vi "参数生成器.vi"() -> ()   [LabVIEW 2013]
uses:
  <vilib>/Utility/config.llb/Write Key (String).vi
  <vilib>/Utility/config.llb/Read Key (String).vi
  <vilib>/Utility/file.llb/Read From Spreadsheet File (string).vi
  <vilib>/Utility/config.llb/Write Key (Path).vi
  <vilib>/Utility/config.llb/NI_LVConfig.lvlib
panel:
  in  "均衡参数设置":bool
  in  "error in":errorcluster caption="错误输入"
  out "临时从板数据":string[](array[string])
  in  "自动记录":bool
  in  "通道电压清零":bool
  in  "自动计算通道电压":bool
  out "均衡参数":T1={"充电结束电压(90%)"=3.0, "充电结束电压(91%)"=3.0, "充电结束电压(92%)"=3.0, "充电结束电压(93%)"=3.0, "充电结束电压(94%)"=3.0, "均衡计算-电压高阀值1级"=3.0, "均衡计算-电压高阀值2级"=3.0, "均衡计算-电压低阀值1级"=3.0, "均衡计算-电压低阀值2级"=3.0, "均衡计算-最低电压阀值"=3.0, "均衡停止-最低电压阀值"=3.0, "均衡计算-电压极差阀值"=3.0, "充电结束电压(95%)"=3.0, "充电结束电压(96%)"=3.0, "充电结束电压(97%)"=3.0, "充电结束电压(98%)"=3.0, "充电结束电压(99%)"=3.0, "充电结束电压(100%)"=3.0} {"充电结束电压(100%)" min=0 max=5 format="%#.4f"; "充电结束电压(99%)" min=0 max=5 format="%#.4f"; "充电结束电压(98%)" min=0 max=5 format="%#.4f"; "充电结束电压(97%)" min=0 max=5 format="%#.4f"; "充电结束电压(96%)" min=0 max=5 format="%#.4f"; "充电结束电压(95%)" min=0 max=5 format="%#.4f"; "均衡计算-电压极差阀值" min=0 max=5 format="%#.4f"; "均衡停止-最低电压阀值" min=0 max=5 format="%#.4f"; "均衡计算-最低电压阀值" min=0 max=5 format="%#.4f"; "均衡计算-电压低阀值2级" min=0 max=5 format="%#.4f"; "充电结束电压(94%)" min=0 max=5 format="%#.4f"; "充电结束电压(93%)" min=0 max=5 format="%#.4f"; "均衡计算-电压低阀值1级" min=0 max=5 format="%#.4f"; "均衡计算-电压高阀值1级" min=0 max=5 format="%#.4f"; "均衡计算-电压高阀值2级" min=0 max=5 format="%#.4f"; "充电结束电压(92%)" min=0 max=5 format="%#.4f"; "充电结束电压(91%)" min=0 max=5 format="%#.4f"; "充电结束电压(90%)" min=0 max=5 format="%#.4f"}
  in  "布尔":bool
  in  "全部记录":bool
  in  "查看":bool
  in  "读从板信息":bool
  in  "字符串":string
  out "MD5 message-digest":string="c47cafb9475eca419ba2638971991389" caption="MD5信息摘要"
  out "从板表头":string[](array[string])=["从板板号", "电压个数", "电压起始值", "温度个数", "温度起始值", "第一个保险通道", "第一个保险位置", "第二个保险通道", "第二个保险位置", "第三个保险通道", "第三个保险位置", "第四个保险通道", "第四个保险位置", "第五个保险通道", "第五个保险位置", "第六个保险通道", "第六个保险位置", "第七个保险通道", "第七个保险位置", "第八个保险通道", "第八个保险位置", "第九个保险通道", "第九个保险位置", "第十个保险通道", "第十个保险位置", "第1通道电压个数", "第2通道电压个数", "第3通道电压个数", "第4通道电压个数", "第5通道电压个数", "第6通道电压个数", "第7通道电压个数", "第8通道电压个数", "第9通道电压个数", "第10通道电压个数", "第11通道电压个数", "第12通道电压个数", "第13通道电压个数", "第14通道电压个数", "第15通道电压个数", "第16通道电压个数", "第17通道电压个数", "第18通道电压个数", "第19通道电压个数", "第20通道电压个数", "风机开启温度", "风机关闭温度", "加热开启温度", "加热关闭温度", "风机开启温差", "风机关闭温差", "加热关闭温差", "电压过高一级", "电压过低一级", "温度过高一级", "温度过低一级", "电压不均衡一级", "温度不均衡一级", "SOC过低一级", "电压过高二级", "电压过低二级", "温度过高二级", "温度过低二级", "电压不均衡二级", "温度不均衡二级", "SOC过低二级", "电压过高三级", "电压过低三级", "温度过高三级", "温度过低三级", "电压不均衡三级", "温度不均衡三级", "SOC过低三级", "均衡计算-电压高阀值1级", "均衡计算-电压高阀值2级", "均衡计算-电压低阀值1级", "均衡计算-电压低阀值2级", "均衡计算-最低电压阀值", "均衡停止-最低电压阀值", "均衡计算-电压极差阀值", "充电结束电压(90%)", "充电结束电压(91%)", "充电结束电压(92%)", "充电结束电压(93%)", "充电结束电压(94%)", "充电结束电压(95%)", "充电结束电压(96%)", "充电结束电压(97%)", "充电结束电压(98%)", "充电结束电压(99%)", "充电结束电压(100%)"]
  out "输出数组":string[][](array[string])=[["1", "2", "3", " ", " ", " ", " ", " ", " ", " ", " ", " ", " ", " ", " ", " ", " ", " ", " ", " ", " ", " ", " ", " ", " ", " ", " ", " ", " ", " "], ["10", "10", "10", " ", " ", " ", " ", " ", " ", " ", " ", " ", " ", " ", " ", " ", " ", " ", " ", " ", " ", " ", " ", " ", " ", " ", " ", " ", " ", " "], ["", "0", "0", " ", " ", " ", " ", " ", " ", " ", " ", " ", " ", " ", " ", " ", " ", " ", " ", " ", " ", " ", " ", " ", " ", " ", " ", " ", " ", " "], ["2", "2", "2", " ", " ", " ", " ", " ", " ", " ", " ", " ", " ", " ", " ", " ", " ", " ", " ", " ", " ", " ", " ", " ", " ", " ", " ", " ", " ", " "], ["", "0", "0", " ", " ", " ", " ", " ", " ", " ", " ", " ", " ", " ", " ", " ", " ", " ", " ", " ", " ", " ", " ", " ", " ", " ", " ", " ", " ", " "], [" ", " ", " ", " ", " ", " ", " ", " ", " ", " ", " ", " ", " ", " ", " ", " ", " ", " ", " ", " ", " ", " ", " ", " ", " ", " ", " ", " ", " ", " "], [" ", " ", " ", " ", " ", " ", " ", " ", " ", " ", " ", " ", " ", " ", " ", " ", " ", " ", " ", " ", " ", " ", " ", " ", " ", " ", " ", " ", " ", " "], [" ", " ", " ", " ", " ", " ", " ", " ", " ", " ", " ", " ", " ", " ", " ", " ", " ", " ", " ", " ", " ", " ", " ", " ", " ", " ", " ", " ", " ", " "], [" ", " ", " ", " ", " ", " ", " ", " ", " ", " ", " ", " ", " ", " ", " ", " ", " ", " ", " ", " ", " ", " ", " ", " ", " ", " ", " ", " ", " ", " "], [" ", " ", " ", " ", " ", " ", " ", " ", " ", " ", " ", " ", " ", " ", " ", " ", " ", " ", " ", " ", " ", " ", " ", " ", " ", " ", " ", " ", " ", " "], [" ", " ", " ", " ", " ", " ", " ", " ", " ", " ", " ", " ", " ", " ", " ", " ", " ", " ", " ", " ", " ", " ", " ", " ", " ", " ", " ", " ", " ", " "], [" ", " ", " ", " ", " ", " ", " ", " ", " ", " ", " ", " ", " ", " ", " ", " ", " ", " ", " ", " ", " ", " ", " ", " ", " ", " ", " ", " ", " ", " "], [" ", " ", " ", " ", " ", " ", " ", " ", " ", " ", " ", " ", " ", " ", " ", " ", " ", " ", " ", " ", " ", " ", " ", " ", " ", " ", " ", " ", " ", " "], [" ", " ", " ", " ", " ", " ", " ", " ", " ", " ", " ", " ", " ", " ", " ", " ", " ", " ", " ", " ", " ", " ", " ", " ", " ", " ", " ", " ", " ", " "], [" ", " ", " ", " ", " ", " ", " ", " ", " ", " ", " ", " ", " ", " ", " ", " ", " ", " ", " ", " ", " ", " ", " ", " ", " ", " ", " ", " ", " ", " "], [" ", " ", " ", " ", " ", " ", " ", " ", " ", " ", " ", " ", " ", " ", " ", " ", " ", " ", " ", " ", " ", " ", " ", " ", " ", " ", " ", " ", " ", " "], [" ", " ", " ", " ", " ", " ", " ", " ", " ", " ", " ", " ", " ", " ", " ", " ", " ", " ", " ", " ", " ", " ", " ", " ", " ", " ", " ", " ", " ", " "], [" ", " ", " ", " ", " ", " ", " ", " ", " ", " ", " ", " ", " ", " ", " ", " ", " ", " ", " ", " ", " ", " ", " ", " ", " ", " ", " ", " ", " ", " "], [" ", " ", " ", " ", " ", " ", " ", " ", " ", " ", " ", " ", " ", " ", " ", " ", " ", " ", " ", " ", " ", " ", " ", " ", " ", " ", " ", " ", " ", " "], [" ", " ", " ", " ", " ", " ", " ", " ", " ", " ", " ", " ", " ", " ", " ", " ", " ", " ", " ", " ", " ", " ", " ", " ", " ", " ", " ", " ", " ", " "], [" ", " ", " ", " ", " ", " ", " ", " ", " ", " ", " ", " ", " ", " ", " ", " ", " ", " ", " ", " ", " ", " ", " ", " ", " ", " ", " ", " ", " ", " "], [" ", " ", " ", " ", " ", " ", " ", " ", " ", " ", " ", " ", " ", " ", " ", " ", " ", " ", " ", " ", " ", " ", " ", " ", " ", " ", " ", " ", " ", " "], [" ", " ", " ", " ", " ", " ", " ", " ", " ", " ", " ", " ", " ", " ", " ", " ", " ", " ", " ", " ", " ", " ", " ", " ", " ", " ", " ", " ", " ", " "], [" ", " ", " ", " ", " ", " ", " ", " ", " ", " ", " ", " ", " ", " ", " ", " ", " ", " ", " ", " ", " ", " ", " ", " ", " ", " ", " ", " ", " ", " "], [" ", " ", " ", " ", " ", " ", " ", " ", " ", " ", " ", " ", " ", " ", " ", " ", " ", " ", " ", " ", " ", " ", " ", " ", " ", " ", " ", " ", " ", " "], [" ", " ", " ", " ", " ", " ", " ", " ", " ", " ", " ", " ", " ", " ", " ", " ", " ", " ", " ", " ", " ", " ", " ", " ", " ", " ", " ", " ", " ", " "], [" ", " ", " ", " ", " ", " ", " ", " ", " ", " ", " ", " ", " ", " ", " ", " ", " ", " ", " ", " ", " ", " ", " ", " ", " ", " ", " ", " ", " ", " "], [" ", " ", " ", " ", " ", " ", " ", " ", " ", " ", " ", " ", " ", " ", " ", " ", " ", " ", " ", " ", " ", " ", " ", " ", " ", " ", " ", " ", " ", " "], [" ", " ", " ", " ", " ", " ", " ", " ", " ", " ", " ", " ", " ", " ", " ", " ", " ", " ", " ", " ", " ", " ", " ", " ", " ", " ", " ", " ", " ", " "], [" ", " ", " ", " ", " ", " ", " ", " ", " ", " ", " ", " ", " ", " ", " ", " ", " ", " ", " ", " ", " ", " ", " ", " ", " ", " ", " ", " ", " ", " "], [" ", " ", " ", " ", " ", " ", " ", " ", " ", " ", " ", " ", " ", " ", " ", " ", " ", " ", " ", " ", " ", " ", " ", " ", " ", " ", " ", " ", " ", " "], [" ", " ", " ", " ", " ", " ", " ", " ", " ", " ", " ", " ", " ", " ", " ", " ", " ", " ", " ", " ", " ", " ", " ", " ", " ", " ", " ", " ", " ", " "], [" ", " ", " ", " ", " ", " ", " ", " ", " ", " ", " ", " ", " ", " ", " ", " ", " ", " ", " ", " ", " ", " ", " ", " ", " ", " ", " ", " ", " ", " "], [" ", " ", " ", " ", " ", " ", " ", " ", " ", " ", " ", " ", " ", " ", " ", " ", " ", " ", " ", " ", " ", " ", " ", " ", " ", " ", " ", " ", " ", " "], [" ", " ", " ", " ", " ", " ", " ", " ", " ", " ", " ", " ", " ", " ", " ", " ", " ", " ", " ", " ", " ", " ", " ", " ", " ", " ", " ", " ", " ", " "], [" ", " ", " ", " ", " ", " ", " ", " ", " ", " ", " ", " ", " ", " ", " ", " ", " ", " ", " ", " ", " ", " ", " ", " ", " ", " ", " ", " ", " ", " "], [" ", " ", " ", " ", " ", " ", " ", " ", " ", " ", " ", " ", " ", " ", " ", " ", " ", " ", " ", " ", " ", " ", " ", " ", " ", " ", " ", " ", " ", " "], [" ", " ", " ", " ", " ", " ", " ", " ", " ", " ", " ", " ", " ", " ", " ", " ", " ", " ", " ", " ", " ", " ", " ", " ", " ", " ", " ", " ", " ", " "], [" ", " ", " ", " ", " ", " ", " ", " ", " ", " ", " ", " ", " ", " ", " ", " ", " ", " ", " ", " ", " ", " ", " ", " ", " ", " ", " ", " ", " ", " "], [" ", " ", " ", " ", " ", " ", " ", " ", " ", " ", " ", " ", " ", " ", " ", " ", " ", " ", " ", " ", " ", " ", " ", " ", " ", " ", " ", " ", " ", " "], [" ", " ", " ", " ", " ", " ", " ", " ", " ", " ", " ", " ", " ", " ", " ", " ", " ", " ", " ", " ", " ", " ", " ", " ", " ", " ", " ", " ", " ", " "], [" ", " ", " ", " ", " ", " ", " ", " ", " ", " ", " ", " ", " ", " ", " ", " ", " ", " ", " ", " ", " ", " ", " ", " ", " ", " ", " ", " ", " ", " "], [" ", " ", " ", " ", " ", " ", " ", " ", " ", " ", " ", " ", " ", " ", " ", " ", " ", " ", " ", " ", " ", " ", " ", " ", " ", " ", " ", " ", " ", " "], [" ", " ", " ", " ", " ", " ", " ", " ", " ", " ", " ", " ", " ", " ", " ", " ", " ", " ", " ", " ", " ", " ", " ", " ", " ", " ", " ", " ", " ", " "], [" ", " ", " ", " ", " ", " ", " ", " ", " ", " ", " ", " ", " ", " ", " ", " ", " ", " ", " ", " ", " ", " ", " ", " ", " ", " ", " ", " ", " ", " "], ["35", "35", "35", " ", " ", " ", " ", " ", " ", " ", " ", " ", " ", " ", " ", " ", " ", " ", " ", " ", " ", " ", " ", " ", " ", " ", " ", " ", " ", " "], ["30", "30", "30", " ", " ", " ", " ", " ", " ", " ", " ", " ", " ", " ", " ", " ", " ", " ", " ", " ", " ", " ", " ", " ", " ", " ", " ", " ", " ", " "], ["0", "0", "0", " ", " ", " ", " ", " ", " ", " ", " ", " ", " ", " ", " ", " ", " ", " ", " ", " ", " ", " ", " ", " ", " ", " ", " ", " ", " ", " "], ["5", "5", "5", " ", " ", " ", " ", " ", " ", " ", " ", " ", " ", " ", " ", " ", " ", " ", " ", " ", " ", " ", " ", " ", " ", " ", " ", " ", " ", " "], ["5", "5", "5", " ", " ", " ", " ", " ", " ", " ", " ", " ", " ", " ", " ", " ", " ", " ", " ", " ", " ", " ", " ", " ", " ", " ", " ", " ", " ", " "], ["3", "3", "3", " ", " ", " ", " ", " ", " ", " ", " ", " ", " ", " ", " ", " ", " ", " ", " ", " ", " ", " ", " ", " ", " ", " ", " ", " ", " ", " "], ["10", "10", "10", " ", " ", " ", " ", " ", " ", " ", " ", " ", " ", " ", " ", " ", " ", " ", " ", " ", " ", " ", " ", " ", " ", " ", " ", " ", " ", " "], ["4.23", "4.23", "4.23", " ", " ", " ", " ", " ", " ", " ", " ", " ", " ", " ", " ", " ", " ", " ", " ", " ", " ", " ", " ", " ", " ", " ", " ", " ", " ", " "], ["3", "3", "3", " ", " ", " ", " ", " ", " ", " ", " ", " ", " ", " ", " ", " ", " ", " ", " ", " ", " ", " ", " ", " ", " ", " ", " ", " ", " ", " "], ["50", "50", "50", " ", " ", " ", " ", " ", " ", " ", " ", " ", " ", " ", " ", " ", " ", " ", " ", " ", " ", " ", " ", " ", " ", " ", " ", " ", " ", " "], ["-20", "-20", "-20", " ", " ", " ", " ", " ", " ", " ", " ", " ", " ", " ", " ", " ", " ", " ", " ", " ", " ", " ", " ", " ", " ", " ", " ", " ", " ", " "], ["0.5", "0.5", "0.5", " ", " ", " ", " ", " ", " ", " ", " ", " ", " ", " ", " ", " ", " ", " ", " ", " ", " ", " ", " ", " ", " ", " ", " ", " ", " ", " "], ["25", "25", "25", " ", " ", " ", " ", " ", " ", " ", " ", " ", " ", " ", " ", " ", " ", " ", " ", " ", " ", " ", " ", " ", " ", " ", " ", " ", " ", " "], ["30", "30", "30", " ", " ", " ", " ", " ", " ", " ", " ", " ", " ", " ", " ", " ", " ", " ", " ", " ", " ", " ", " ", " ", " ", " ", " ", " ", " ", " "], ["4.25", "4.25", "4.25", " ", " ", " ", " ", " ", " ", " ", " ", " ", " ", " ", " ", " ", " ", " ", " ", " ", " ", " ", " ", " ", " ", " ", " ", " ", " ", " "], ["2.75", "2.75", "2.75", " ", " ", " ", " ", " ", " ", " ", " ", " ", " ", " ", " ", " ", " ", " ", " ", " ", " ", " ", " ", " ", " ", " ", " ", " ", " ", " "], ["55", "55", "55", " ", " ", " ", " ", " ", " ", " ", " ", " ", " ", " ", " ", " ", " ", " ", " ", " ", " ", " ", " ", " ", " ", " ", " ", " ", " ", " "], ["-30", "-30", "-30", " ", " ", " ", " ", " ", " ", " ", " ", " ", " ", " ", " ", " ", " ", " ", " ", " ", " ", " ", " ", " ", " ", " ", " ", " ", " ", " "], ["1", "1", "1", " ", " ", " ", " ", " ", " ", " ", " ", " ", " ", " ", " ", " ", " ", " ", " ", " ", " ", " ", " ", " ", " ", " ", " ", " ", " ", " "], ["30", "30", "30", " ", " ", " ", " ", " ", " ", " ", " ", " ", " ", " ", " ", " ", " ", " ", " ", " ", " ", " ", " ", " ", " ", " ", " ", " ", " ", " "], ["20", "20", "20", " ", " ", " ", " ", " ", " ", " ", " ", " ", " ", " ", " ", " ", " ", " ", " ", " ", " ", " ", " ", " ", " ", " ", " ", " ", " ", " "], ["4.3", "4.3", "4.3", " ", " ", " ", " ", " ", " ", " ", " ", " ", " ", " ", " ", " ", " ", " ", " ", " ", " ", " ", " ", " ", " ", " ", " ", " ", " ", " "], ["2.5", "2.5", "2.5", " ", " ", " ", " ", " ", " ", " ", " ", " ", " ", " ", " ", " ", " ", " ", " ", " ", " ", " ", " ", " ", " ", " ", " ", " ", " ", " "], ["60", "60", "60", " ", " ", " ", " ", " ", " ", " ", " ", " ", " ", " ", " ", " ", " ", " ", " ", " ", " ", " ", " ", " ", " ", " ", " ", " ", " ", " "], ["-40", "-40", "-40", " ", " ", " ", " ", " ", " ", " ", " ", " ", " ", " ", " ", " ", " ", " ", " ", " ", " ", " ", " ", " ", " ", " ", " ", " ", " ", " "], ["1.5", "1.5", "1.5", " ", " ", " ", " ", " ", " ", " ", " ", " ", " ", " ", " ", " ", " ", " ", " ", " ", " ", " ", " ", " ", " ", " ", " ", " ", " ", " "], ["35", "35", "35", " ", " ", " ", " ", " ", " ", " ", " ", " ", " ", " ", " ", " ", " ", " ", " ", " ", " ", " ", " ", " ", " ", " ", " ", " ", " ", " "], ["10", "10", "10", " ", " ", " ", " ", " ", " ", " ", " ", " ", " ", " ", " ", " ", " ", " ", " ", " ", " ", " ", " ", " ", " ", " ", " ", " ", " ", " "], ["3", "4.23", "4.23", " ", " ", " ", " ", " ", " ", " ", " ", " ", " ", " ", " ", " ", " ", " ", " ", " ", " ", " ", " ", " ", " ", " ", " ", " ", " ", " "], ["3", "3", "3", " ", " ", " ", " ", " ", " ", " ", " ", " ", " ", " ", " ", " ", " ", " ", " ", " ", " ", " ", " ", " ", " ", " ", " ", " ", " ", " "], ["3", "50", "50", " ", " ", " ", " ", " ", " ", " ", " ", " ", " ", " ", " ", " ", " ", " ", " ", " ", " ", " ", " ", " ", " ", " ", " ", " ", " ", " "], ["3", "-20", "-20", " ", " ", " ", " ", " ", " ", " ", " ", " ", " ", " ", " ", " ", " ", " ", " ", " ", " ", " ", " ", " ", " ", " ", " ", " ", " ", " "], ["3", "0.5", "0.5", " ", " ", " ", " ", " ", " ", " ", " ", " ", " ", " ", " ", " ", " ", " ", " ", " ", " ", " ", " ", " ", " ", " ", " ", " ", " ", " "], ["3", "25", "25", " ", " ", " ", " ", " ", " ", " ", " ", " ", " ", " ", " ", " ", " ", " ", " ", " ", " ", " ", " ", " ", " ", " ", " ", " ", " ", " "], ["3", "30", "30", " ", " ", " ", " ", " ", " ", " ", " ", " ", " ", " ", " ", " ", " ", " ", " ", " ", " ", " ", " ", " ", " ", " ", " ", " ", " ", " "], ["3", "4.25", "4.25", " ", " ", " ", " ", " ", " ", " ", " ", " ", " ", " ", " ", " ", " ", " ", " ", " ", " ", " ", " ", " ", " ", " ", " ", " ", " ", " "], ["3", "2.75", "2.75", " ", " ", " ", " ", " ", " ", " ", " ", " ", " ", " ", " ", " ", " ", " ", " ", " ", " ", " ", " ", " ", " ", " ", " ", " ", " ", " "], ["3", "55", "55", " ", " ", " ", " ", " ", " ", " ", " ", " ", " ", " ", " ", " ", " ", " ", " ", " ", " ", " ", " ", " ", " ", " ", " ", " ", " ", " "], ["3", "-30", "-30", " ", " ", " ", " ", " ", " ", " ", " ", " ", " ", " ", " ", " ", " ", " ", " ", " ", " ", " ", " ", " ", " ", " ", " ", " ", " ", " "], ["3", "1", "1", " ", " ", " ", " ", " ", " ", " ", " ", " ", " ", " ", " ", " ", " ", " ", " ", " ", " ", " ", " ", " ", " ", " ", " ", " ", " ", " "], ["3", "30", "30", " ", " ", " ", " ", " ", " ", " ", " ", " ", " ", " ", " ", " ", " ", " ", " ", " ", " ", " ", " ", " ", " ", " ", " ", " ", " ", " "], ["3", "20", "20", " ", " ", " ", " ", " ", " ", " ", " ", " ", " ", " ", " ", " ", " ", " ", " ", " ", " ", " ", " ", " ", " ", " ", " ", " ", " ", " "], ["3", "4.3", "4.3", " ", " ", " ", " ", " ", " ", " ", " ", " ", " ", " ", " ", " ", " ", " ", " ", " ", " ", " ", " ", " ", " ", " ", " ", " ", " ", " "], ["3", "2.5", "2.5", " ", " ", " ", " ", " ", " ", " ", " ", " ", " ", " ", " ", " ", " ", " ", " ", " ", " ", " ", " ", " ", " ", " ", " ", " ", " ", " "], ["3", "60", "60", " ", " ", " ", " ", " ", " ", " ", " ", " ", " ", " ", " ", " ", " ", " ", " ", " ", " ", " ", " ", " ", " ", " ", " ", " ", " ", " "], ["3", "-40", "-40", " ", " ", " ", " ", " ", " ", " ", " ", " ", " ", " ", " ", " ", " ", " ", " ", " ", " ", " ", " ", " ", " ", " ", " ", " ", " ", " "], [" ", "1.5", "1.5", " ", " ", " ", " ", " ", " ", " ", " ", " ", " ", " ", " ", " ", " ", " ", " ", " ", " ", " ", " ", " ", " ", " ", " ", " ", " ", " "], [" ", "35", "35", " ", " ", " ", " ", " ", " ", " ", " ", " ", " ", " ", " ", " ", " ", " ", " ", " ", " ", " ", " ", " ", " ", " ", " ", " ", " ", " "], [" ", "10", "10", " ", " ", " ", " ", " ", " ", " ", " ", " ", " ", " ", " ", " ", " ", " ", " ", " ", " ", " ", " ", " ", " ", " ", " ", " ", " ", " "], [" ", "3", "4.23", " ", " ", " ", " ", " ", " ", " ", " ", " ", " ", " ", " ", " ", " ", " ", " ", " ", " ", " ", " ", " ", " ", " ", " ", " ", " ", " "], [" ", "3", "3", " ", " ", " ", " ", " ", " ", " ", " ", " ", " ", " ", " ", " ", " ", " ", " ", " ", " ", " ", " ", " ", " ", " ", " ", " ", " ", " "], [" ", "3", "50", " ", " ", " ", " ", " ", " ", " ", " ", " ", " ", " ", " ", " ", " ", " ", " ", " ", " ", " ", " ", " ", " ", " ", " ", " ", " ", " "], [" ", "3", "-20", " ", " ", " ", " ", " ", " ", " ", " ", " ", " ", " ", " ", " ", " ", " ", " ", " ", " ", " ", " ", " ", " ", " ", " ", " ", " ", " "], [" ", "3", "0.5", " ", " ", " ", " ", " ", " ", " ", " ", " ", " ", " ", " ", " ", " ", " ", " ", " ", " ", " ", " ", " ", " ", " ", " ", " ", " ", " "], [" ", "3", "25", " ", " ", " ", " ", " ", " ", " ", " ", " ", " ", " ", " ", " ", " ", " ", " ", " ", " ", " ", " ", " ", " ", " ", " ", " ", " ", " "]]
  in  "退出":bool
  in  "工程代号":string="B32615"
  in  "选项卡控件":enum32{"主板", "从板", "预览"}(tab)=enum."从板"
  in  "分流器型号":T2(ring)=enum."300A"
  in  "全部清零(主板)":bool
  in  "默认值":bool
  in  "读主板参数":bool
  in  "加热控制参数":T3={"风机开启温度(℃)"=30.0, "风机关闭温度(℃)"=20.0, "加热开启温度(℃)"=10.0, "加热关闭温度(℃)"=15.0, "风机开启温差(℃)"=5.0, "风机关闭温差(℃)"=3.0, "加热关闭温差(℃)"=10.0}
  in  "设电池信息主板":bool
  in  "电池信息":string[][](table)=[["电池串联", "92"], ["电池并联", "2"], ["电池包额定容量", "67"], ["电池包额定能量", "0"], ["电池包额定总电压", "340"], ["实际容量", "67"], ["电池厂家", "普莱德"], ["电池类型", "磷酸铁锂"], ["电池生产日期", "2013-12-11 11:34:30"], ["电池包组号", "0"], ["累计充电总安时", "0"], ["累计放电总安时", "0"], ["电池放空次数", "0"], ["电池充满次数", "0"], ["电池充电次数", "0"]]
  in  "一级故障":dbl[][](array[numeric])=[[389.0, 391.0, 395.0], [276.0, 253.0, 230.0], [50.0, 55.0, 60.0], [-20.0, -30.0, -40.0], [0.5, 1.0, 1.5], [0.5, 1.0, 1.5], [25.0, 30.0, 35.0], [25.0, 30.0, 35.0], [4.23, 4.25, 4.3], [3.0, 2.75, 2.5], [110.0, 132.0, 165.0], [250.0, 270.0, 300.0], [101.0, 101.0, 101.0], [30.0, 20.0, 10.0], [3.0, 5.0, 10.0], [50.0, 55.0, 60.0], [90.0, 80.0, 70.0]]
  in  "从板个数":dbl=3.0
  in  "主板信息":string[][](table)=[["电池额定容量", "0"], ["电池实际容量", "0"], ["SOC", "0"], ["SOH", "0"], ["产品编号", ""], ["车架(牌)号", ""], ["配置文件版本", ""], ["从板1电池节数", "10"], ["从板2电池节数", "10"], ["从板3电池节数", "10"], ["从板1温度个数", "2"], ["从板2温度个数", "2"], ["从板3温度个数", "2"]]
  in  "单个写入":bool
  in  "充电控制参数":T4={"最大允许单体电压(V)"=4.15, "最大允许总电压(V)"=382.0, "最小允许单体电压(V)"=2.75, "最大允许充电电流(A)"=50.0, "最小允许充电电流(A)"=3.0, "最大允许充电温度(℃)"=55.0, "最小允许充电温度(℃)"=-15.0, "电流步长"=5.0}
  in  "温度个数":dbl
  in  "电压个数":dbl
  in  "粘贴":bool
  in  "复制":T5
  in  "保险位置清零":bool
  in  "5个通道电压个数(最小5个)":u8[](array[numeric])=[0, 0, 0, 0, 0, 0, 0, 0, 0, 0, 0, 0, 0, 0, 0, 0, 0, 0, 0, 0] max=12
  in  "保险位置":T6
  in  "全部清零(从板)":bool
  in  "读从板参数":bool
  in  "从板板号":dbl=1.0 min=1.0 max=3.0 step=1.0
  in  "从板信息电压温度通道配置":string[][](table)=[["电压个数", "10"], ["电压起始值", ""], ["温度个数", "2"], ["温度起始值", ""], ["第一个保险通道", " "], ["第一个保险位置", " "], ["第二个保险通道", " "], ["第二个保险位置", " "], ["第三个保险通道", " "], ["第三个保险位置", " "], ["第四个保险通道", " "], ["第四个保险位置", " "], ["第五个保险通道", " "], ["第五个保险位置", " "], ["第六个保险通道", " "], ["第六个保险位置", " "], ["第七个保险通道", " "], ["第七个保险位置", " "], ["第八个保险通道", " "], ["第八个保险位置", " "], ["第九个保险通道", " "], ["第九个保险位置", " "], ["第十个保险通道", " "], ["第十个保险位置", " "], ["第1通道电压个数", " "], ["第2通道电压个数", " "], ["第3通道电压个数", " "], ["第4通道电压个数", " "], ["第5通道电压个数", " "], ["", " "], ["", " "], ["", " "], ["", " "], ["", " "], ["", " "], ["", " "], ["", " "], ["", " "], ["", " "], ["", " "], ["", " "], ["", " "], ["", " "], ["", " "]]
  in  "默认值 2":bool
  out "结果":i32(listbox)=-1
  in  "保存当前从板配置":T5
  in  "一级故障 2":dbl[][](array[numeric])=[[4.23, 4.25, 4.3], [3.0, 2.75, 2.5], [50.0, 55.0, 60.0], [-20.0, -30.0, -40.0], [0.5, 1.0, 1.5], [25.0, 30.0, 35.0], [30.0, 20.0, 10.0]] caption="一级故障"
  in  "加热控制参数 2":T3={"风机开启温度(℃)"=35.0, "风机关闭温度(℃)"=30.0, "加热开启温度(℃)"=0.0, "加热关闭温度(℃)"=5.0, "风机开启温差(℃)"=5.0, "风机关闭温差(℃)"=3.0, "加热关闭温差(℃)"=10.0}
  in  "主从板":enum32{"单选选项2", "单选选项1"}(radio)
  in  "读取(ini)":bool
  in  "预览":bool
  in  "工号":string="123"
  in  "写配置文件":bool
  # "操作说明 \n1） 输入从板1参数\n2） 完成后点“记录”\n3） 把参数更改成从板2参数\n4） 再点击“记录”\n5） 以此类推，直到完成所有从板"
  # "参数设置上位机"
  # "Step7->"
  # "<-Step3"
  # "Step2->"
  # "每个项目需要确认6个步骤都设置正确!"
  # "二级故障"
  # "三级故障"
  # "总电压过高(V)"
  # "Step1->"
  # "总电压过低(V)"
  # "温度过高(℃)"
  # "温度过低(℃)"
  # "<-Step4"
  # "整组电压不均衡(V)"
  # "单组电压不均衡(V)"
  # "整组温度不均衡(V)"
  # "单组温度不均衡(V)"
  # "单体电压过高(V)"
  # "单体电压过低(V)"
  # "<-Step5"
  # "充电电流过高(A)"
  # "Step6->"
  # "放电电流过高(A)"
  # "SOC过高(%)"
  # "SOC过低(%)"
  # "内阻过大(mΩ)"
  # "极柱温度过高(℃)"
  # "SOH过低(%)"
  # "Step1->"
  # "Step2->"
  # "1"
  # "2"
  # "3"
  # "4"
  # "5"
  # "Step3->"
  # "Step4->"
  # "Step5->"
  # "Step6->"
  # "1"
  # "2"
  # "3"
  # "7"
  # "4"
  # "5"
  # "6"
  # "8"
  # "9"
  # "10"
  # "11"
  # "12"
  # "通道1"
  # "通道2"
  # "通道3"
  # "通道4"
  # "通道5"
  # "二级故障"
  # "三级故障"
  # "电压过高(V)"
  # "电压过低(V)"
  # "温度过高(℃)"
  # "温度过低(℃)"
  # "电压不均衡(V)"
  # "温度不均衡(℃)"
  # "SOC过低(%)"
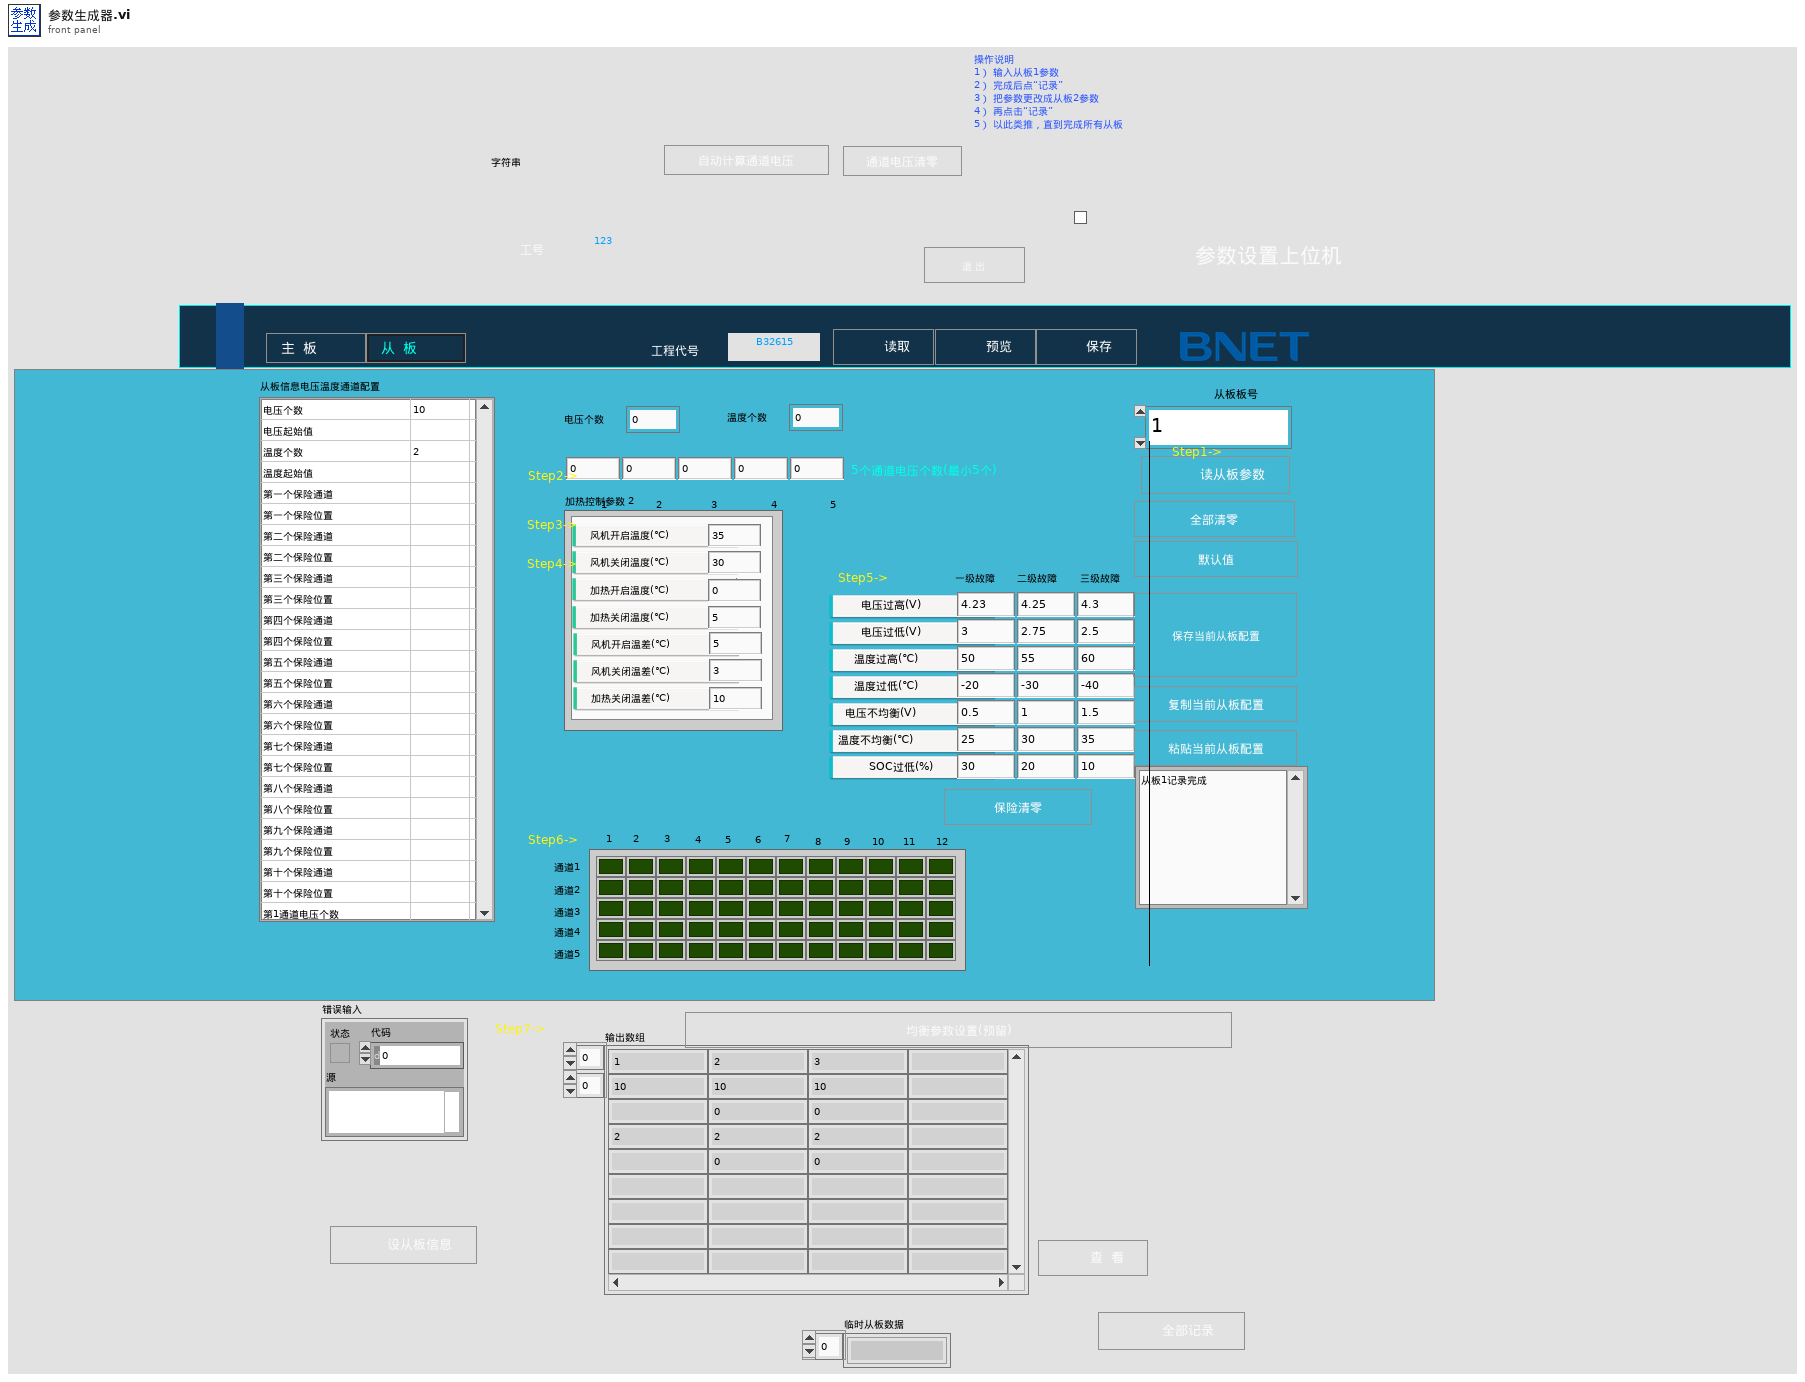
[diagram p1: front panel]
types:
  T1 = cluster{"充电结束电压(90%)":sgl, "充电结束电压(91%)":sgl, "充电结束电压(92%)":sgl, "充电结束电压(93%)":sgl, "充电结束电压(94%)":sgl, "均衡计算-电压高阀值1级":sgl, "均衡计算-电压高阀值2级":sgl, "均衡计算-电压低阀值1级":sgl, "均衡计算-电压低阀值2级":sgl, "均衡计算-最低电压阀值":sgl, "均衡停止-最低电压阀值":sgl, "均衡计算-电压极差阀值":sgl, "充电结束电压(95%)":sgl, "充电结束电压(96%)":sgl, "充电结束电压(97%)":sgl, "充电结束电压(98%)":sgl, "充电结束电压(99%)":sgl, "充电结束电压(100%)":sgl}
  T2 = enum16{"选择分流器型号", "100A", "200A", "300A", "400A", "500A", "600A", "700A", "800A", "900A", "1000A"}
  T3 = cluster{"风机开启温度(℃)":dbl, "风机关闭温度(℃)":dbl, "加热开启温度(℃)":dbl, "加热关闭温度(℃)":dbl, "风机开启温差(℃)":dbl, "风机关闭温差(℃)":dbl, "加热关闭温差(℃)":dbl}
  T4 = cluster{"最大允许单体电压(V)":dbl, "最大允许总电压(V)":dbl, "最小允许单体电压(V)":dbl, "最大允许充电电流(A)":dbl, "最小允许充电电流(A)":dbl, "最大允许充电温度(℃)":dbl, "最小允许充电温度(℃)":dbl, "电流步长":dbl}
  T5 = typedef "button.ctl" = bool
  T6 = typedef "111.ctl" = T7[][]
  T7 = typedef "保险位置.ctl" = bool
  T8 = cluster{"风机开启温度(℃)":dbl, "风机关闭温度(℃)":dbl, "加热开启温度(℃)":dbl, "加热关闭温度(℃)":dbl, "风机开启温差(℃)":dbl, "风机开启温度(℃)":dbl, "加热关闭温差(℃)":dbl}
  T9 = cluster{"风机开启温度":dbl, "风机关闭温度":dbl, "加热开启温度":dbl, "加热关闭温度":dbl, "风机开启温差":dbl, "风机关闭温差":dbl, "加热关闭温差":dbl}
  T10 = cluster{"[0]":dbl, "[1]":dbl, "[2]":dbl, "[3]":dbl, "[4]":dbl, "[5]":dbl, "[6]":dbl}
  T11 = typedef "NI_LVConfig.lvlib/Config Data RefNum.ctl" = refnum<k1>
  T12 = cluster{"[0]":dbl, "[1]":dbl, "[2]":dbl, "[3]":dbl, "[4]":dbl, "[5]":dbl, "[6]":dbl, "[7]":dbl}
  T13 = cluster{"[0]":dbl, "[1]":dbl, "[2]":dbl, "[3]":dbl, "[4]":dbl, "[5]":dbl, "[6]":dbl, "[7]":dbl, "[8]":dbl, "[9]":dbl, "[10]":dbl, "[11]":dbl, "[12]":dbl, "[13]":dbl, "[14]":dbl, "[15]":dbl, "[16]":dbl, "[17]":dbl}
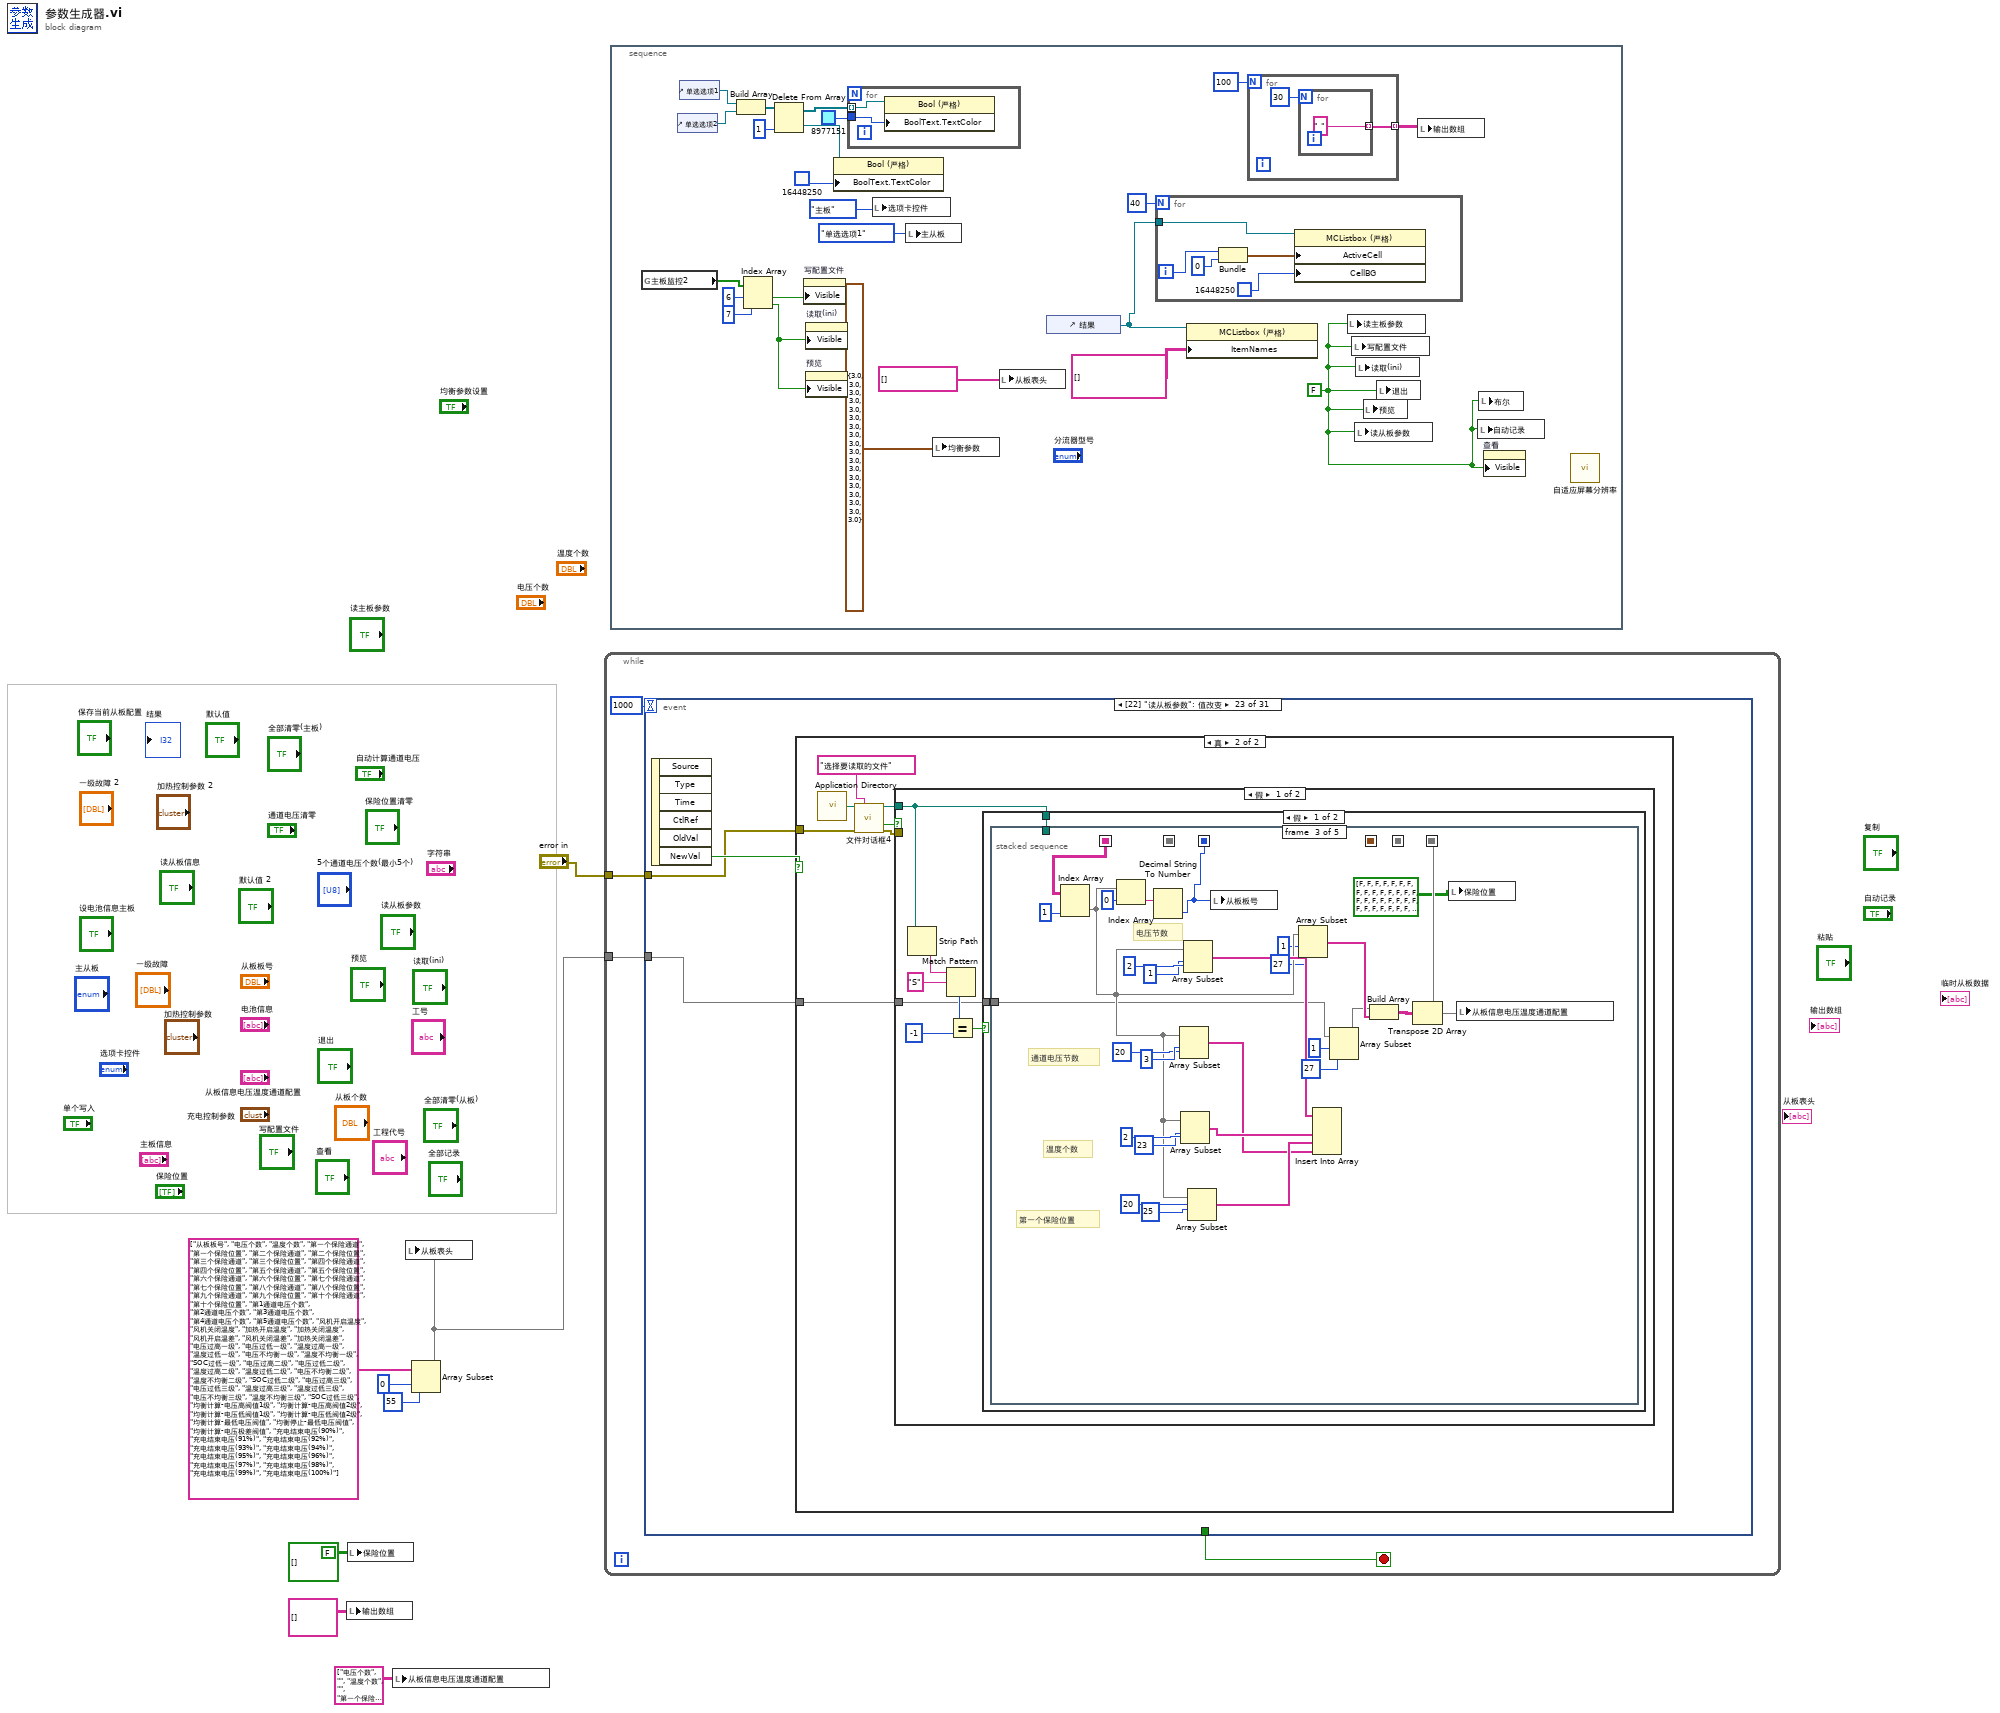
[diagram p0: block diagram]
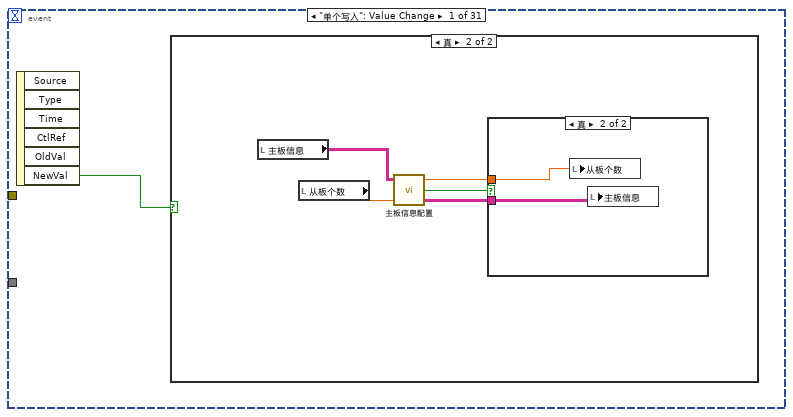
[diagram p2: hidden frame]
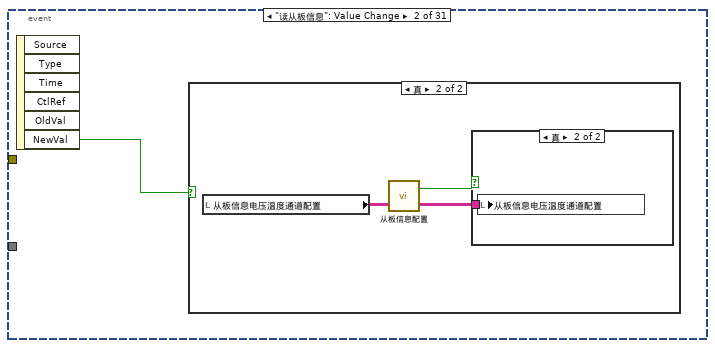
[diagram p5: hidden frame]
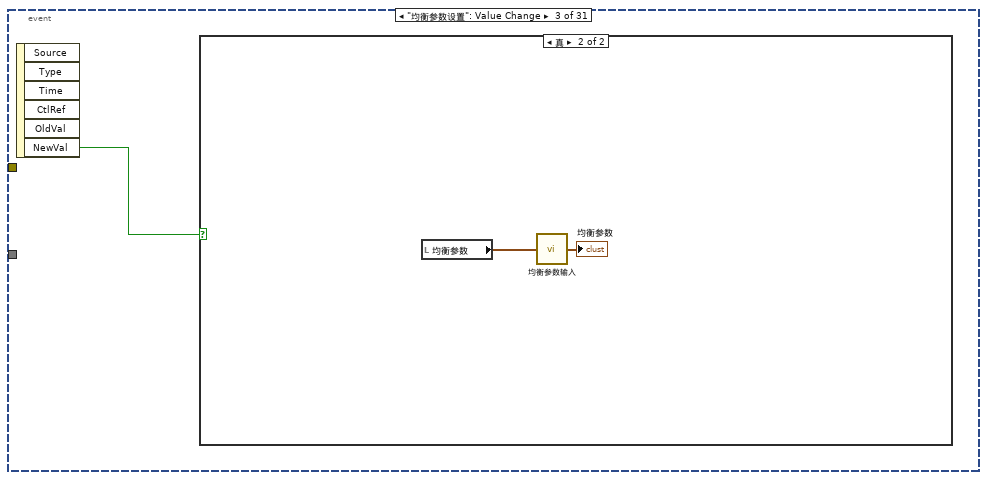
[diagram p8: hidden frame]
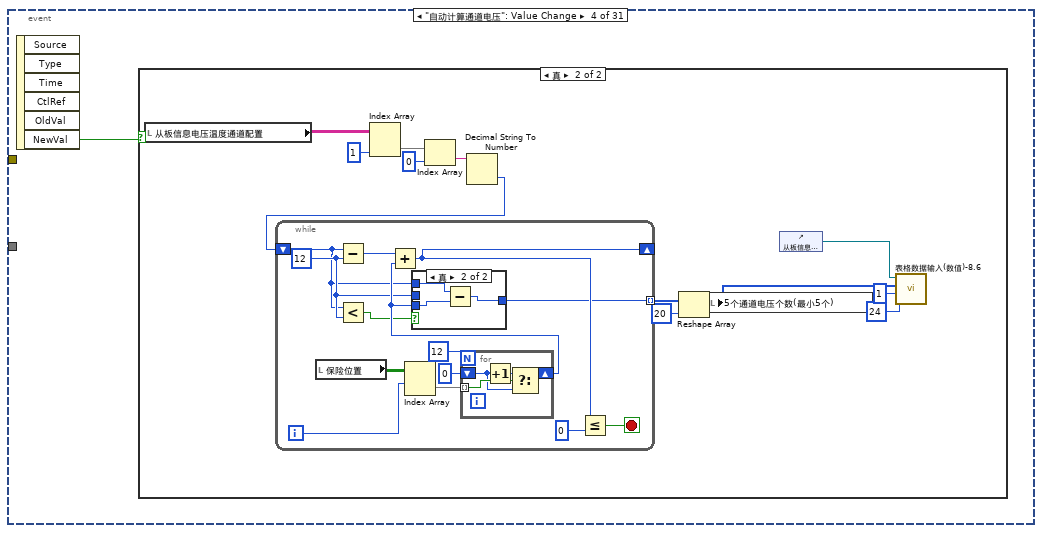
[diagram p10: hidden frame]
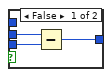
[diagram p12: hidden frame]
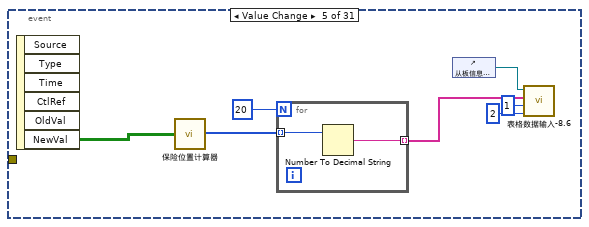
[diagram p13: hidden frame]
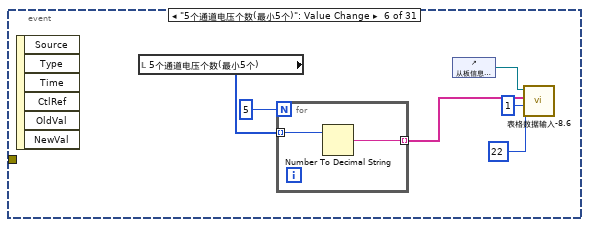
[diagram p14: hidden frame]
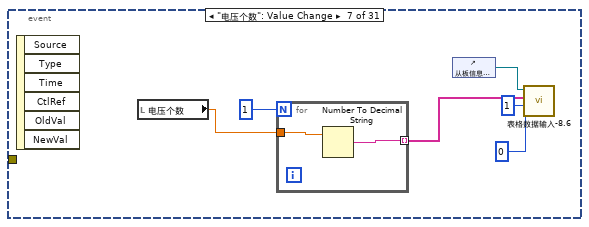
[diagram p15: hidden frame]
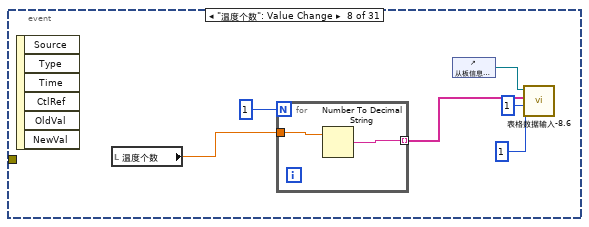
[diagram p16: hidden frame]
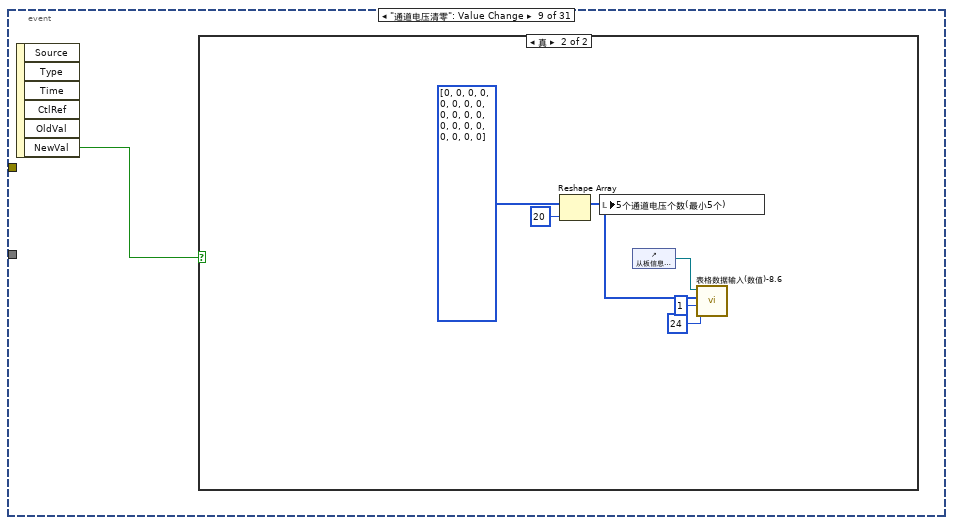
[diagram p17: hidden frame]
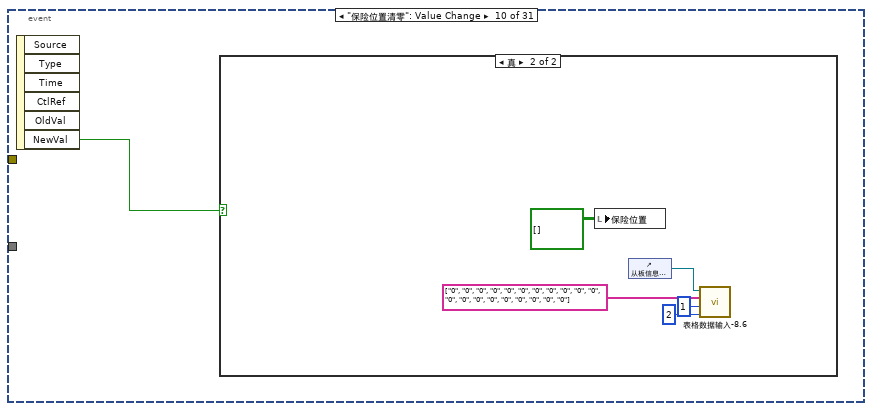
[diagram p19: hidden frame]
diagram:
  (unwired) T7 FALSE ("布尔")
  n1 = local write "输出数组"(string[][] [] ("输出数组")) -> ()
  n2 = local write "保险位置"(T6 [] ("保险位置")) -> ()
  n3 = local write "从板信息电压温度通道配置"(string[][] [["电压个数", ""], ["温度个数", ""], ["第一个保险通道", "0"], ["第一个保险位置", "0"], ["第二个保险通道", "0"], ["第二个保险位置", "0"], ["第三个保险通道", "0"], ["第三个保险位置", "0"], ["第四个保险通道", "0"], ["第四个保险位置", "0"], ["第五个保险通道", "0"], ["第五个保险位置", "0"], ["第六个保险通道", "0"], ["第六个保险位置", "0"], ["第七个保险通道", "0"], ["第七个保险位置", "0"], ["第八个保险通道", "0"], ["第八个保险位置", "0"], ["第九个保险通道", "0"], ["第九个保险位置", "0"], ["第十个保险通道", "0"], ["第十个保险位置", "0"], ["第1通道电压个数", ""], ["第2通道电压个数", ""], ["第3通道电压个数", ""], ["第4通道电压个数", ""], ["第5通道电压个数", ""]] ("从板信息电压温度通道配置")) -> ()
  n4 = Array Subset(array=string[] ["从板板号", "电压个数", "温度个数", "第一个保险通道", "第一个保险位置", "第二个保险通道", "第二个保险位置", "第三个保险通道", "第三个保险位置", "第四个保险通道", "第四个保险位置", "第五个保险通道", "第五个保险位置", "第六个保险通道", "第六个保险位置", "第七个保险通道", "第七个保险位置", "第八个保险通道", "第八个保险位置", "第九个保险通道", "第九个保险位置", "第十个保险通道", "第十个保险位置", "第1通道电压个数", "第2通道电压个数", "第3通道电压个数", "第4通道电压个数", "第5通道电压个数", "风机开启温度", "风机关闭温度", "加热开启温度", "加热关闭温度", "风机开启温差", "风机关闭温差", "加热关闭温差", "电压过高一级", "电压过低一级", "温度过高一级", "温度过低一级", "电压不均衡一级", "温度不均衡一级", "SOC过低一级", "电压过高二级", "电压过低二级", "温度过高二级", "温度过低二级", "电压不均衡二级", "温度不均衡二级", "SOC过低二级", "电压过高三级", "电压过低三级", "温度过高三级", "温度过低三级", "电压不均衡三级", "温度不均衡三级", "SOC过低三级", "均衡计算-电压高阀值1级", "均衡计算-电压高阀值2级", "均衡计算-电压低阀值1级", "均衡计算-电压低阀值2级", "均衡计算-最低电压阀值", "均衡停止-最低电压阀值", "均衡计算-电压极差阀值", "充电结束电压(90%)", "充电结束电压(91%)", "充电结束电压(92%)", "充电结束电压(93%)", "充电结束电压(94%)", "充电结束电压(95%)", "充电结束电压(96%)", "充电结束电压(97%)", "充电结束电压(98%)", "充电结束电压(99%)", "充电结束电压(100%)"] ("从板表头"), index=0 ("索引"), length=55 ("长度")) -> (w1:string[])
  n5 = local write "从板表头"(w1) -> ()
  n6 = while {
    tunnel: "error in" -> [w10]
    tunnel: w1 -> [w9]
    stop <- w12 stop-if-true
    n7 = event shown="[22] \"读从板参数\": 值改变" {
      selector: _ -> [_ _ _ _ _ _ _ _ _ _ _ _ _ _ _ _ _ _ _ _ _ _ _ _ _ _ _ _ _ _ _]
      dyn-events: _ -> [_ _ _ _ _ _ _ _ _ _ _ _ _ _ _ _ _ _ _ _ _ _ _ _ _ _ _ _ _ _ _]
      timeout: 1000 -> [_ _ _ _ _ _ _ _ _ _ _ _ _ _ _ _ _ _ _ _ _ _ _ _ _ _ _ _ _ _ _]
      tunnel: [_ _ _ _ _ _ _ _ _ _ _ _ _ _ _ _ _ _ _ _ _ _ _ _ _ _ TRUE TRUE _ _ _] -> w12
      tunnel: w10 -> [_ _ _ _ _ _ _ _ _ _ _ _ _ _ _ _ _ _ _ _ _ w977 w1163 _ _ _ _ _ _ _ _]
      tunnel: w9 -> [_ _ _ _ _ _ _ _ _ _ _ _ _ _ _ _ _ w534 _ _ _ _ w1162 _ _ _ _ _ _ _ _]
      event "单个写入": Value Change {
        n8 = event-data() -> ("NewVal"=w13:bool)  [unwired: 1 in, 5 out]
        n9 = case shown="真" w13 {
          frame False {
          }
          frame True {
            n10 = local read "主板信息"() -> (w15:string[][])
            n11 = local read "从板个数"() -> (w18:dbl)
            n12 = call "主板信息配置.vi"("从板个数"=w18, "主板信息查看"=w15) -> ("输出数组"=w17:string[][], "布尔"=w14:bool, "从板个数 2"=w16:dbl)  [unwired: 1 in]
            n13 = case shown="真" w14 {
              tunnel: w17 -> [_ w20]
              tunnel: w16 -> [_ w19]
              frame False {
              }
              frame True {
                n14 = local write "从板个数"(w19) -> ()
                n15 = local write "主板信息"(w20) -> ()
              }
            }
          }
        }
      }
      event "读从板信息": Value Change {
        n16 = event-data() -> ("NewVal"=w21:bool)  [unwired: 1 in, 5 out]
        n17 = case shown="真" w21 {
          frame False {
          }
          frame True {
            n18 = local read "从板信息电压温度通道配置"() -> (w23:string[][])
            n19 = call "从板信息配置.vi"("从板信息查看"=w23) -> ("输出数组"=w24:string[][], "布尔"=w22:bool)  [unwired: 1 in]
            n20 = case shown="真" w22 {
              tunnel: w24 -> [_ w25]
              frame False {
              }
              frame True {
                n21 = local write "从板信息电压温度通道配置"(w25) -> ()
              }
            }
          }
        }
      }
      event "均衡参数设置": Value Change {
        n22 = event-data() -> ("NewVal"=w26:bool)  [unwired: 1 in, 5 out]
        n23 = case shown="真" w26 {
          frame False {
          }
          frame True {
            n24 = local read "均衡参数"() -> (w28:T1)
            n25 = call "均衡参数输入.vi"("均衡参数"=w28) -> ("均衡参数 2"=→"均衡参数":T1)
          }
        }
      }
      event "自动计算通道电压": Value Change {
        n26 = event-data() -> ("NewVal"=w29:bool)  [unwired: 1 in, 5 out]
        n27 = case shown="真" w29 {
          frame False {
          }
          frame True {
            n28 = local read "从板信息电压温度通道配置"() -> (w34:string[][])
            n29 = Index Array(array=w34, index (col)=1 ("禁用的索引 (列)")) -> (element=w40:string[])  [unwired: 1 in]
            n30 = Index Array(array=w40, index=0 ("索引")) -> (element=w38:string)
            n31 = Decimal String To Number(string=w38) -> (number=w37:i32)  [unwired: 2 in, 1 out]
            n32 = while {
              shift-right: [w48] -> _
              shift-left: w37 -> [w43]
              tunnel: [w46] -> w36 mode=indexing
              i -> [w55]
              stop <- w49 stop-if-true
              w45 = 12 ("y")
              n33 = local read "保险位置"() -> (w42:T6)
              n34 = Subtract(x=w43, y=w45) -> (x-y=w51:i32)
              n35 = Less?(x=w43, y=w45) -> (x < y?=w44:bool)
              n36 = Index Array(array=w42, index (row)=w55) -> (element=w54:T7[])  [unwired: 1 in]
              n37 = for {
                N: 12 -> [_]
                tunnel: w54 -> [w64] mode=indexing
                shift-right: [w65] -> w47
                shift-left: 0 -> [w62]
                n38 = Increment(x=w62) -> (x+1=w63:i32)
                n39 = Select(t=w63, s=w64, f=w62) -> (s? t:f=w65:i32)
              }
              n40 = Add(x=w51, y=w47) -> (x+y=w48:i32)
              n41 = case shown="真" w44 {
                tunnel: w47 -> [w58 w61]
                tunnel: [w57 w59] -> w46
                tunnel: w45 -> [w56 _]
                tunnel: w43 -> [_ w60]
                frame False {
                  n42 = Subtract(x=w56, y=w58) -> (x-y=w57:i32)
                }
                frame True {
                  n43 = Subtract(x=w60, y=w61) -> (x-y=w59:i32)
                }
              }
              n44 = Less Or Equal?(x=w48, y=0) -> (x <= y?=w49:bool)
            }
            n45 = Reshape Array(w36, 20 ("维数大小")) -> (w32:i32[])
            n46 = local write "5个通道电压个数(最小5个)"(w32) -> ()
            n47 = control-ref of="从板信息电压温度通道配置"() -> (w33:refnum<vi>)
            n48 = call "表格数据输入(数值)-8.6.vi"("行数"=u32 24, "列数"=u32 1, "数值数组"=w32, "表格引用"=w33) -> ()  [unwired: 8 in]
          }
        }
      }
      event Value Change {
        n49 = event-data() -> ("NewVal"=w70:T6)  [unwired: 1 in, 5 out]
        n50 = call "保险位置计算器.vi"("保险位置"=w70) -> ("输出数组"=w72:i32[])
        n51 = for {
          N: 20 -> [_]
          tunnel: w72 -> [w74] mode=indexing
          tunnel: [w73] -> w68 mode=indexing
          n52 = Number To Decimal String(number=w74) -> (decimal integer string=w73:string)  [unwired: 1 in]
        }
        n53 = control-ref of="从板信息电压温度通道配置"() -> (w69:refnum<vi>)
        n54 = call "表格数据输入-8.6.vi"("行数"=u32 2, "列数"=u32 1, "字符串数组"=w68, "表格引用"=w69) -> ()  [unwired: 8 in]
      }
      event "5个通道电压个数(最小5个)": Value Change {
        n55 = event-data() -> ()  [unwired: 1 in, 6 out]
        n56 = local read "5个通道电压个数(最小5个)"() -> (w75:u8[])
        n57 = for {
          N: 5 -> [_]
          tunnel: w75 -> [w82] mode=indexing
          tunnel: [w81] -> w78 mode=indexing
          n58 = Number To Decimal String(number=w82) -> (decimal integer string=w81:string)  [unwired: 1 in]
        }
        n59 = control-ref of="从板信息电压温度通道配置"() -> (w79:refnum<vi>)
        n60 = call "表格数据输入-8.6.vi"("行数"=u32 22, "列数"=u32 1, "字符串数组"=w78, "表格引用"=w79) -> ()  [unwired: 8 in]
      }
      event "电压个数": Value Change {
        n61 = event-data() -> ()  [unwired: 1 in, 6 out]
        n62 = local read "电压个数"() -> (w83:dbl)
        n63 = for {
          N: 1 -> [_]
          tunnel: w83 -> [w90]
          tunnel: [w89] -> w86 mode=indexing
          n64 = Number To Decimal String(number=w90) -> (decimal integer string=w89:string)  [unwired: 1 in]
        }
        n65 = control-ref of="从板信息电压温度通道配置"() -> (w87:refnum<vi>)
        n66 = call "表格数据输入-8.6.vi"("行数"=u32 0, "列数"=u32 1, "字符串数组"=w86, "表格引用"=w87) -> ()  [unwired: 8 in]
      }
      event "温度个数": Value Change {
        n67 = event-data() -> ()  [unwired: 1 in, 6 out]
        n68 = local read "温度个数"() -> (w91:dbl)
        n69 = for {
          N: 1 -> [_]
          tunnel: w91 -> [w98]
          tunnel: [w97] -> w94 mode=indexing
          n70 = Number To Decimal String(number=w98) -> (decimal integer string=w97:string)  [unwired: 1 in]
        }
        n71 = control-ref of="从板信息电压温度通道配置"() -> (w95:refnum<vi>)
        n72 = call "表格数据输入-8.6.vi"("行数"=u32 1, "列数"=u32 1, "字符串数组"=w94, "表格引用"=w95) -> ()  [unwired: 8 in]
      }
      event "通道电压清零": Value Change {
        n73 = event-data() -> ("NewVal"=w99:bool)  [unwired: 1 in, 5 out]
        n74 = case shown="真" w99 {
          frame False {
          }
          frame True {
            n75 = Reshape Array(u8[] [0, 0, 0, 0, 0, 0, 0, 0, 0, 0, 0, 0, 0, 0, 0, 0, 0, 0, 0, 0] ("20个通道电压个数"), 20 ("维数大小")) -> (w100:u8[])
            n76 = local write "5个通道电压个数(最小5个)"(w100) -> ()
            n77 = control-ref of="从板信息电压温度通道配置"() -> (w103:refnum<vi>)
            n78 = call "表格数据输入(数值)-8.6.vi"("行数"=u32 24, "列数"=u32 1, "数值数组"=w100, "表格引用"=w103) -> ()  [unwired: 8 in]
          }
        }
      }
      event "保险位置清零": Value Change {
        n79 = event-data() -> ("NewVal"=w106:bool)  [unwired: 1 in, 5 out]
        n80 = case shown="真" w106 {
          frame False {
          }
          frame True {
            n81 = local write "保险位置"(bool[][] [] ("保险位置")) -> ()
            n82 = control-ref of="从板信息电压温度通道配置"() -> (w110:refnum<vi>)
            n83 = call "表格数据输入-8.6.vi"("行数"=u32 2, "列数"=u32 1, "字符串数组"=string[] ["0", "0", "0", "0", "0", "0", "0", "0", "0", "0", "0", "0", "0", "0", "0", "0", "0", "0", "0", "0"], "表格引用"=w110) -> ()  [unwired: 8 in]
          }
        }
      }
      event Value Change {
        n84 = event-data() -> ("NewVal"=w112:T5)  [unwired: 1 in, 5 out]
        n85 = case shown="真" w112 {
          frame False {
          }
          frame True {
            n86 = local read "从板信息电压温度通道配置"() -> (w135:string[][])
            n87 = local read "一级故障 2"() -> (w132:dbl[][])
            n88 = local read "均衡参数"() -> (w114:T1)
            n89 = local read "加热控制参数 2"() -> (w134:T3)
            n90 = Transpose 2D Array(2D array=w132) -> (transposed array=w119:dbl[][])
            n91 = Cluster To Array(cluster=w114) -> (array=w113:sgl[])
            n92 = Array Subset(array=w135, index (row)=0 ("索引"), index (col)=0 ("索引"), length (col)=2 ("索引")) -> (w130:string[][])  [unwired: 1 in]
            n93 = for {
              tunnel: w119 -> [w154] mode=indexing
              shift-right: [w153] -> w128
              shift-left: string[] [] -> [w151]
              n94 = for {
                N: 7 -> [_]
                tunnel: w154 -> [w157] mode=indexing
                tunnel: [w155] -> w152 mode=indexing
                n95 = Format Into String(format string="%#f" ("格式字符串"), w157) -> (resulting string=w155:string)  [unwired: 2 in, 1 out]
              }
              n96 = Insert Into Array(array=w151, new element=w152) -> (w153:string[])  [unwired: 1 in]
            }
            n97 = Cluster To Array(cluster=w134) -> (array=w133:dbl[])
            n98 = for {
              tunnel: w113 -> [w141] mode=indexing
              tunnel: [w139] -> _ mode=indexing
              n99 = Format Into String(format string="%#f" ("格式字符串"), w141) -> (resulting string=w139:string)  [unwired: 2 in, 1 out]
            }
            n100 = Index Array(array=w130, index (col) #2=1 ("索引 (列)")) -> (element #2=w116:string[])  [unwired: 3 in, 1 out]
            n101 = for {
              tunnel: w133 -> [w160] mode=indexing
              tunnel: [w158] -> w129 mode=indexing
              n102 = Format Into String(format string="%#f" ("格式字符串"), w160) -> (resulting string=w158:string)  [unwired: 2 in, 1 out]
            }
            n103 = local read "从板板号"() -> (w123:dbl)
            n104 = Array Subset(array=w116, length=27 ("长度")) -> (w117:string[])  [unwired: 1 in]
            n105 = Number To Decimal String(number=w123) -> (decimal integer string=w121:string)  [unwired: 1 in]
            n106 = Insert Into Array(array=w117, new element #1=w129, new element #2=w128) -> (w127:string[])  [unwired: 1 in]
            n107 = Decrement(x=w123) -> (x-1=w118:dbl)
            n108 = local read "输出数组"() -> (w125:string[][])
            n109 = Insert Into Array(array=w127, index=0 ("索引"), new element=w121) -> (w124:string[])
            n110 = Replace Array Subset(array=w125, new element=w124, index (col)=w118) -> (w122:string[][])  [unwired: 1 in]
            n111 = stacked-sequence {
              tunnel: w122 -> [w142]
              tunnel: w121 -> [w147]
              frame #0 {
                n112 = control-ref of="结果"() -> (w149:refnum<vi>)
                n113 = Concatenate Strings("从板", w147, "保存成功") -> (w145:string)
                n114 = local write "输出数组"(w142) -> ()
                n115 = Build Array(w145) -> (w143:string[])
                n116 = call "表格编辑.vi"("新元素/子数组"=w143, "活动单元格:单元格背景色"=u32 6618880, "MCListbox引用句柄"=w149) -> ()  [unwired: 9 in]
              }
            }
          }
        }
      }
      event "全部记录": Value Change {
        n117 = event-data() -> ("NewVal"=w161:bool)  [unwired: 1 in, 5 out]
        n118 = case shown="真" w161 {
          frame False {
          }
          frame True {
            n119 = local read "从板个数"() -> (w165:dbl)
            n120 = for {
              N: w165 -> [_]
              tunnel: [w173] -> w164 mode=indexing
              i -> [w174]
              n121 = local read "从板信息电压温度通道配置"() -> (w189:string[][])
              n122 = local read "一级故障 2"() -> (w186:dbl[][])
              n123 = local read "加热控制参数 2"() -> (w188:T3)
              n124 = local read "均衡参数"() -> (w169:T1)
              n125 = Transpose 2D Array(2D array=w186) -> (transposed array=w177:dbl[][])
              n126 = Array Subset(array=w189, index (row)=0 ("索引"), index (col)=0 ("索引"), length (col)=2 ("索引")) -> (w184:string[][])  [unwired: 1 in]
              n127 = for {
                tunnel: w177 -> [w207] mode=indexing
                shift-right: [w206] -> w181
                shift-left: string[] [] -> [w204]
                n128 = for {
                  N: 7 -> [_]
                  tunnel: w207 -> [w210] mode=indexing
                  tunnel: [w208] -> w205 mode=indexing
                  n129 = Format Into String(format string="%#f" ("格式字符串"), w210) -> (resulting string=w208:string)  [unwired: 2 in, 1 out]
                }
                n130 = Insert Into Array(array=w204, new element=w205) -> (w206:string[])  [unwired: 1 in]
              }
              n131 = Cluster To Array(cluster=w169) -> (array=w168:sgl[])
              n132 = Cluster To Array(cluster=w188) -> (array=w187:dbl[])
              n133 = Index Array(array=w184, index (col) #1=0 ("禁用的索引 (列)"), index (col) #2=1 ("索引 (列)")) -> (element #2=w171:string[])  [unwired: 2 in, 1 out]
              n134 = for {
                tunnel: w187 -> [w213] mode=indexing
                tunnel: [w211] -> w182 mode=indexing
                n135 = Format Into String(format string="%#f" ("格式字符串"), w213) -> (resulting string=w211:string)  [unwired: 2 in, 1 out]
              }
              n136 = for {
                tunnel: w168 -> [w195] mode=indexing
                tunnel: [w193] -> w167 mode=indexing
                n137 = Format Into String(format string="%#f" ("格式字符串"), w195) -> (resulting string=w193:string)  [unwired: 2 in, 1 out]
              }
              n138 = Array Subset(array=w171, length=44 ("长度")) -> (w172:string[])  [unwired: 1 in]
              n139 = Increment(x=w174) -> (x+1=w176:i32)
              n140 = Number To Decimal String(number=w176) -> (decimal integer string=w179:string)  [unwired: 1 in]
              n141 = stacked-sequence {
                tunnel: w179 -> [w200]
                frame #0 {
                  n142 = control-ref of="结果"() -> (w202:refnum<vi>)
                  n143 = Concatenate Strings("从板", w200, "记录完成") -> (w198:string)
                  n144 = Build Array(w198) -> (w196:string[])
                  n145 = call "表格编辑.vi"("新元素/子数组"=w196, "活动单元格:单元格背景色"=u32 6618880, "MCListbox引用句柄"=w202) -> ()  [unwired: 9 in]
                }
              }
              n146 = Insert Into Array(array=w172, new element #1=w182, new element #2=w181, new element #3=w167) -> (w180:string[])  [unwired: 1 in]
              n147 = Insert Into Array(array=w180, index=0 ("索引"), new element=w179) -> (w173:string[])
            }
            n148 = local write "从板表头"(string[] ["从板板号", "电压个数", "电压起始值", "温度个数", "温度起始值", "第一个保险通道", "第一个保险位置", "第二个保险通道", "第二个保险位置", "第三个保险通道", "第三个保险位置", "第四个保险通道", "第四个保险位置", "第五个保险通道", "第五个保险位置", "第六个保险通道", "第六个保险位置", "第七个保险通道", "第七个保险位置", "第八个保险通道", "第八个保险位置", "第九个保险通道", "第九个保险位置", "第十个保险通道", "第十个保险位置", "第1通道电压个数", "第2通道电压个数", "第3通道电压个数", "第4通道电压个数", "第5通道电压个数", "第6通道电压个数", "第7通道电压个数", "第8通道电压个数", "第9通道电压个数", "第10通道电压个数", "第11通道电压个数", "第12通道电压个数", "第13通道电压个数", "第14通道电压个数", "第15通道电压个数", "第16通道电压个数", "第17通道电压个数", "第18通道电压个数", "第19通道电压个数", "第20通道电压个数", "风机开启温度", "风机关闭温度", "加热开启温度", "加热关闭温度", "风机开启温差", "风机关闭温差", "加热关闭温差", "电压过高一级", "电压过低一级", "温度过高一级", "温度过低一级", "电压不均衡一级", "温度不均衡一级", "SOC过低一级", "电压过高二级", "电压过低二级", "温度过高二级", "温度过低二级", "电压不均衡二级", "温度不均衡二级", "SOC过低二级", "电压过高三级", "电压过低三级", "温度过高三级", "温度过低三级", "电压不均衡三级", "温度不均衡三级", "SOC过低三级", "均衡计算-电压高阀值1级", "均衡计算-电压高阀值2级", "均衡计算-电压低阀值1级", "均衡计算-电压低阀值2级", "均衡计算-最低电压阀值", "均衡停止-最低电压阀值", "均衡计算-电压极差阀值", "充电结束电压(90%)", "充电结束电压(91%)", "充电结束电压(92%)", "充电结束电压(93%)", "充电结束电压(94%)", "充电结束电压(95%)", "充电结束电压(96%)", "充电结束电压(97%)", "充电结束电压(98%)", "充电结束电压(99%)", "充电结束电压(100%)"] ("从板表头")) -> ()
            n149 = property on="查看" class="Bool (严格)"("Visible"=TRUE ("可见")) -> ()  [unwired: 2 in, 2 out]
            n150 = Transpose 2D Array(2D array=w164) -> (transposed array=w163:string[][])
            n151 = local write "输出数组"(w163) -> ()
          }
        }
      }
      event "主从板": Value Change {
        n152 = event-data() -> ()  [unwired: 1 in, 6 out]
        n153 = control-ref of="单选选项2"() -> (w219:refnum<vi>)
        n154 = control-ref of="单选选项1"() -> (w218:refnum<vi>)
        n155 = local read "主从板"() -> (w214:enum32{"单选选项2", "单选选项1"})
        n156 = case shown="\"单选选项2\"" w214 {
          frame "单选选项2" {
            n157 = case shown="假" TRUE {
              frame False {
                n158 = stacked-sequence {
                  seq-local: [w227 _] -> [_ w295]
                  seq-local: [w226 _] -> [_ w293]
                  frame #0 {
                    n159 = local read "主板信息"() -> (w233:string[][])
                    n160 = local read "从板个数"() -> (w228:dbl)
                    n161 = Index Array(array=w233, index (col) #1=0 ("禁用的索引 (列)"), index (col) #2=1 ("索引 (列)")) -> (element #1=w230:string[], element #2=w229:string[])  [unwired: 2 in]
                    n162 = for {
                      N: w228 -> [_]
                      tunnel: w230 -> [w268]
                      tunnel: w229 -> [w260]
                      tunnel: [w245] -> w225
                      tunnel: [w252] -> w224
                      i -> [w245]
                      n163 = Cluster To Array(cluster=T8 {"风机开启温度(℃)"=35.0, "风机关闭温度(℃)"=30.0, "加热开启温度(℃)"=0.0, "加热关闭温度(℃)"=5.0, "风机开启温差(℃)"=5.0, "风机开启温度(℃)"=3.0, "加热关闭温差(℃)"=10.0} ("加热控制参数")) -> (array=w247:dbl[])
                      n164 = local read "输出数组"() -> (w246:string[][])
                      n165 = Transpose 2D Array(2D array=dbl[][] [[4.23, 4.25, 4.3], [3.0, 2.75, 2.5], [50.0, 55.0, 60.0], [-20.0, -30.0, -40.0], [0.5, 1.0, 1.5], [25.0, 30.0, 35.0], [30.0, 20.0, 10.0]] ("一级故障 2")) -> (transposed array=w248:dbl[][])
                      n166 = Search 1D Array(1D array=w268, element="从板1电池节数" ("元素")) -> (index of element=w265:i32)  [unwired: 1 in]
                      n167 = Search 1D Array(1D array=w268, element="从板1电压起始值" ("元素")) -> (index of element=w263:i32)  [unwired: 1 in]
                      n168 = Search 1D Array(1D array=w268, element="从板1温度个数" ("元素")) -> (index of element=w259:i32)  [unwired: 1 in]
                      n169 = Search 1D Array(1D array=w268, element="从板1温度起始值" ("元素")) -> (index of element=w258:i32)  [unwired: 1 in]
                      n170 = for {
                        tunnel: w247 -> [w285] mode=indexing
                        tunnel: [w283] -> w240 mode=indexing
                        n171 = Format Into String(format string="%#f" ("格式字符串"), w285) -> (resulting string=w283:string)  [unwired: 2 in, 1 out]
                      }
                      n172 = for {
                        tunnel: w248 -> [w279] mode=indexing
                        shift-right: [w278] -> w236
                        shift-left: _ -> [w276]
                        n173 = for {
                          N: 7 -> [_]
                          tunnel: w279 -> [w282] mode=indexing
                          tunnel: [w280] -> w277 mode=indexing
                          n174 = Format Into String(format string="%#f" ("格式字符串"), w282) -> (resulting string=w280:string)  [unwired: 2 in, 1 out]
                        }
                        n175 = Insert Into Array(array=w276, new element=w277) -> (w278:string[])  [unwired: 1 in]
                      }
                      n176 = Add(x=w265, y=w245) -> (x+y=w266:i32)
                      n177 = Add(x=w263, y=w245) -> (x+y=w264:i32)
                      n178 = Add(x=w258, y=w245) -> (x+y=w261:i32)
                      n179 = Add(x=w259, y=w245) -> (x+y=w262:i32)
                      n180 = Index Array(array=w246, index (col)=w245) -> (element=w244:string[])  [unwired: 1 in]
                      n181 = Index Array(array=w260, index=w266) -> (element=w257:string)
                      n182 = Index Array(array=w260, index=w264) -> ()  [unwired: 1 out]
                      n183 = Index Array(array=w260, index=w261) -> ()  [unwired: 1 out]
                      n184 = Index Array(array=w260, index=w262) -> (element=w256:string)
                      n185 = local read "均衡参数"() -> (w239:T1)
                      n186 = Array Subset(array=w244, index=3 ("索引"), length=27 ("长度")) -> (w241:string[])
                      n187 = Increment(x=w245) -> (x+1=w251:i32)
                      n188 = Number To Decimal String(number=w251) -> (decimal integer string=w255:string)  [unwired: 1 in]
                      n189 = Cluster To Array(cluster=w239) -> (array=w238:sgl[])
                      n190 = local read "输出数组"() -> (w254:string[][])
                      n191 = for {
                        tunnel: w238 -> [w274] mode=indexing
                        tunnel: [w272] -> w237 mode=indexing
                        n192 = Format Into String(format string="%#f" ("格式字符串"), w274) -> (resulting string=w272:string)  [unwired: 2 in, 1 out]
                      }
                      n193 = Build Array (concatenate)(w255, w257, w256, w241, w240, w236, w237) -> (w253:string[])
                      n194 = Replace Array Subset(array=w254, new element=w253, index (col)=w245) -> (w252:string[][])  [unwired: 1 in]
                      n195 = local write "输出数组"(w252) -> ()
                    }
                    n196 = stacked-sequence {
                      tunnel: [w234] -> w227
                      tunnel: [w235] -> w226
                      tunnel: w225 -> [_]
                      tunnel: w224 -> [w235]
                      frame #0 {
                        w234 = string[] ["从板板号", "电压个数", "温度个数", "第一个保险通道", "第一个保险位置", "第二个保险通道", "第二个保险位置", "第三个保险通道", "第三个保险位置", "第四个保险通道", "第四个保险位置", "第五个保险通道", "第五个保险位置", "第六个保险通道", "第六个保险位置", "第七个保险通道", "第七个保险位置", "第八个保险通道", "第八个保险位置", "第九个保险通道", "第九个保险位置", "第十个保险通道", "第十个保险位置", "第1通道电压个数", "第2通道电压个数", "第3通道电压个数", "第4通道电压个数", "第5通道电压个数", "风机开启温度", "风机关闭温度", "加热开启温度", "加热关闭温度", "风机开启温差", "风机关闭温差", "加热关闭温差", "电压过高一级", "电压过低一级", "温度过高一级", "温度过低一级", "电压不均衡一级", "温度不均衡一级", "SOC过低一级", "电压过高二级", "电压过低二级", "温度过高二级", "温度过低二级", "电压不均衡二级", "温度不均衡二级", "SOC过低二级", "电压过高三级", "电压过低三级", "温度过高三级", "温度过低三级", "电压不均衡三级", "温度不均衡三级", "SOC过低三级", "均衡计算-电压高阀值1级", "均衡计算-电压高阀值2级", "均衡计算-电压低阀值1级", "均衡计算-电压低阀值2级", "均衡计算-最低电压阀值", "均衡停止-最低电压阀值", "均衡计算-电压极差阀值", "充电结束电压(90%)", "充电结束电压(91%)", "充电结束电压(92%)", "充电结束电压(93%)", "充电结束电压(94%)", "充电结束电压(95%)", "充电结束电压(96%)", "充电结束电压(97%)", "充电结束电压(98%)", "充电结束电压(99%)", "充电结束电压(100%)"] ("从板表头")
                        n197 = local write "从板表头"(w234) -> ()
                      }
                    }
                  }
                  frame #1 {
                    (unwired) string[] ["从板板号", "电压个数", "电压起始值", "温度个数", "温度起始值", "第一个保险通道", "第一个保险位置", "第二个保险通道", "第二个保险位置", "第三个保险通道", "第三个保险位置", "第四个保险通道", "第四个保险位置", "第五个保险通道", "第五个保险位置", "第六个保险通道", "第六个保险位置", "第七个保险通道", "第七个保险位置", "第八个保险通道", "第八个保险位置", "第九个保险通道", "第九个保险位置", "第十个保险通道", "第十个保险位置", "第1通道电压个数", "第2通道电压个数", "第3通道电压个数", "第4通道电压个数", "第5通道电压个数", "第6通道电压个数", "第7通道电压个数", "第8通道电压个数", "第9通道电压个数", "第10通道电压个数", "第11通道电压个数", "第12通道电压个数", "第13通道电压个数", "第14通道电压个数", "第15通道电压个数", "第16通道电压个数", "第17通道电压个数", "第18通道电压个数", "第19通道电压个数", "第20通道电压个数", "风机开启温度", "风机关闭温度", "加热开启温度", "加热关闭温度", "风机开启温差", "风机关闭温差", "加热关闭温差", "电压过高一级", "电压过低一级", "温度过高一级", "温度过低一级", "电压不均衡一级", "温度不均衡一级", "SOC过低一级", "电压过高二级", "电压过低二级", "温度过高二级", "温度过低二级", "电压不均衡二级", "温度不均衡二级", "SOC过低二级", "电压过高三级", "电压过低三级", "温度过高三级", "温度过低三级", "电压不均衡三级", "温度不均衡三级", "SOC过低三级", "均衡计算-电压高阀值1级", "均衡计算-电压高阀值2级", "均衡计算-电压低阀值1级", "均衡计算-电压低阀值2级", "均衡计算-最低电压阀值", "均衡停止-最低电压阀值", "均衡计算-电压极差阀值", "充电结束电压(90%)", "充电结束电压(91%)", "充电结束电压(92%)", "充电结束电压(93%)", "充电结束电压(94%)", "充电结束电压(95%)", "充电结束电压(96%)", "充电结束电压(97%)", "充电结束电压(98%)", "充电结束电压(99%)", "充电结束电压(100%)"] ("从板表头")
                    n198 = local read "从板板号"() -> (w292:dbl)
                    n199 = Search 1D Array(1D array=w295, element="风机开启温度" ("元素")) -> (index of element=w314:i32)  [unwired: 1 in]
                    n200 = Search 1D Array(1D array=w295, element="电压过高一级" ("元素"), start index (0)=w314) -> (index of element=w312:i32)
                    n201 = Decrement(x=w292) -> (x-1=w291:dbl)
                    n202 = Index Array(array=w293, index (col)=w291) -> (element=w290:string[])  [unwired: 1 in]
                    n203 = Decrement(x=w314) -> (x-1=w316:i32)
                    n204 = Array Subset(array=w290, index=1 ("索引"), length=w316) -> (w318:string[])
                    n205 = Array Subset(array=w290, index=w312, length=21 ("长度")) -> (w298:string[])
                    n206 = Array Subset(array=w290, index=w314, length=7 ("长度")) -> (w310:string[])
                    n207 = for {
                      tunnel: w298 -> [w322] mode=indexing
                      tunnel: [w321] -> w297 mode=indexing
                      n208 = Fract/Exp String To Number(string=w322) -> (number=w321:dbl)  [unwired: 3 in, 1 out]
                    }
                    n209 = for {
                      tunnel: w310 -> [w324] mode=indexing
                      tunnel: [w323] -> w294 mode=indexing
                      n210 = Fract/Exp String To Number(string=w324) -> (number=w323:dbl)  [unwired: 3 in, 1 out]
                    }
                    n211 = Array Subset(array=string[] ["从板板号", "电压个数", "温度个数", "第一个保险通道", "第一个保险位置", "第二个保险通道", "第二个保险位置", "第三个保险通道", "第三个保险位置", "第四个保险通道", "第四个保险位置", "第五个保险通道", "第五个保险位置", "第六个保险通道", "第六个保险位置", "第七个保险通道", "第七个保险位置", "第八个保险通道", "第八个保险位置", "第九个保险通道", "第九个保险位置", "第十个保险通道", "第十个保险位置", "第1通道电压个数", "第2通道电压个数", "第3通道电压个数", "第4通道电压个数", "第5通道电压个数", "第6通道电压个数", "第7通道电压个数", "第8通道电压个数", "第9通道电压个数", "第10通道电压个数", "第11通道电压个数", "第12通道电压个数", "第13通道电压个数", "第14通道电压个数", "第15通道电压个数", "第16通道电压个数", "第17通道电压个数", "第18通道电压个数", "第19通道电压个数", "第20通道电压个数", "风机开启温度", "风机关闭温度", "加热开启温度", "加热关闭温度", "风机开启温差", "风机关闭温差", "加热关闭温差", "电压过高一级", "电压过低一级", "温度过高一级", "温度过低一级", "电压不均衡一级", "温度不均衡一级", "SOC过低一级", "电压过高二级", "电压过低二级", "温度过高二级", "温度过低二级", "电压不均衡二级", "温度不均衡二级", "SOC过低二级", "电压过高三级", "电压过低三级", "温度过高三级", "温度过低三级", "电压不均衡三级", "温度不均衡三级", "SOC过低三级", "均衡计算-电压高阀值1级", "均衡计算-电压高阀值2级", "均衡计算-电压低阀值1级", "均衡计算-电压低阀值2级", "均衡计算-最低电压阀值", "均衡停止-最低电压阀值", "均衡计算-电压极差阀值", "充电结束电压(90%)", "充电结束电压(91%)", "充电结束电压(92%)", "充电结束电压(93%)", "充电结束电压(94%)", "充电结束电压(95%)", "充电结束电压(96%)", "充电结束电压(97%)", "充电结束电压(98%)", "充电结束电压(99%)", "充电结束电压(100%)"] ("从板表头"), index=1 ("长度"), length=27 ("长度")) -> (w286:string[])
                    n212 = Delete From Array(array=w297, length=7 ("长度"), index=0 ("索引")) -> (deleted portion=w306:dbl[], array with subset deleted=w305:dbl[])
                    n213 = Build Array(w286, w318) -> (w317:string[][])
                    n214 = Array To Cluster(array=w294) -> (cluster=w309:T10)
                    n215 = Delete From Array(array=w305, length=7 ("长度"), index=0 ("索引")) -> (deleted portion=w302:dbl[], array with subset deleted=w301:dbl[])
                    n216 = Transpose 2D Array(2D array=w317) -> (transposed array=w296:string[][])
                    n217 = local write "加热控制参数 2"(w309) -> ()
                    n218 = Build Array(w306, w302, w301) -> (w300:dbl[][])
                    n219 = local write "从板信息电压温度通道配置"(w296) -> ()
                    n220 = Transpose 2D Array(2D array=w300) -> (transposed array=w299:dbl[][])
                    n221 = local write "一级故障 2"(w299) -> ()
                  }
                }
              }
              frame True {
              }
            }
          }
          frame "单选选项1", Default {
          }
        }
        n222 = Build Array(w218, w219) -> (w220:refnum<vi>[])
        n223 = case shown="\"单选选项2\", 默认" w214 {
          selector: w214 -> [w329 w334]
          tunnel: [enum32{"主板", "从板", "预览"}."从板" ("选项卡控件") enum32{"主板", "从板", "预览"}."主板" ("选项卡控件")] -> w217
          tunnel: w220 -> [w330 w335]
          tunnel: [w328 w333] -> w221
          tunnel: [w327 w332] -> w222
          frame "单选选项2", Default {
            n224 = Delete From Array(array=w330, index=w329) -> (deleted portion=w327:refnum<vi>, array with subset deleted=w328:refnum<vi>[])  [unwired: 1 in]
          }
          frame "单选选项1" {
            n225 = Delete From Array(array=w335, index=w334) -> (deleted portion=w332:refnum<vi>, array with subset deleted=w333:refnum<vi>[])  [unwired: 1 in]
          }
        }
        n226 = for {
          tunnel: u32 65511 -> [w326]
          tunnel: w221 -> [w325] mode=indexing
          n227 = property class="Bool (严格)"(reference=w325, "BoolText.TextColor"=w326) -> ()  [unwired: 1 in, 2 out]
        }
        n228 = local write "选项卡控件"(w217) -> ()
        n229 = property class="Bool (严格)"(reference=w222, "BoolText.TextColor"=u32 16119285) -> ()  [unwired: 1 in, 2 out]
      }
      event "默认值 2": Value Change {
        n230 = event-data() -> ("NewVal"=w337:bool)  [unwired: 1 in, 5 out]
        n231 = case shown="真" w337 {
          frame False {
          }
          frame True {
            n232 = local write "保险位置"(bool[][] [] ("保险位置")) -> ()
            n233 = local write "一级故障 2"(dbl[][] [[4.23, 4.25, 4.3], [3.0, 2.75, 2.5], [50.0, 55.0, 60.0], [-20.0, -30.0, -40.0], [0.5, 1.0, 1.5], [25.0, 30.0, 35.0], [30.0, 20.0, 10.0]] ("一级故障 2")) -> ()
            n234 = local write "加热控制参数 2"(T8 {"风机开启温度(℃)"=35.0, "风机关闭温度(℃)"=30.0, "加热开启温度(℃)"=0.0, "加热关闭温度(℃)"=5.0, "风机开启温差(℃)"=5.0, "风机开启温度(℃)"=3.0, "加热关闭温差(℃)"=10.0} ("加热控制参数")) -> ()
            n235 = Reshape Array(u8[] [0, 0, 0, 0, 0, 0, 0, 0, 0, 0, 0, 0, 0, 0, 0, 0, 0, 0, 0, 0] ("20个通道电压个数"), 5 ("维数大小")) -> (w342:u8[])
            n236 = control-ref of="从板信息电压温度通道配置"() -> (w338:refnum<vi>)
            n237 = local write "5个通道电压个数(最小5个)"(w342) -> ()
            n238 = call "表格数据输入-8.6.vi"("行数"=u32 4, "列数"=u32 1, "字符串数组"=string[] ["", "", "", "", "", "", "", "", "", "", "", "", "", "", "", "", "", ""], "表格引用"=w338) -> ()  [unwired: 8 in]
            n239 = call "表格数据输入(数值)-8.6.vi"("行数"=u32 22, "列数"=u32 1, "数值数组"=w342, "表格引用"=w338) -> ()  [unwired: 8 in]
          }
        }
      }
      event "全部清零(从板)": Value Change {
        n240 = event-data() -> ("NewVal"=w350:bool)  [unwired: 1 in, 5 out]
        n241 = case shown="真" w350 {
          frame False {
          }
          frame True {
            n242 = control-ref of="从板信息电压温度通道配置"() -> (w356:refnum<vi>)
            n243 = local write "一级故障 2"(dbl[][] [[0.0, 0.0, 0.0], [0.0, 0.0, 0.0], [0.0, 0.0, 0.0], [0.0, 0.0, 0.0], [0.0, 0.0, 0.0], [0.0, 0.0, 0.0], [0.0, 0.0, 0.0]] ("一级故障 2")) -> ()
            n244 = call "表格数据输入-8.6.vi"("行数"=u32 0, "列数"=u32 1, "字符串数组"=string[] ["", "", "", "", "", "", "", "", "", "", "", "", "", "", "", "", "", "", "", "", "", "", "", "", "", "", "", " "], "表格引用"=w356) -> ()  [unwired: 8 in]
            n245 = local write "加热控制参数 2"(T8 {"风机开启温度(℃)"=0.0, "风机关闭温度(℃)"=0.0, "加热开启温度(℃)"=0.0, "加热关闭温度(℃)"=0.0, "风机开启温差(℃)"=0.0, "风机开启温度(℃)"=0.0, "加热关闭温差(℃)"=0.0} ("加热控制参数")) -> ()
            n246 = Reshape Array(u8[] [0, 0, 0, 0, 0, 0, 0, 0, 0, 0, 0, 0, 0, 0, 0, 0, 0, 0, 0, 0] ("20个通道电压个数"), 20 ("维数大小")) -> (w352:u8[])
            n247 = local write "5个通道电压个数(最小5个)"(w352) -> ()
            n248 = local write "保险位置"(bool[][] [] ("保险位置")) -> ()
          }
        }
      }
      event "设电池信息主板": Value Change {
        n249 = event-data() -> ("NewVal"=w361:bool)  [unwired: 1 in, 5 out]
        n250 = case shown="真" w361 {
          frame False {
          }
          frame True {
            n251 = local read "电池信息"() -> (w363:string[][])
            n252 = call "主板电池信息配置.vi"("电池信息查看"=w363) -> ("输出数组"=w364:string[][], "布尔"=w362:bool)  [unwired: 1 in]
            n253 = case shown="真" w362 {
              tunnel: w364 -> [_ w365]
              frame False {
              }
              frame True {
                n254 = local write "电池信息"(w365) -> ()
              }
            }
          }
        }
      }
      event "写配置文件": Value Change {
        n255 = event-data() -> ("NewVal"=w366:bool)  [unwired: 1 in, 5 out]
        n256 = case shown="真" w366 {
          frame False {
          }
          frame True {
            n257 = for {
              N: 2 -> [_]
              i -> [w369]
              n258 = stacked-sequence {
                seq-local: [w397 _ _] -> [_ w453 _]
                seq-local: [w395 _ _] -> [_ w447 _]
                seq-local: [w393 _ _] -> [_ w449 _]
                seq-local: [_ w448 _] -> [_ _ w496]
                seq-local: [w392 _ _] -> [_ _ w495]
                seq-local: [_ w443 _] -> [_ _ w494]
                seq-local: [_ w442 _] -> [_ _ w493]
                tunnel: w369 -> [_ w441 _]
                tunnel: w369 -> [_ w440 w492]
                frame #0 {
                  n259 = local read "一级故障"() -> (w409:dbl[][])
                  n260 = local read "充电控制参数"() -> (w381:T4)
                  n261 = local read "主板信息"() -> (w410:string[][])
                  n262 = local read "电池信息"() -> (w400:string[][])
                  n263 = local read "加热控制参数"() -> (w406:T3)
                  n264 = Array Subset(array=w410, index (row)=0 ("索引"), index (col)=0 ("索引"), length (col)=2 ("索引")) -> (w412:string[][])  [unwired: 1 in]
                  n265 = Transpose 2D Array(2D array=w409) -> (transposed array=w391:dbl[][])
                  n266 = for {
                    tunnel: w391 -> [w426] mode=indexing
                    shift-right: [w425] -> w385
                    shift-left: string[] [] -> [w423]
                    n267 = for {
                      N: 17 -> [_]
                      tunnel: w426 -> [w429] mode=indexing
                      tunnel: [w427] -> w424 mode=indexing
                      n268 = Format Into String(format string="%#f" ("格式字符串"), w429) -> (resulting string=w427:string)  [unwired: 2 in, 1 out]
                    }
                    n269 = Insert Into Array(array=w423, new element=w424) -> (w425:string[])  [unwired: 1 in]
                  }
                  n270 = Unbundle(w381) -> ("最大允许单体电压(V)"=w380:dbl, "最大允许总电压(V)"=w376:dbl, "最小允许单体电压(V)"=w379:dbl, "最大允许充电电流(A)"=w378:dbl, "最小允许充电电流(A)"=w377:dbl, "最大允许充电温度(℃)"=w375:dbl, "最小允许充电温度(℃)"=w374:dbl, "电流步长"=w373:dbl)
                  n271 = Index Array(array=w412, index (col) #1=1 ("禁用的索引 (列)"), index (col) #2=0 ("索引 (列)")) -> (element #1=w390:string[], element #2=w395:string[])  [unwired: 2 in]
                  n272 = local read "从板个数"() -> (w392:dbl)
                  n273 = Array Subset(array=w400, index (row)=0 ("索引"), index (col)=0 ("索引"), length (col)=2 ("索引")) -> (w404:string[][])  [unwired: 1 in]
                  n274 = Cluster To Array(cluster=w406) -> (array=w407:dbl[])
                  n275 = local read "分流器型号"() -> (w371:T2)
                  n276 = for {
                    tunnel: w407 -> [w421] mode=indexing
                    tunnel: [w419] -> w389 mode=indexing
                    n277 = Format Into String(format string="%#f" ("格式字符串"), w421) -> (resulting string=w419:string)  [unwired: 2 in, 1 out]
                  }
                  n278 = Build Array(w380, w379, w378, w377, w376, w375, w374, w373) -> (w372:dbl[])
                  n279 = Index Array(array=w404, index (col) #1=0 ("禁用的索引 (列)"), index (col) #2=1 ("禁用的索引 (列)")) -> (element #1=w393:string[], element #2=w387:string[])  [unwired: 2 in]
                  n280 = for {
                    tunnel: w372 -> [w418] mode=indexing
                    tunnel: [w416] -> w388 mode=indexing
                    n281 = Format Into String(format string="%#f" ("格式字符串"), w418) -> (resulting string=w416:string)  [unwired: 2 in, 1 out]
                  }
                  n282 = Number To Decimal String(number=w392) -> (decimal integer string=w399:string)  [unwired: 1 in]
                  n283 = Number To Decimal String(number=w371) -> (decimal integer string=w370:string)  [unwired: 1 in]
                  n284 = Array Subset(array=w385, index=0 ("索引"), length=51 ("长度")) -> (w382:string[])
                  n285 = Insert Into Array(array=w390, new element #1=w382, new element #2=w389, new element #3=w388, new element #4=w387, new element #5=w370) -> (w386:string[])  [unwired: 1 in]
                  n286 = Insert Into Array(array=w386, index=0 ("索引"), new element=w399) -> (w397:string[])
                }
                frame #1 {
                  w434 = ".ini" ("pattern (all files)")
                  n287 = call <vilib>:"Application Directory.vi"() -> ("Application Directory"=w437:path)
                  n288 = local read "工程代号"() -> (w435:string)
                  n289 = call "路径分析-8.6.vi"("第二个文件夹"="", "第一个文件夹"="ConfigFile", "输入路径"=w437) -> ("输出路径"=w433:path)  [unwired: 8 in]
                  n290 = Concatenate Strings(w435, "test" ("字符串"), w434) -> (w431:string)
                  n291 = Build Path(base path=w433, name or relative path=w431) -> (appended path=w432:path)
                  n292 = case shown="1" w440 {
                    tunnel: "选择要保存的位置" ("prompt") -> [_ w464]
                    tunnel: [w454 w463] -> w443
                    tunnel: [_ w461] -> w442
                    tunnel: w432 -> [w454 w460]
                    tunnel: w434 -> [_ w459]
                    frame 0, Default {
                    }
                    frame 1 {
                      n293 = local read "工程代号"() -> (w457:string)
                      n294 = Concatenate Strings(w457, "V0" ("字符串"), ".ini" ("pattern (all files)")) -> (w455:string)
                      n295 = call "文件对话框"("start path"=w460, "prompt"=w464, "default name"=w455, "pattern (all files)"=w459) -> ("selected path"=w463:path, "cancelled"=w461:bool, "error out"=w462:errorcluster)  [unwired: 8 in, 1 out]
                      n296 = call <vilib>:"Clear Errors.vi"("error in (no error)"=w462) -> ()  [unwired: 6 in, 1 out]
                    }
                  }
                  n297 = Insert Into Array(array=w447, index=0 ("索引"), new element="从板个数" ("新元素/子数组")) -> (w446:string[])
                  n298 = Insert Into Array(array=w446, new element #1=string[] ["总电压过高一级", "总电压过低一级", "温度过高一级", "温度过低一级", "整组电压不均衡一级", "单组电压不均衡一级", "整组温度不均衡一级", "单组温度不均衡一级", "单体电压过高一级", "单体电压过低一级", "充电电流过高一级", "放电电流过高一级", "SOC过高一级", "SOC过低一级", "内阻过大一级", "极柱温度过高一级", "SOH过低一级", "总电压过高二级", "总电压过低二级", "温度过高二级", "温度过低二级", "整组电压不均衡二级", "单组电压不均衡二级", "整组温度不均衡二级", "单组温度不均衡二级", "单体电压过高二级", "单体电压过低二级", "充电电流过高二级", "放电电流过高二级", "SOC过高二级", "SOC过低二级", "内阻过大二级", "极柱温度过高二级", "SOH过低二级", "总电压过高三级", "总电压过低三级", "温度过高三级", "温度过低三级", "整组电压不均衡三级", "单组电压不均衡三级", "整组温度不均衡三级", "单组温度不均衡三级", "单体电压过高三级", "单体电压过低三级", "充电电流过高三级", "放电电流过高三级", "SOC过高三级", "SOC过低三级", "内阻过大三级", "极柱温度过高三级", "SOH过低三级", "风机开启温度", "风机关闭温度", "加热开启温度", "加热关闭温度", "风机开启温差", "风机关闭温差", "加热关闭温差", "最大允许单体电压", "最小允许单体电压", "最大允许充电电流", "最小允许充电电流", "最大允许总电压", "最大允许充电温度", "最小允许充电温度", "电流步长"], new element #2=w449, new element #3="分流器型号") -> (w450:string[])  [unwired: 1 in]
                  n299 = case shown="假" w442 {
                    tunnel: w453 -> [w469 _]
                    tunnel: w450 -> [w468 _]
                    tunnel: [w467 _] -> w448
                    tunnel: w443 -> [w466 _]
                    tunnel: w441 -> [w465 _]
                    frame False {
                      n300 = call <vilib>:"Open Config Data.vi"("configuration file path"=w466) -> ("refnum"=w467:T11)  [unwired: 8 in, 2 out]
                      n301 = stacked-sequence {
                        tunnel: w469 -> [_ _ _ w487]
                        tunnel: w468 -> [_ _ _ w486]
                        tunnel: w467 -> [w473 w477 w482 w485]
                        tunnel: w465 -> [_ _ w479 _]
                        frame #0 {
                          n302 = local read "工号"() -> (w470:string)
                          n303 = call-poly <vilib>:"Write Key.vi"("section"="总信息" ("key"), "value"=w470, "key"="工号", "refnum"=w473) -> ()  [unwired: 5 in, 3 out]
                        }
                        frame #1 {
                          n304 = local read "工程代号"() -> (w474:string)
                          n305 = call-poly <vilib>:"Write Key.vi"("section"="总信息" ("key"), "value"=w474, "key"="工程代号", "refnum"=w477) -> ()  [unwired: 5 in, 3 out]
                        }
                        frame #2 {
                          n306 = case shown="1" w479 {
                            tunnel: ["MD5码" ("key") w484] -> w478
                            frame 0, Default {
                            }
                            frame 1 {
                              n307 = local read "MD5 message-digest"() -> (w484:string)
                            }
                          }
                          n308 = call-poly <vilib>:"Write Key.vi"("section"="总信息" ("key"), "value"=w478, "key"="MD5码", "refnum"=w482) -> ()  [unwired: 5 in, 3 out]
                        }
                        frame #3 {
                          n309 = for {
                            tunnel: w485 -> [w491]
                            tunnel: w487 -> [w490] mode=indexing
                            tunnel: w486 -> [w488] mode=indexing
                            n310 = call-poly <vilib>:"Write Key.vi"("section"="主板" ("key"), "value"=w490, "key"=w488, "refnum"=w491) -> ()  [unwired: 5 in, 3 out]
                          }
                        }
                      }
                    }
                    frame True {
                    }
                  }
                }
                frame #2 {
                  n311 = case shown="假" w493 {
                    tunnel: w496 -> [w497 _]
                    tunnel: w495 -> [w502 _]
                    tunnel: w494 -> [w501 _]
                    tunnel: w492 -> [w499 _]
                    frame False {
                      n312 = local read "输出数组"() -> (w503:string[][])
                      n313 = Transpose 2D Array(2D array=w503) -> (transposed array=w500:string[][])
                      n314 = for {
                        N: w502 -> [_]
                        tunnel: w500 -> [w527] mode=indexing
                        tunnel: w497 -> [w526]
                        tunnel: [w520] -> _
                        tunnel: [w519] -> w498
                        i -> [w525]
                        n315 = Increment(x=w525) -> (x+1=w524:i32)
                        n316 = Number To Decimal String(number=w524) -> (decimal integer string=w523:string)  [unwired: 1 in]
                        n317 = local read "从板表头"() -> (w518:string[])
                        n318 = Concatenate Strings("从板", w523) -> (w521:string)
                        n319 = for {
                          tunnel: w527 -> [w529] mode=indexing
                          tunnel: w526 -> [w533]
                          tunnel: w521 -> [w532]
                          tunnel: [w531] -> w520
                          tunnel: [w530] -> w519
                          tunnel: w518 -> [w528] mode=indexing
                          n320 = call-poly <vilib>:"Write Key.vi"("section"=w532, "value"=w529, "key"=w528, "refnum"=w533) -> ("error out"=w530:errorcluster, "refnum out"=w531:T11)  [unwired: 5 in, 1 out]
                        }
                      }
                      n321 = stacked-sequence {
                        tunnel: w498 -> [_ _ _]
                        tunnel: w501 -> [_ w507 w509]
                        tunnel: w499 -> [_ _ w508]
                        tunnel: w497 -> [w504 _ _]
                        frame #0 {
                          n322 = call <vilib>:"Close Config Data.vi"("refnum"=w504) -> ("error out"=w505:errorcluster)  [unwired: 9 in, 1 out]
                          n323 = call <vilib>:"Clear Errors.vi"("error in (no error)"=w505) -> ()  [unwired: 6 in, 1 out]
                        }
                        frame #1 {
                          n324 = call <vilib>:"MD5Checksum File.vi"("Path"=w507) -> ("MD5 message-digest"=→"MD5 message-digest":string)  [unwired: 9 in, 1 out]
                        }
                        frame #2 {
                          n325 = case shown="0, 默认" w508 {
                            tunnel: w509 -> [w510 w514]
                            frame 0, Default {
                              n326 = Delete(path (use dialog)=w510) -> (error out=w511:errorcluster)  [unwired: 4 in, 2 out]
                              n327 = call <vilib>:"Clear Errors.vi"("error in (no error)"=w511) -> ()  [unwired: 6 in, 1 out]
                            }
                            frame 1 {
                              n328 = Path To String(path=w514) -> (string=w513:string)
                              n329 = Concatenate Strings("保存完成，路径为：" ("按钮名称（“确定”）"), "\n", w513) -> (w512:string)
                              n330 = One Button Dialog(message=w512, button name ("OK")="确定" ("按钮名称（“确定”）")) -> ()  [unwired: 1 out]
                            }
                          }
                        }
                      }
                    }
                    frame True {
                    }
                  }
                }
              }
            }
            n331 = local write "MD5 message-digest"("" ("MD5 message-digest")) -> ()
          }
        }
      }
      event "预览": Value Change {
        n332 = event-data() -> ("NewVal"=w535:bool)  [unwired: 1 in, 5 out]
        n333 = case shown="真" w535 {
          tunnel: w534 -> [_ w536]
          frame False {
          }
          frame True {
            n334 = stacked-sequence {
              seq-local: [w564 _ _ _] -> [_ w612 _ _]
              seq-local: [w562 _ _ _] -> [_ w605 _ _]
              seq-local: [w560 _ _ _] -> [_ w606 _ _]
              seq-local: [w559 _ _ _] -> [_ _ w642 _]
              seq-local: [_ w599 _ _] -> [_ _ w638 _]
              tunnel: w536 -> [_ _ w635 _]
              frame #0 {
                n335 = local read "一级故障"() -> (w576:dbl[][])
                n336 = local read "充电控制参数"() -> (w540:T4)
                n337 = local read "主板信息"() -> (w577:string[][])
                n338 = local read "电池信息"() -> (w567:string[][])
                n339 = local read "加热控制参数"() -> (w573:T3)
                n340 = Array Subset(array=w577, index (row)=0 ("索引"), index (col)=0 ("索引"), length (col)=2 ("索引")) -> (w579:string[][])  [unwired: 1 in]
                n341 = Transpose 2D Array(2D array=w576) -> (transposed array=w558:dbl[][])
                n342 = for {
                  tunnel: w558 -> [w593] mode=indexing
                  shift-right: [w592] -> w552
                  shift-left: string[] [] -> [w590]
                  n343 = for {
                    N: 17 -> [_]
                    tunnel: w593 -> [w596] mode=indexing
                    tunnel: [w594] -> w591 mode=indexing
                    n344 = Format Into String(format string="%#f" ("格式字符串"), w596) -> (resulting string=w594:string)  [unwired: 2 in, 1 out]
                  }
                  n345 = Insert Into Array(array=w590, new element=w591) -> (w592:string[])  [unwired: 1 in]
                }
                n346 = Unbundle(w540) -> ("最大允许单体电压(V)"=w548:dbl, "最大允许总电压(V)"=w544:dbl, "最小允许单体电压(V)"=w547:dbl, "最大允许充电电流(A)"=w546:dbl, "最小允许充电电流(A)"=w545:dbl, "最大允许充电温度(℃)"=w543:dbl, "最小允许充电温度(℃)"=w542:dbl, "电流步长"=w541:dbl)
                n347 = Index Array(array=w579, index (col) #1=1 ("禁用的索引 (列)"), index (col) #2=0 ("索引 (列)")) -> (element #1=w557:string[], element #2=w562:string[])  [unwired: 2 in]
                n348 = local read "从板个数"() -> (w559:dbl)
                n349 = Array Subset(array=w567, index (row)=0 ("索引"), index (col)=0 ("索引"), length (col)=2 ("索引")) -> (w571:string[][])  [unwired: 1 in]
                n350 = Cluster To Array(cluster=w573) -> (array=w574:dbl[])
                n351 = local read "分流器型号"() -> (w538:T2)
                n352 = for {
                  tunnel: w574 -> [w588] mode=indexing
                  tunnel: [w586] -> w556 mode=indexing
                  n353 = Format Into String(format string="%#f" ("格式字符串"), w588) -> (resulting string=w586:string)  [unwired: 2 in, 1 out]
                }
                n354 = Build Array(w548, w547, w546, w545, w544, w543, w542, w541) -> (w539:dbl[])
                n355 = Index Array(array=w571, index (col) #1=0 ("禁用的索引 (列)"), index (col) #2=1 ("禁用的索引 (列)")) -> (element #1=w560:string[], element #2=w554:string[])  [unwired: 2 in]
                n356 = for {
                  tunnel: w539 -> [w585] mode=indexing
                  tunnel: [w583] -> w555 mode=indexing
                  n357 = Format Into String(format string="%#f" ("格式字符串"), w585) -> (resulting string=w583:string)  [unwired: 2 in, 1 out]
                }
                n358 = Number To Decimal String(number=w559) -> (decimal integer string=w566:string)  [unwired: 1 in]
                n359 = Number To Decimal String(number=w538) -> (decimal integer string=w537:string)  [unwired: 1 in]
                n360 = Array Subset(array=w552, index=0 ("索引"), length=51 ("长度")) -> (w549:string[])
                n361 = Insert Into Array(array=w557, new element #1=w549, new element #2=w556, new element #3=w555, new element #4=w554, new element #5=w537) -> (w553:string[])  [unwired: 1 in]
                n362 = Insert Into Array(array=w553, index=0 ("索引"), new element=w566) -> (w564:string[])
              }
              frame #1 {
                n363 = call <vilib>:"Application Directory.vi"() -> ("Application Directory"=w613:path)
                n364 = local read "工程代号"() -> (w610:string)
                n365 = call "路径分析-8.6.vi"("第二个文件夹"="", "第一个文件夹"="ConfigFile", "输入路径"=w613) -> ("输出路径"=w600:path)  [unwired: 8 in]
                n366 = Concatenate Strings(w610, "-rc" ("字符串"), ".ini" ("pattern (all files)")) -> (w601:string)
                n367 = Build Path(base path=w600, name or relative path=w601) -> (appended path=w599:path)
                n368 = call <vilib>:"Open Config Data.vi"("configuration file path"=w599) -> ("refnum"=w598:T11)  [unwired: 8 in, 2 out]
                n369 = Insert Into Array(array=w605, index=0 ("索引"), new element="从板个数" ("新元素/子数组")) -> (w604:string[])
                n370 = Insert Into Array(array=w604, new element #1=string[] ["总电压过高一级", "总电压过低一级", "温度过高一级", "温度过低一级", "整组电压不均衡一级", "单组电压不均衡一级", "整组温度不均衡一级", "单组温度不均衡一级", "单体电压过高一级", "单体电压过低一级", "充电电流过高一级", "放电电流过高一级", "SOC过高一级", "SOC过低一级", "内阻过大一级", "极柱温度过高一级", "SOH过低一级", "总电压过高二级", "总电压过低二级", "温度过高二级", "温度过低二级", "整组电压不均衡二级", "单组电压不均衡二级", "整组温度不均衡二级", "单组温度不均衡二级", "单体电压过高二级", "单体电压过低二级", "充电电流过高二级", "放电电流过高二级", "SOC过高二级", "SOC过低二级", "内阻过大二级", "极柱温度过高二级", "SOH过低二级", "总电压过高三级", "总电压过低三级", "温度过高三级", "温度过低三级", "整组电压不均衡三级", "单组电压不均衡三级", "整组温度不均衡三级", "单组温度不均衡三级", "单体电压过高三级", "单体电压过低三级", "充电电流过高三级", "放电电流过高三级", "SOC过高三级", "SOC过低三级", "内阻过大三级", "极柱温度过高三级", "SOH过低三级", "风机开启温度", "风机关闭温度", "加热开启温度", "加热关闭温度", "风机开启温差", "风机关闭温差", "加热关闭温差", "最大允许单体电压", "最小允许单体电压", "最大允许充电电流", "最小允许充电电流", "最大允许总电压", "最大允许充电温度", "最小允许充电温度", "电流步长"], new element #2=w606, new element #3="分流器型号") -> (w607:string[])  [unwired: 1 in]
                n371 = stacked-sequence {
                  tunnel: w612 -> [_ _ w628]
                  tunnel: w607 -> [_ _ w627]
                  tunnel: w598 -> [w616 w620 w626]
                  frame #0 {
                    n372 = local read "工号"() -> (w617:string)
                    n373 = call-poly <vilib>:"Write Key.vi"("section"="总信息" ("key"), "value"=w617, "key"="工号", "refnum"=w616) -> ()  [unwired: 5 in, 3 out]
                  }
                  frame #1 {
                    n374 = local read "工程代号"() -> (w621:string)
                    n375 = call-poly <vilib>:"Write Key.vi"("section"="总信息" ("key"), "value"=w621, "key"="工程代号", "refnum"=w620) -> ()  [unwired: 5 in, 3 out]
                  }
                  frame #2 {
                    n376 = for {
                      tunnel: w626 -> [w634]
                      tunnel: w628 -> [w633] mode=indexing
                      tunnel: w627 -> [w631] mode=indexing
                      tunnel: [w630] -> w625
                      tunnel: [w629] -> w624
                      n377 = call-poly <vilib>:"Write Key.vi"("section"="主板" ("key"), "value"=w633, "key"=w631, "refnum"=w634) -> ("error out"=w629:errorcluster, "refnum out"=w630:T11)  [unwired: 5 in, 1 out]
                    }
                    n378 = call <vilib>:"Close Config Data.vi"("error in (no error)"=w624, "refnum"=w625) -> ()  [unwired: 8 in, 2 out]
                  }
                }
              }
              frame #2 {
                n379 = local read "输出数组"() -> (w641:string[][])
                n380 = Transpose 2D Array(2D array=w641) -> (transposed array=w640:string[][])
                n381 = call <vilib>:"Open Config Data.vi"("configuration file path"=w638) -> ("refnum"=w637:T11)  [unwired: 8 in, 2 out]
                n382 = for {
                  N: w642 -> [_]
                  tunnel: w640 -> [w652] mode=indexing
                  tunnel: w637 -> [w651]
                  tunnel: [w645] -> w636
                  tunnel: [w644] -> w639
                  tunnel: w635 -> [w643]
                  i -> [w650]
                  n383 = Increment(x=w650) -> (x+1=w649:i32)
                  n384 = Number To Decimal String(number=w649) -> (decimal integer string=w648:string)  [unwired: 1 in]
                  n385 = Concatenate Strings("从板", w648) -> (w646:string)
                  n386 = for {
                    tunnel: w652 -> [w654] mode=indexing
                    tunnel: w651 -> [w658]
                    tunnel: w646 -> [w657]
                    tunnel: [w656] -> w645
                    tunnel: [w655] -> w644
                    tunnel: w643 -> [w653] mode=indexing
                    n387 = call-poly <vilib>:"Write Key.vi"("section"=w657, "value"=w654, "key"=w653, "refnum"=w658) -> ("error out"=w655:errorcluster, "refnum out"=w656:T11)  [unwired: 5 in, 1 out]
                  }
                }
                n388 = stacked-sequence {
                  tunnel: w638 -> [_ w662 _]
                  tunnel: w639 -> [_ _ _]
                  tunnel: w636 -> [w659 _ _]
                  frame #0 {
                    n389 = call <vilib>:"Close Config Data.vi"("refnum"=w659) -> ("error out"=w660:errorcluster)  [unwired: 9 in, 1 out]
                    n390 = call <vilib>:"Clear Errors.vi"("error in (no error)"=w660) -> ()  [unwired: 6 in, 1 out]
                  }
                  frame #1 {
                    n391 = Open/Create/Replace File(file path (use dialog)=w662) -> (refnum out=w669:refnum<file>, error out=w668:errorcluster)  [unwired: 5 in, 1 out]
                    n392 = Read from Text File(file (use dialog)=w669, error in=w668) -> (refnum out=w666:refnum<file>, text=w667:string, error out=w665:errorcluster)  [unwired: 2 in, 1 out]
                    n393 = call "预览结果显示.vi"("预览结果"=w667) -> ()  [unwired: 1 out]
                    n394 = Close File(refnum=w666, error in=w665) -> (error out=w663:errorcluster)  [unwired: 1 out]
                    n395 = local write "预览"(FALSE ("预览")) -> ()
                    n396 = Delete(path (use dialog)=w662, error in=w663) -> (error out=w661:errorcluster)  [unwired: 3 in, 2 out]
                    n397 = call <vilib>:"Clear Errors.vi"("error in (no error)"=w661) -> ()  [unwired: 6 in, 1 out]
                  }
                  frame #2 {
                    n398 = disable-structure shown="禁用" {
                      disable-tunnel: _ -> [w672 _]
                      frame Disabled {
                        n399 = Path To String(path=w672) -> (string=w671:string)
                        n400 = Concatenate Strings("保存完成，路径为：" ("按钮名称（“确定”）"), "\n", w671) -> (w670:string)
                        n401 = One Button Dialog(message=w670, button name ("OK")="确定" ("按钮名称（“确定”）")) -> ()  [unwired: 1 out]
                      }
                      frame Enabled {
                      }
                    }
                  }
                }
              }
              frame #3 {
              }
            }
          }
        }
      }
      event "读取(ini)": Value Change {
        n402 = event-data() -> ("NewVal"=w676:bool)  [unwired: 1 in, 5 out]
        n403 = case shown="真" w676 {
          frame False {
          }
          frame True {
            n404 = stacked-sequence {
              seq-local: [w689 _ _ _ _] -> [_ w747 w821 _ _]
              seq-local: [w679 _ _ _ _] -> [_ w746 w819 w910 w952]
              seq-local: [_ w745 _ _ _] -> [_ _ _ _ w951]
              frame #0 {
                n405 = global read "配置文件全局.vi" "参数生成器读取地址"() -> (w678:path)
                n406 = call "文件对话框"("start path"=w678, "prompt"="选择要读取的文件") -> ("selected path"=w683:path, "cancelled"=w682:bool, "error out"=w688:errorcluster)  [unwired: 10 in, 1 out]
                n407 = Strip Path(path=w683) -> (stripped path=w677:path, name=w687:string)
                n408 = global write "配置文件全局.vi" "参数生成器读取地址"(w677) -> ()
                n409 = Match Pattern(string=w687, regular expression=".ini" ("正则表达式")) -> (offset past match=w685:i32)  [unwired: 1 in, 3 out]
                n410 = Equal?(x=w685, y=-1) -> (x = y?=w681:bool)
                n411 = case shown="假" w681 {
                  tunnel: w683 -> [w703 _]
                  tunnel: [w691 _] -> w680
                  frame False {
                    w714 = "MD5码" ("key")
                    w715 = "总信息" ("section")
                    n412 = Strip Path(path=w703) -> (stripped path=w701:path, name=w700:string)
                    n413 = Match Pattern(string=w700, regular expression=".ini" ("正则表达式")) -> (before substring=w697:string, match substring=w698:string)  [unwired: 1 in, 2 out]
                    n414 = Concatenate Strings(w697, "-rc" ("字符串"), w698) -> (w696:string)
                    n415 = Build Path(base path=w701, name or relative path=w696) -> (appended path=w702:path)
                    n416 = Copy(10:w702, 11:w703) -> (3:w707:path)  [unwired: 3 in, 2 out]
                    n417 = call <vilib>:"Open Config Data.vi"("create file if necessary (T)"=FALSE, "configuration file path"=w707) -> ("refnum"=w717:T11)  [unwired: 7 in, 2 out]
                    n418 = call-poly <vilib>:"Read Key.vi"("section"=w715, "key"=w714, "refnum"=w717) -> ("value"=w694:string, "refnum out"=w716:T11)  [unwired: 5 in, 2 out]
                    n419 = call-poly <vilib>:"Write Key.vi"("section"=w715, "value"=w714, "key"=w714, "refnum"=w716) -> ("error out"=w711:errorcluster, "found?"=w710:bool, "refnum out"=w709:T11)  [unwired: 5 in]
                    n420 = call <vilib>:"Close Config Data.vi"("error in (no error)"=w711, "write file if changed (T)"=w710, "refnum"=w709) -> ("error out"=w708:errorcluster, "file path"=w705:path)  [unwired: 7 in]
                    n421 = call <vilib>:"MD5Checksum File.vi"("error in (no error)"=w708, "Path"=w705) -> ("error out"=w706:errorcluster, "MD5 message-digest"=w713:string)  [unwired: 8 in]
                    n422 = for {
                      N: 2 -> [_]
                      tunnel: w713 -> [w722]
                      tunnel: [w721] -> w712 mode=indexing
                      tunnel: w694 -> [w720]
                      i -> [w719]
                      n423 = case shown="1" w719 {
                        tunnel: w722 -> [w726 w727]
                        tunnel: [w725 w729] -> w721
                        tunnel: w720 -> [w724 w728]
                        frame 0, Default {
                          n424 = To Upper Case(1:w726) -> (0:w723:string)
                          n425 = Equal?(x=w723, y=w724) -> (x = y?=w725:bool)
                        }
                        frame 1 {
                          n426 = Equal?(x=w727, y=w728) -> (x = y?=w729:bool)
                        }
                      }
                    }
                    n427 = Or Array Elements(Boolean array=w712) -> (logical OR=w692:bool)
                    n428 = Not(x=w692) -> (.not. x?=w691:bool)
                    n429 = Delete(path (use dialog)=w705, error in=w706) -> (error out=w704:errorcluster)  [unwired: 3 in, 2 out]
                    n430 = call <vilib>:"Clear Errors.vi"("error in (no error)"=w704) -> ()  [unwired: 6 in, 1 out]
                  }
                  frame True {
                  }
                }
                n431 = call <vilib>:"Clear Errors.vi"("error in (no error)"=w688) -> ()  [unwired: 6 in, 1 out]
                n432 = Compound Arithmetic op=OR(w682, w681, w680) -> (w679:bool)
                n433 = case shown="真" w679 {
                  tunnel: w683 -> [w734 _]
                  tunnel: [w733 _] -> w689
                  frame False {
                    w736 = "总信息" ("section")
                    n434 = call <vilib>:"Open Config Data.vi"("create file if necessary (T)"=FALSE, "configuration file path"=w734) -> ("refnum"=w733:T11)  [unwired: 7 in, 2 out]
                    n435 = call <vilib>:"Get Key Names.vi"("section"=w736, "refnum"=w733) -> ("key names"=w735:string[], "refnum out"=w737:T11)  [unwired: 6 in, 2 out]
                    n436 = for {
                      tunnel: w737 -> [w742]
                      tunnel: w736 -> [w741]
                      tunnel: w735 -> [w740] mode=indexing
                      tunnel: [w739] -> w732 mode=indexing
                      n437 = call-poly <vilib>:"Read Key.vi"("section"=w741, "key"=w740, "refnum"=w742) -> ("value"=w739:string)  [unwired: 5 in, 3 out]
                    }
                    n438 = Index Array(array=w732) -> (element #1=w731:string, element #2=w730:string)  [unwired: 2 in]
                    n439 = local write "工程代号"(w730) -> ()
                    n440 = local write "工号"(w731) -> ()
                  }
                  frame True {
                    n441 = One Button Dialog(message="文件格式错误或文件不正确" ("消息"), button name ("OK")="确定" ("按钮名称（“确定”）")) -> ()  [unwired: 1 out]
                  }
                }
              }
              frame #1 {
                n442 = case shown="假" w746 {
                  tunnel: w747 -> [w772 _]
                  tunnel: [w766 _] -> w745
                  frame False {
                    w776 = 15 ("长度")
                    w808 = "主板" ("section")
                    n443 = call <vilib>:"Get Key Names.vi"("section"=w808, "refnum"=w772) -> ("key names"=w752:string[], "refnum out"=w809:T11)  [unwired: 6 in, 2 out]
                    n444 = for {
                      tunnel: w809 -> [w817]
                      tunnel: w808 -> [w816]
                      tunnel: w752 -> [w815] mode=indexing
                      tunnel: [w814] -> w751 mode=indexing
                      n445 = call-poly <vilib>:"Read Key.vi"("section"=w816, "key"=w815, "refnum"=w817) -> ("value"=w814:string)  [unwired: 5 in, 3 out]
                    }
                    n446 = Search 1D Array(1D array=w752, element="总电压过高一级" ("元素"), start index (0)=0 ("开始索引(0)")) -> (index of element=w785:i32)
                    n447 = Search 1D Array(1D array=w752, element="风机开启温度" ("元素"), start index (0)=w785) -> (index of element=w786:i32)
                    n448 = Search 1D Array(1D array=w752, element="电池串联" ("元素"), start index (0)=w785) -> (index of element=w777:i32)
                    n449 = Search 1D Array(1D array=w752, element="分流器型号" ("元素")) -> (index of element=w750:i32)  [unwired: 1 in]
                    n450 = Decrement(x=w785) -> (x-1=w771:i32)
                    n451 = Index Array(array=w751, index=w750) -> (element=w749:string)
                    n452 = Array Subset(array=w751, index=w786, length=15 ("长度")) -> (w781:string[])
                    n453 = Array Subset(array=w751, index=w785, length=51 ("长度")) -> (w799:string[])
                    n454 = Array Subset(array=w751, index=w777, length=w776) -> (w774:string[])
                    n455 = Array Subset(array=w752, index=1 ("索引"), length=w771) -> (w803:string[])
                    n456 = Array Subset(array=w752, index=w777, length=w776) -> (w775:string[])
                    n457 = Array Subset(array=w751, index=1 ("索引"), length=w771) -> (w802:string[])
                    n458 = Index Array(array=w751, index=0 ("索引")) -> (element=w769:string)
                    n459 = for {
                      tunnel: w799 -> [w813] mode=indexing
                      tunnel: [w812] -> w798 mode=indexing
                      n460 = Fract/Exp String To Number(string=w813) -> (number=w812:dbl)  [unwired: 3 in, 1 out]
                    }
                    n461 = for {
                      tunnel: w781 -> [w811] mode=indexing
                      tunnel: [w810] -> w780 mode=indexing
                      n462 = Fract/Exp String To Number(string=w811) -> (number=w810:dbl)  [unwired: 3 in, 1 out]
                    }
                    n463 = Decimal String To Number(string=w749) -> (number=w748:i32)  [unwired: 2 in, 1 out]
                    n464 = Build Array(w803, w802) -> (w801:string[][])
                    n465 = Decimal String To Number(string=w769) -> (number=w766:i32)  [unwired: 2 in, 1 out]
                    n466 = Build Array(w775, w774) -> (w773:string[][])
                    n467 = local write "分流器型号"(w748) -> ()
                    n468 = Transpose 2D Array(2D array=w801) -> (transposed array=w768:string[][])
                    n469 = Transpose 2D Array(2D array=w773) -> (transposed array=w767:string[][])
                    n470 = Delete From Array(array=w798, length=17 ("长度"), index=0 ("索引")) -> (deleted portion=w795:dbl[], array with subset deleted=w794:dbl[])
                    n471 = Delete From Array(array=w780, length=7 ("长度"), index=0 ("索引")) -> (deleted portion=w779:dbl[], array with subset deleted=w764:dbl[])
                    n472 = local write "主板信息"(w768) -> ()
                    n473 = Delete From Array(array=w794, length=17 ("长度"), index=0 ("索引")) -> (deleted portion=w765:dbl[], array with subset deleted=w791:dbl[])
                    n474 = local write "电池信息"(w767) -> ()
                    n475 = local write "从板个数"(w766) -> ()
                    n476 = Array To Cluster(array=w779) -> (cluster=w778:T10)
                    n477 = Build Array(w795, w765, w791) -> (w790:dbl[][])
                    n478 = Index Array(array=w764) -> (element #1=w761:dbl, element #2=w759:dbl, element #3=w758:dbl, element #4=w757:dbl, element #5=w760:dbl, element #6=w756:dbl, element #7=w755:dbl, element #8=w754:dbl)  [unwired: 8 in]
                    n479 = local write "加热控制参数"(w778) -> ()
                    n480 = Transpose 2D Array(2D array=w790) -> (transposed array=w789:dbl[][])
                    n481 = Build Array(w761, w760, w759, w758, w757, w756, w755, w754) -> (w762:dbl[])
                    n482 = local write "一级故障"(w789) -> ()
                    n483 = Array To Cluster(array=w762) -> (cluster=w763:T12)
                    n484 = local write "充电控制参数"(w763) -> ()
                  }
                  frame True {
                  }
                }
              }
              frame #2 {
                n485 = case shown="假" w819 {
                  tunnel: w821 -> [w888 _]
                  frame False {
                    w823 = string[] ["从板板号", "电压个数", "温度个数", "第一个保险通道", "第一个保险位置", "第二个保险通道", "第二个保险位置", "第三个保险通道", "第三个保险位置", "第四个保险通道", "第四个保险位置", "第五个保险通道", "第五个保险位置", "第六个保险通道", "第六个保险位置", "第七个保险通道", "第七个保险位置", "第八个保险通道", "第八个保险位置", "第九个保险通道", "第九个保险位置", "第十个保险通道", "第十个保险位置", "第1通道电压个数", "第2通道电压个数", "第3通道电压个数", "第4通道电压个数", "第5通道电压个数", "风机开启温度", "风机关闭温度", "加热开启温度", "加热关闭温度", "风机开启温差", "风机关闭温差", "加热关闭温差", "电压过高一级", "电压过低一级", "温度过高一级", "温度过低一级", "电压不均衡一级", "温度不均衡一级", "SOC过低一级", "电压过高二级", "电压过低二级", "温度过高二级", "温度过低二级", "电压不均衡二级", "温度不均衡二级", "SOC过低二级", "电压过高三级", "电压过低三级", "温度过高三级", "温度过低三级", "电压不均衡三级", "温度不均衡三级", "SOC过低三级", "均衡计算-电压高阀值1级", "均衡计算-电压高阀值2级", "均衡计算-电压低阀值1级", "均衡计算-电压低阀值2级", "均衡计算-最低电压阀值", "均衡停止-最低电压阀值", "均衡计算-电压极差阀值", "充电结束电压(90%)", "充电结束电压(91%)", "充电结束电压(92%)", "充电结束电压(93%)", "充电结束电压(94%)", "充电结束电压(95%)", "充电结束电压(96%)", "充电结束电压(97%)", "充电结束电压(98%)", "充电结束电压(99%)", "充电结束电压(100%)"] ("从板表头")
                    (unwired) string[] ["从板板号", "电压个数", "电压起始值", "温度个数", "温度起始值", "第一个保险通道", "第一个保险位置", "第二个保险通道", "第二个保险位置", "第三个保险通道", "第三个保险位置", "第四个保险通道", "第四个保险位置", "第五个保险通道", "第五个保险位置", "第六个保险通道", "第六个保险位置", "第七个保险通道", "第七个保险位置", "第八个保险通道", "第八个保险位置", "第九个保险通道", "第九个保险位置", "第十个保险通道", "第十个保险位置", "第1通道电压个数", "第2通道电压个数", "第3通道电压个数", "第4通道电压个数", "第5通道电压个数", "第6通道电压个数", "第7通道电压个数", "第8通道电压个数", "第9通道电压个数", "第10通道电压个数", "第11通道电压个数", "第12通道电压个数", "第13通道电压个数", "第14通道电压个数", "第15通道电压个数", "第16通道电压个数", "第17通道电压个数", "第18通道电压个数", "第19通道电压个数", "第20通道电压个数", "风机开启温度", "风机关闭温度", "加热开启温度", "加热关闭温度", "风机开启温差", "风机关闭温差", "加热关闭温差", "电压过高一级", "电压过低一级", "温度过高一级", "温度过低一级", "电压不均衡一级", "温度不均衡一级", "SOC过低一级", "电压过高二级", "电压过低二级", "温度过高二级", "温度过低二级", "电压不均衡二级", "温度不均衡二级", "SOC过低二级", "电压过高三级", "电压过低三级", "温度过高三级", "温度过低三级", "电压不均衡三级", "温度不均衡三级", "SOC过低三级", "均衡计算-电压高阀值1级", "均衡计算-电压高阀值2级", "均衡计算-电压低阀值1级", "均衡计算-电压低阀值2级", "均衡计算-最低电压阀值", "均衡停止-最低电压阀值", "均衡计算-电压极差阀值", "充电结束电压(90%)", "充电结束电压(91%)", "充电结束电压(92%)", "充电结束电压(93%)", "充电结束电压(94%)", "充电结束电压(95%)", "充电结束电压(96%)", "充电结束电压(97%)", "充电结束电压(98%)", "充电结束电压(99%)", "充电结束电压(100%)"] ("从板表头")
                    w880 = 1 ("索引")
                    n486 = call <vilib>:"Get Section Names.vi"("refnum"=w888) -> ("section names"=w887:string[], "refnum out"=w883:T11)  [unwired: 8 in, 1 out]
                    n487 = local read "从板板号"() -> (w857:dbl)
                    n488 = Delete From Array(array=w887, length=2 ("长度"), index=0 ("索引")) -> (array with subset deleted=w884:string[])  [unwired: 1 out]
                    n489 = Decrement(x=w857) -> (x-1=w855:dbl)
                    n490 = for {
                      tunnel: w884 -> [w904] mode=indexing
                      tunnel: w883 -> [w905]
                      tunnel: [w897] -> w882 mode=indexing
                      tunnel: [w896] -> w850
                      n491 = call <vilib>:"Get Key Names.vi"("section"=w904, "refnum"=w905) -> ("key names"=w896:string[], "refnum out"=w903:T11)  [unwired: 6 in, 2 out]
                      n492 = for {
                        tunnel: w896 -> [w909] mode=indexing
                        tunnel: w904 -> [w908]
                        tunnel: w903 -> [w907]
                        tunnel: [w906] -> w897 mode=indexing
                        n493 = call-poly <vilib>:"Read Key.vi"("section"=w908, "key"=w909, "refnum"=w907) -> ("value"=w906:string)  [unwired: 5 in, 3 out]
                      }
                      n494 = Index Array(array=w897, index=0 ("索引")) -> (element=w900:string)
                      n495 = local read "输出数组"() -> (w901:string[][])
                      n496 = Decimal String To Number(string=w900) -> (number=w899:i32)  [unwired: 2 in, 1 out]
                      n497 = Decrement(x=w899) -> (x-1=w895:i32)
                      n498 = Replace Array Subset(array=w901, new element=w897, index (col)=w895) -> (w898:string[][])  [unwired: 1 in]
                      n499 = local write "输出数组"(w898) -> ()
                    }
                    n500 = Index Array(array=w882, index (row)=w855) -> (element=w849:string[])  [unwired: 1 in]
                    n501 = Search 1D Array(1D array=w850, element="风机开启温度" ("元素")) -> (index of element=w875:i32)  [unwired: 1 in]
                    n502 = Search 1D Array(1D array=w850, element="电压过高一级" ("元素"), start index (0)=w875) -> (index of element=w851:i32)
                    n503 = Search 1D Array(1D array=w850, element="均衡计算-电压高阀值1级" ("元素"), start index (0)=w851) -> (index of element=w853:i32)
                    n504 = Decrement(x=w875) -> (x-1=w877:i32)
                    n505 = Array Subset(array=w849, index=w880, length=27 ("长度")) -> (w879:string[])
                    n506 = Array Subset(array=w849, index=w851, length=21 ("长度")) -> (w861:string[])
                    n507 = Array Subset(array=w850, index=w880, length=w877) -> ()  [unwired: 1 out]
                    n508 = Array Subset(array=w849, index=w875, length=7 ("长度")) -> (w872:string[])
                    n509 = Array Subset(array=w849, index=w853, length=17 ("长度")) -> (w852:string[])
                    n510 = for {
                      tunnel: w861 -> [w892] mode=indexing
                      tunnel: [w891] -> w860 mode=indexing
                      n511 = Fract/Exp String To Number(string=w892) -> (number=w891:dbl)  [unwired: 3 in, 1 out]
                    }
                    n512 = for {
                      tunnel: w872 -> [w894] mode=indexing
                      tunnel: [w893] -> w871 mode=indexing
                      n513 = Fract/Exp String To Number(string=w894) -> (number=w893:dbl)  [unwired: 3 in, 1 out]
                    }
                    n514 = for {
                      tunnel: w852 -> [w890] mode=indexing
                      tunnel: [w889] -> w829 mode=indexing
                      n515 = Fract/Exp String To Number(string=w890) -> (number=w889:dbl)  [unwired: 3 in, 1 out]
                    }
                    n516 = Array Subset(array=w823, index=1 ("长度"), length=27 ("长度")) -> (w826:string[])
                    n517 = Build Array(w826, w879) -> (w878:string[][])
                    n518 = local write "从板表头"(w823) -> ()
                    n519 = Delete From Array(array=w860, length=7 ("长度"), index=0 ("索引")) -> (deleted portion=w867:dbl[], array with subset deleted=w866:dbl[])
                    n520 = Array To Cluster(array=w871) -> (cluster=w870:T10)
                    n521 = Transpose 2D Array(2D array=w878) -> (transposed array=w858:string[][])
                    n522 = Delete From Array(array=w866, length=7 ("长度"), index=0 ("索引")) -> (deleted portion=w863:dbl[], array with subset deleted=w862:dbl[])
                    n523 = local write "加热控制参数 2"(w870) -> ()
                    n524 = Build Array(w867, w863, w862) -> (w859:dbl[][])
                    n525 = Transpose 2D Array(2D array=w859) -> (transposed array=w856:dbl[][])
                    n526 = local write "从板信息电压温度通道配置"(w858) -> ()
                    n527 = Index Array(array=w829) -> (element #1=w847:dbl, element #2=w846:dbl, element #3=w845:dbl, element #4=w844:dbl, element #5=w843:dbl, element #6=w842:dbl, element #7=w841:dbl, element #8=w840:dbl, element #9=w839:dbl, element #10=w838:dbl, element #11=w837:dbl, element #12=w836:dbl, element #13=w835:dbl, element #14=w834:dbl, element #15=w833:dbl, element #16=w832:dbl, element #17=w831:dbl, element #18=w830:dbl)  [unwired: 18 in]
                    n528 = local write "一级故障 2"(w856) -> ()
                    n529 = local read "均衡参数"() -> (w827:T1)
                    n530 = Bundle(cluster=w827, "充电结束电压(90%)"=w840, "充电结束电压(91%)"=w839, "充电结束电压(92%)"=w838, "充电结束电压(93%)"=w837, "充电结束电压(94%)"=w836, "均衡计算-电压高阀值1级"=w847, "均衡计算-电压高阀值2级"=w846, "均衡计算-电压低阀值1级"=w845, "均衡计算-电压低阀值2级"=w844, "均衡计算-最低电压阀值"=w843, "均衡停止-最低电压阀值"=w842, "均衡计算-电压极差阀值"=w841, "充电结束电压(95%)"=w835, "充电结束电压(96%)"=w834, "充电结束电压(97%)"=w833, "充电结束电压(98%)"=w832, "充电结束电压(99%)"=w831, "充电结束电压(100%)"=w830) -> (w828:T1)
                    n531 = local write "均衡参数"(w828) -> ()
                  }
                  frame True {
                  }
                }
                n532 = local write "读取(ini)"(FALSE ("读取")) -> ()
                n533 = local write "布尔"(TRUE ("布尔")) -> ()
              }
              frame #3 {
                n534 = case shown="假" w910 {
                  frame False {
                    w919 = bool[][] [[FALSE, FALSE, FALSE, FALSE, FALSE, FALSE, FALSE, FALSE, FALSE, FALSE, FALSE, FALSE], [FALSE, FALSE, FALSE, FALSE, FALSE, FALSE, FALSE, FALSE, FALSE, FALSE, FALSE, FALSE], [FALSE, FALSE, FALSE, FALSE, FALSE, FALSE, FALSE, FALSE, FALSE, FALSE, FALSE, FALSE], [FALSE, FALSE, FALSE, FALSE, FALSE, FALSE, FALSE, FALSE, FALSE, FALSE, FALSE, FALSE], [FALSE, FALSE, FALSE, FALSE, FALSE, FALSE, FALSE, FALSE, FALSE, FALSE, FALSE, FALSE], [FALSE, FALSE, FALSE, FALSE, FALSE, FALSE, FALSE, FALSE, FALSE, FALSE, FALSE, FALSE], [FALSE, FALSE, FALSE, FALSE, FALSE, FALSE, FALSE, FALSE, FALSE, FALSE, FALSE, FALSE], [FALSE, FALSE, FALSE, FALSE, FALSE, FALSE, FALSE, FALSE, FALSE, FALSE, FALSE, FALSE], [FALSE, FALSE, FALSE, FALSE, FALSE, FALSE, FALSE, FALSE, FALSE, FALSE, FALSE, FALSE], [FALSE, FALSE, FALSE, FALSE, FALSE, FALSE, FALSE, FALSE, FALSE, FALSE, FALSE, FALSE]]
                    n535 = local read "从板信息电压温度通道配置"() -> (w918:string[][])
                    n536 = Index Array(array=w918, index (col)=1 ("禁用的索引 (列)")) -> (element=w913:string[])  [unwired: 1 in]
                    n537 = Array Subset(array=w913, index=4 ("索引"), length=20 ("长度")) -> (w926:string[])
                    n538 = Array Subset(array=w913, index=24 ("索引"), length=20 ("长度")) -> (w915:string[])
                    n539 = for {
                      tunnel: w915 -> [w931] mode=indexing
                      tunnel: [w930] -> w914 mode=indexing
                      n540 = Fract/Exp String To Number(string=w931, default (0 dbl)=u8 0) -> (number=w930:u8)  [unwired: 2 in, 1 out]
                    }
                    n541 = for {
                      tunnel: w926 -> [w950] mode=indexing
                      shift-right: [w947] -> w920
                      shift-left: i32[] [] -> [w946]
                      n542 = Fract/Exp String To Number(string=w950, default (0 dbl)=u8 0) -> (number=w945:u8)  [unwired: 2 in, 1 out]
                      n543 = Equal To 0?(x=w945) -> (x = 0?=w948:bool)
                      n544 = Insert Into Array(array=w946, new element=w945) -> (w944:i32[])  [unwired: 1 in]
                      n545 = Select(t=w946, s=w948, f=w944) -> (s? t:f=w947:i32[])
                    }
                    n546 = Array Subset(array=w914, length=20 ("维数大小")) -> (w912:u8[])  [unwired: 1 in]
                    n547 = local write "5个通道电压个数(最小5个)"(w912) -> ()
                    n548 = Array Size(array=w920) -> (size(s)=w923:i32)
                    n549 = Quotient & Remainder(x=w923, y=2) -> (floor(x/y)=w921:i32)  [unwired: 1 out]
                    n550 = for {
                      N: w921 -> [_]
                      tunnel: w920 -> [w935]
                      tunnel: w919 -> [_]
                      i -> [w934]
                      n551 = Multiply(x=w934, y=2) -> (x*y=w942:i32)
                      n552 = Increment(x=w942) -> (x+1=w941:i32)
                      n553 = Index Array(array=w935, index #1=w942, index #2=w941) -> (element #1=w940:i32, element #2=w939:i32)
                      n554 = local read "保险位置"() -> (w932:T6)
                      n555 = Decrement(x=w940) -> (x-1=w937:i32)
                      n556 = Decrement(x=w939) -> (x-1=w936:i32)
                      n557 = Replace Array Subset(array=w932, new element=TRUE, index (row)=w937, index (col)=w936) -> (w933:T6)
                      n558 = local write "保险位置"(w933) -> ()
                    }
                    n559 = local write "保险位置"(w919) -> ()
                  }
                  frame True {
                  }
                }
              }
              frame #4 {
                n560 = case shown="假" w952 {
                  tunnel: w951 -> [w957 _]
                  frame False {
                    n561 = local write "自动记录"(TRUE ("自动记录")) -> ()
                    n562 = Number To Decimal String(number=w957) -> (decimal integer string=w956:string)  [unwired: 1 in]
                    n563 = Concatenate Strings("读取完成，配置文件为 一主" ("字符串"), w956, "从" ("字符串")) -> (w959:string)
                    n564 = One Button Dialog(message=w959, button name ("OK")="确定" ("按钮名称（“确定”）")) -> ()  [unwired: 1 out]
                  }
                  frame True {
                  }
                }
              }
            }
          }
        }
      }
      event "默认值": Value Change {
        n565 = event-data() -> ("NewVal"=w960:bool)  [unwired: 1 in, 5 out]
        n566 = case shown="真" w960 {
          frame False {
          }
          frame True {
            n567 = local write "加热控制参数"(T3 {"风机开启温度(℃)"=30.0, "风机关闭温度(℃)"=20.0, "加热开启温度(℃)"=10.0, "加热关闭温度(℃)"=15.0, "风机开启温差(℃)"=5.0, "风机关闭温差(℃)"=3.0, "加热关闭温差(℃)"=10.0} ("加热控制参数")) -> ()
            n568 = local write "充电控制参数"(T4 {"最大允许单体电压(V)"=4.15, "最大允许总电压(V)"=382.0, "最小允许单体电压(V)"=2.75, "最大允许充电电流(A)"=50.0, "最小允许充电电流(A)"=3.0, "最大允许充电温度(℃)"=55.0, "最小允许充电温度(℃)"=-15.0, "电流步长"=5.0} ("充电控制参数")) -> ()
            n569 = local write "一级故障"(dbl[][] [[389.0, 391.0, 395.0], [276.0, 253.0, 230.0], [50.0, 55.0, 60.0], [-20.0, -30.0, -40.0], [0.5, 1.0, 1.5], [0.5, 1.0, 1.5], [25.0, 30.0, 35.0], [25.0, 30.0, 35.0], [4.23, 4.25, 4.3], [3.0, 2.75, 2.5], [110.0, 132.0, 165.0], [250.0, 270.0, 300.0], [101.0, 101.0, 101.0], [30.0, 20.0, 10.0], [3.0, 5.0, 10.0], [50.0, 55.0, 60.0], [90.0, 80.0, 70.0]] ("一级故障")) -> ()
            n570 = local write "电池信息"(string[][] [["电池串联", "92"], ["电池并联", "2"], ["电池包额定容量", "67"], ["电池包额定能量", "0"], ["电池包额定总电压", "340"], ["实际容量", "67"], ["电池厂家", "普莱德"], ["电池类型", "磷酸铁锂"], ["电池生产日期", "2013-12-11 11:34:30"], ["电池包组号", "0"], ["累计充电总安时", "0"], ["累计放电总安时", "0"], ["电池放空次数", "0"], ["电池充满次数", "0"], ["电池充电次数", "0"]] ("电池信息")) -> ()
          }
        }
      }
      event "全部清零(主板)": Value Change {
        n571 = event-data() -> ("NewVal"=w965:bool)  [unwired: 1 in, 5 out]
        n572 = case shown="真" w965 {
          frame False {
          }
          frame True {
            n573 = local write "加热控制参数"(T3 {"风机开启温度(℃)"=0.0, "风机关闭温度(℃)"=0.0, "加热开启温度(℃)"=0.0, "加热关闭温度(℃)"=0.0, "风机开启温差(℃)"=0.0, "风机关闭温差(℃)"=0.0, "加热关闭温差(℃)"=0.0} ("加热控制参数")) -> ()
            n574 = control-ref of="主板信息"() -> (w973:refnum<vi>)
            n575 = local write "充电控制参数"(T4 {"最大允许单体电压(V)"=0.0, "最大允许总电压(V)"=0.0, "最小允许单体电压(V)"=0.0, "最大允许充电电流(A)"=0.0, "最小允许充电电流(A)"=0.0, "最大允许充电温度(℃)"=0.0, "最小允许充电温度(℃)"=0.0, "电流步长"=0.0} ("充电控制参数")) -> ()
            n576 = local write "一级故障"(dbl[][] [[0.0, 0.0, 0.0], [0.0, 0.0, 0.0], [0.0, 0.0, 0.0], [0.0, 0.0, 0.0], [0.0, 0.0, 0.0], [0.0, 0.0, 0.0], [0.0, 0.0, 0.0], [0.0, 0.0, 0.0], [0.0, 0.0, 0.0], [0.0, 0.0, 0.0], [0.0, 0.0, 0.0], [0.0, 0.0, 0.0], [0.0, 0.0, 0.0], [0.0, 0.0, 0.0], [0.0, 0.0, 0.0], [0.0, 0.0, 0.0], [0.0, 0.0, 0.0]] ("一级故障")) -> ()
            n577 = control-ref of="电池信息"() -> (w969:refnum<vi>)
            n578 = call "表格数据输入-8.6.vi"("行数"=u32 0, "列数"=u32 1, "字符串数组"=string[] ["", "", "", "", "", "", "", "", "", "", "", "", "", "", ""], "表格引用"=w969) -> ()  [unwired: 8 in]
            n579 = call "表格数据输入-8.6.vi"("行数"=u32 0, "列数"=u32 1, "字符串数组"=string[] ["", "", "", "", "", "", "", "", "", "", "", "", "", "", "", "", "", "", "", "", "", "", "", "", "", "", "", "", "", "", "", "", "", "", "", "", "", "", "", "", "", "", "", "", "", "", "", "", "", "", "", "", "", "", "", "", "", "", "", "", "", "", "", "", "", "", "", "", "", "", "", "", "", "", "", "", "", "", "", "", "", "", "", "", "", "", "", "", "", "", "", "", "", "", "", "", "", "", "", "", "", "", "", "", "", "", "", "", "", "", "", "", "", "", "", "", "", "", "", "", "", "", "", "", "", "", "", "", "", "", "", "", "", "", "", "", "", "", "", "", "", "", "", "", "", "", "", "", "", "", "", "", "", "", "", "", "", "", "", "", "", "", "", "", "", "", "", "", "", "", "", "", "", "", "", "", "", "", "", "", "", "", "", "", "", "", "", "", "", "", "", "", "", "", "", "", "", "", "", "", ""], "表格引用"=w973) -> ()  [unwired: 8 in]
          }
        }
      }
      event "读主板参数": Value Change {
        n580 = event-data() -> ("NewVal"=w978:bool)  [unwired: 1 in, 5 out]
        n581 = case shown="真" w978 {
          tunnel: w977 -> [_ w980]
          frame False {
          }
          frame True {
            n582 = call <vilib>:"Application Directory.vi"() -> ("Application Directory"=w983:path)
            n583 = call "文件对话框3"("start path"=w983, "prompt"="选择要读取的文件", "error in"=w980) -> ("selected path"=w981:path, "cancelled"=w982:bool, "error out"=w979:errorcluster)  [unwired: 9 in, 1 out]
            n584 = case shown="假" w982 {
              tunnel: w981 -> [w990 _]
              tunnel: w979 -> [_ _]
              frame False {
                n585 = Strip Path(path=w990) -> (name=w989:string)  [unwired: 1 out]
                n586 = Match Pattern(string=w989, regular expression="M" ("正则表达式")) -> (offset past match=w987:i32)  [unwired: 1 in, 3 out]
                n587 = Equal?(x=w987, y=-1) -> (x = y?=w985:bool)
                n588 = case shown="假" w985 {
                  tunnel: w990 -> [w991 _]
                  frame False {
                    # "一级故障"
                    # "电池信息1"
                    n589 = stacked-sequence {
                      seq-local: [w1013 _ _ _] -> [_ _ _ w1133]
                      seq-local: [w998 _ _ _] -> [_ w1028 _ _]
                      seq-local: [w1001 _ _ _] -> [_ w1033 w1100 w1155]
                      seq-local: [string[] ["电池额定容量", "电池实际容量", "SOC", "SOH", "产品编号", "车架(牌)号", "配置文件版本"] _ _ _] -> [_ _ _ w1139]
                      tunnel: w991 -> [w1023 _ _ _]
                      frame #0 {
                        n590 = call-poly <vilib>:"Read From Spreadsheet File.vi"("file path (dialog if empty)"=w1023) -> ("all rows"=w1001:string[][])  [unwired: 6 in, 4 out]
                        n591 = Index Array(array=w1001, index (col)=3 ("禁用的索引 (列)")) -> (element=w1021:string[])  [unwired: 1 in]
                        n592 = Index Array(array=w1021) -> (element #1=w1020:string, element #2=w1019:string, element #3=w1018:string, element #4=w1017:string, element #5=w1015:string, element #6=w1014:string, element #7=w1016:string, element #9=w1012:string, element #10=w1011:string, element #11=w1010:string, element #12=w996:string, element #13=w995:string, element #14=w994:string, element #15=w992:string, element #16=w993:string, element #17=w1009:string, element #18=w1008:string, element #19=w1007:string, element #20=w1006:string, element #21=w1005:string, element #22=w1004:string, element #23=w1003:string, element #24=w1002:string, element #25=w997:string)  [unwired: 25 in, 1 out]
                        n593 = Build Array(w1020, w1019, w1018, w1017, w1016, w1015, w1014) -> (w1013:string[])
                        n594 = Build Array(w1012, w1011, w1010, w996, w994, w995, w993, w992, w1009, w1008, w1007, w1006, w1005, w1004, w1003, w1002, w997) -> (w999:string[])
                        n595 = for {
                          tunnel: w999 -> [w1025] mode=indexing
                          tunnel: [w1024] -> w998 mode=indexing
                          n596 = Fract/Exp String To Number(string=w1025) -> (number=w1024:dbl)  [unwired: 3 in, 1 out]
                        }
                      }
                      frame #1 {
                        n597 = Index Array(array=w1033, index (col)=7 ("禁用的索引 (列)")) -> (element=w1035:string[])  [unwired: 1 in]
                        n598 = Index Array(array=w1033, index (col)=5 ("禁用的索引 (列)")) -> (element=w1070:string[])  [unwired: 1 in]
                        n599 = Index Array(array=w1035) -> (element #1=w1036:string, element #2=w1037:string, element #3=w1038:string, element #4=w1039:string, element #5=w1041:string, element #6=w1040:string, element #7=w1043:string, element #8=w1042:string, element #9=w1044:string, element #10=w1045:string, element #11=w1046:string, element #12=w1047:string, element #13=w1048:string, element #14=w1049:string, element #15=w1050:string, element #16=w1051:string, element #17=w1052:string)  [unwired: 17 in]
                        n600 = Index Array(array=w1070) -> (element #1=w1069:string, element #2=w1068:string, element #3=w1067:string, element #4=w1066:string, element #5=w1064:string, element #6=w1065:string, element #7=w1062:string, element #8=w1063:string, element #9=w1061:string, element #10=w1060:string, element #11=w1059:string, element #12=w1058:string, element #13=w1057:string, element #14=w1056:string, element #15=w1055:string, element #16=w1054:string, element #17=w1053:string)  [unwired: 17 in]
                        n601 = Build Array(w1036, w1037, w1038, w1039, w1040, w1041, w1042, w1043, w1044, w1045, w1046, w1047, w1048, w1049, w1050, w1051, w1052) -> (w1031:string[])
                        n602 = Build Array(w1069, w1068, w1067, w1066, w1065, w1064, w1063, w1062, w1061, w1060, w1059, w1058, w1057, w1056, w1055, w1054, w1053) -> (w1032:string[])
                        n603 = for {
                          tunnel: w1031 -> [w1073] mode=indexing
                          tunnel: [w1072] -> w1026 mode=indexing
                          n604 = Fract/Exp String To Number(string=w1073) -> (number=w1072:dbl)  [unwired: 3 in, 1 out]
                        }
                        n605 = for {
                          tunnel: w1032 -> [w1075] mode=indexing
                          tunnel: [w1074] -> w1027 mode=indexing
                          n606 = Fract/Exp String To Number(string=w1075) -> (number=w1074:dbl)  [unwired: 3 in, 1 out]
                        }
                        n607 = Build Array(w1028, w1027, w1026) -> (w1030:dbl[][])
                        n608 = Transpose 2D Array(2D array=w1030) -> (transposed array=w1029:dbl[][])
                        n609 = local write "一级故障"(w1029) -> ()
                      }
                      frame #2 {
                        n610 = Index Array(array=w1100, index (col)=11 ("禁用的索引 (列)")) -> (element=w1099:string[])  [unwired: 1 in]
                        n611 = Index Array(array=w1100, index (col)=9 ("禁用的索引 (列)")) -> (element=w1109:string[])  [unwired: 1 in]
                        n612 = Delete From Array(array=w1099, length=6 ("长度"), index=0 ("索引")) -> (deleted portion=w1096:string[], array with subset deleted=w1095:string[])
                        n613 = for {
                          tunnel: w1109 -> [w1112] mode=indexing
                          tunnel: [w1111] -> w1108 mode=indexing
                          n614 = Fract/Exp String To Number(string=w1112) -> (number=w1111:dbl)  [unwired: 3 in, 1 out]
                        }
                        n615 = Index Array(array=w1095) -> (element #1=w1094:string, element #2=w1093:string, element #3=w1084:string, element #4=w1083:string, element #5=w1092:string, element #6=w1091:string, element #7=w1090:string, element #8=w1081:string, element #9=w1082:string, element #10=w1080:string, element #11=w1089:string)  [unwired: 11 in]
                        n616 = Index Array(array=w1096) -> (element #1=w1086:string, element #2=w1088:string, element #3=w1087:string, element #4=w1085:string)  [unwired: 4 in]
                        n617 = Delete From Array(array=w1108, length=7 ("长度"), index=0 ("索引")) -> (deleted portion=w1103:dbl[], array with subset deleted=w1102:dbl[])
                        n618 = Array To Cluster(array=w1102) -> (cluster=w1105:T12)
                        n619 = Array To Cluster(array=w1103) -> (cluster=w1104:T10)
                        n620 = Build Array(w1094, w1093, w1092, w1091, w1090, w1089, w1088, w1087, w1086, w1085, w1084, w1083, w1082, w1081, w1080) -> (w1077:string[])
                        n621 = local write "加热控制参数"(w1104) -> ()
                        n622 = local write "充电控制参数"(w1105) -> ()
                        n623 = Build Array(string[] ["电池串联", "电池并联", "电池包额定容量", "电池包额定能量", "电池包额定总电压", "实际容量", "电池厂家", "电池类型", "电池生产日期", "电池包组号", "累计充电总安时", "累计放电总安时", "电池放空次数", "电池充满次数", "电池充电次数"], w1077) -> (w1079:string[][])
                        n624 = Transpose 2D Array(2D array=w1079) -> (transposed array=w1076:string[][])
                        n625 = local write "电池信息"(w1076) -> ()
                      }
                      frame #3 {
                        w1140 = 20
                        w1150 = 20 ("长度")
                        n626 = Index Array(array=w1155, index (col)=1 ("禁用的索引 (列)")) -> (element=w1122:string[])  [unwired: 1 in]
                        n627 = Index Array(array=w1155, index (col)=0 ("禁用的索引 (列)")) -> (element=w1118:string[])  [unwired: 1 in]
                        n628 = Index Array(array=w1122, index=0 ("索引")) -> (element=w1154:string)
                        n629 = Search 1D Array(1D array=w1118, element="主板电压起始值" ("元素")) -> (index of element=w1148:i32)  [unwired: 1 in]
                        n630 = Search 1D Array(1D array=w1118, element="主板电池节数" ("元素")) -> (index of element=w1152:i32)  [unwired: 1 in]
                        n631 = Search 1D Array(1D array=w1118, element="主板温度个数" ("元素")) -> (index of element=w1147:i32)  [unwired: 1 in]
                        n632 = Search 1D Array(1D array=w1118, element="主板温度起始值" ("元素")) -> (index of element=w1144:i32)  [unwired: 1 in]
                        n633 = Search 1D Array(1D array=w1118, element="第1通道电压个数" ("元素")) -> (index of element=w1151:i32)  [unwired: 1 in]
                        n634 = Search 1D Array(1D array=w1118, element="第一个保险通道" ("元素")) -> (index of element=w1142:i32)  [unwired: 1 in]
                        n635 = Decimal String To Number(string=w1154) -> (number=w1119:i32)  [unwired: 2 in, 1 out]
                        n636 = Increment(x=w1119) -> (x+1=w1143:i32)
                        n637 = Array Subset(array=w1122, index=w1151, length=w1150) -> (w1127:string[])
                        n638 = Array Subset(array=w1118, index=w1152, length=w1143) -> (w1123:string[])
                        n639 = Array Subset(array=w1118, index=w1151, length=w1150) -> (w1134:string[])
                        n640 = Array Subset(array=w1122, index=w1148, length=w1143) -> (w1131:string[])
                        n641 = Array Subset(array=w1118, index=w1148, length=w1143) -> (w1138:string[])
                        n642 = Array Subset(array=w1122, index=w1147, length=w1143) -> (w1130:string[])
                        n643 = Array Subset(array=w1122, index=w1144, length=w1143) -> (w1129:string[])
                        n644 = Array Subset(array=w1118, index=w1147, length=w1143) -> (w1137:string[])
                        n645 = Array Subset(array=w1118, index=w1144, length=w1143) -> (w1136:string[])
                        n646 = Array Subset(array=w1122, index=w1142, length=w1140) -> (w1128:string[])
                        n647 = Array Subset(array=w1118, index=w1142, length=w1140) -> (w1135:string[])
                        n648 = Array Subset(array=w1122, index=w1152, length=w1143) -> (w1132:string[])
                        n649 = local write "从板个数"(w1119) -> ()
                        n650 = Insert Into Array(array=w1133, new element #1=w1132, new element #2=w1131, new element #3=w1130, new element #4=w1129, new element #5=w1128, new element #6=w1127) -> (w1125:string[])  [unwired: 1 in]
                        n651 = Multiply(x=w1119, y=2.0) -> (x*y=w1116:dbl)
                        n652 = Array Subset(array=w1122, index=1 ("索引"), length=w1116) -> (w1114:string[])
                        n653 = Insert Into Array(array=w1139, new element #1=w1123, new element #2=w1138, new element #3=w1137, new element #4=w1136, new element #5=w1135, new element #6=w1134) -> (w1126:string[])  [unwired: 1 in]
                        n654 = Array Subset(array=w1118, index=1 ("索引"), length=w1116) -> (w1115:string[])
                        n655 = Build Array(w1126, w1125) -> ()  [unwired: 1 out]
                        n656 = Build Array(w1115, w1114) -> (w1113:string[][])
                        n657 = Transpose 2D Array(2D array=w1113) -> (transposed array=w1124:string[][])
                        n658 = local write "主板信息"(w1124) -> ()
                      }
                    }
                  }
                  frame True {
                    n659 = One Button Dialog(message="选择文件类型错误" ("消息"), button name ("OK")="确定" ("按钮名称（“确定”）")) -> ()  [unwired: 1 out]
                  }
                }
              }
              frame True {
              }
            }
          }
        }
      }
      event "读从板参数": Value Change {
        n660 = event-data() -> ("NewVal"=w1164:bool)  [unwired: 1 in, 5 out]
        n661 = case shown="真" w1164 {
          tunnel: w1163 -> [_ w1167]
          tunnel: w1162 -> [_ w1165]
          frame False {
          }
          frame True {
            n662 = call <vilib>:"Application Directory.vi"() -> ("Application Directory"=w1170:path)
            n663 = call "文件对话框4"("start path"=w1170, "prompt"="选择要读取的文件", "error in"=w1167) -> ("selected path"=w1168:path, "cancelled"=w1169:bool, "error out"=w1166:errorcluster)  [unwired: 9 in, 1 out]
            n664 = case shown="假" w1169 {
              tunnel: w1168 -> [w1173 _]
              tunnel: w1166 -> [_ _]
              tunnel: w1165 -> [w1172 _]
              frame False {
                n665 = Strip Path(path=w1173) -> (name=w1178:string)  [unwired: 1 out]
                n666 = Match Pattern(string=w1178, regular expression="S" ("正则表达式")) -> (offset past match=w1176:i32)  [unwired: 1 in, 3 out]
                n667 = Equal?(x=w1176, y=-1) -> (x = y?=w1174:bool)
                n668 = case shown="假" w1174 {
                  tunnel: w1173 -> [w1180 _]
                  tunnel: w1172 -> [w1179 _]
                  frame False {
                    n669 = stacked-sequence {
                      seq-local: [w1198 _ _ _ _] -> [_ w1204 w1237 _ _]
                      seq-local: [w1183 _ _ _ _] -> [_ _ _ _ w1283]
                      seq-local: [w1181 _ _ _ _] -> [_ _ _ _ w1282]
                      seq-local: [_ _ w1222 _ _] -> [_ _ _ _ w1284]
                      seq-local: [_ _ w1221 _ _] -> [_ _ _ w1249 w1285]
                      seq-local: [_ w1203 _ _ _] -> [_ _ _ _ w1277]
                      tunnel: w1180 -> [w1199 _ _ _ _]
                      tunnel: w1179 -> [_ _ w1215 _ _]
                      frame #0 {
                        n670 = call-poly <vilib>:"Read From Spreadsheet File.vi"("file path (dialog if empty)"=w1199) -> ("all rows"=w1198:string[][])  [unwired: 6 in, 4 out]
                        n671 = Index Array(array=w1198, index (col)=3 ("禁用的索引 (列)")) -> (element=w1197:string[])  [unwired: 1 in]
                        n672 = for {
                          tunnel: w1197 -> [w1202] mode=indexing
                          tunnel: [w1201] -> w1196 mode=indexing
                          n673 = Fract/Exp String To Number(string=w1202) -> (number=w1201:dbl)  [unwired: 3 in, 1 out]
                        }
                        n674 = Delete From Array(array=w1196, length=7 ("长度"), index=0 ("索引")) -> (deleted portion=w1184:dbl[], array with subset deleted=w1193:dbl[])
                        n675 = Delete From Array(array=w1193, length=7 ("索引"), index=0 ("索引")) -> (deleted portion=w1187:dbl[], array with subset deleted=w1188:dbl[])
                        n676 = Array To Cluster(array=w1184) -> (cluster=w1183:T10)
                        n677 = Delete From Array(array=w1188, length=7 ("索引"), index=0 ("索引")) -> (deleted portion=w1186:dbl[], array with subset deleted=w1185:dbl[])
                        n678 = local write "加热控制参数 2"(w1183) -> ()
                        n679 = Build Array(w1187, w1186, w1185) -> (w1182:dbl[][])
                        n680 = Transpose 2D Array(2D array=w1182) -> (transposed array=w1181:dbl[][])
                        n681 = local write "一级故障 2"(w1181) -> ()
                      }
                      frame #1 {
                        n682 = disable-structure shown="禁用" {
                          disable-tunnel: w1204 -> [w1208 _]
                          disable-tunnel: [w1207 _] -> w1203
                          frame Disabled {
                            n683 = Index Array(array=w1208, index (col)=7 ("禁用的索引 (列)")) -> (element=w1207:string[])  [unwired: 1 in]
                            n684 = for {
                              tunnel: w1207 -> [w1211] mode=indexing
                              tunnel: [w1210] -> w1206 mode=indexing
                              n685 = Fract/Exp String To Number(string=w1211) -> (number=w1210:dbl)  [unwired: 3 in, 1 out]
                            }
                            n686 = Array To Cluster(array=w1206) -> (cluster=w1205:T13)
                            n687 = local write "均衡参数"(w1205) -> ()
                          }
                          frame Enabled {
                          }
                        }
                      }
                      frame #2 {
                        # "第一个保险位置"
                        # "温度个数"
                        # "通道电压节数"
                        # "电压节数"
                        n688 = Index Array(array=w1237, index (col)=1 ("禁用的索引 (列)")) -> (element=w1219:string[])  [unwired: 1 in]
                        n689 = Index Array(array=w1219, index=0 ("索引")) -> (element=w1236:string)
                        n690 = Decimal String To Number(string=w1236) -> (number=w1222:i32)  [unwired: 2 in, 1 out]
                        n691 = Array Subset(array=w1219, index=3 ("禁用的索引 (列)"), length=20 ("禁用的索引 (列)")) -> (w1223:string[])
                        n692 = Array Subset(array=w1219, index=23 ("禁用的索引 (列)"), length=2 ("禁用的索引 (列)")) -> (w1225:string[])
                        n693 = Array Subset(array=w1219, index=1 ("禁用的索引 (列)"), length=2 ("禁用的索引 (列)")) -> (w1226:string[])
                        n694 = Array Subset(array=w1219, index=25 ("禁用的索引 (列)"), length=20 ("禁用的索引 (列)")) -> (w1224:string[])
                        n695 = local write "从板板号"(w1222) -> ()
                        n696 = Array Subset(array=w1219, index=1 ("索引"), length=27 ("长度")) -> (w1216:string[])
                        n697 = Insert Into Array(array=w1226, new element #1=w1225, new element #2=w1224, new element #3=w1223) -> ()  [unwired: 1 in, 1 out]
                        n698 = Array Subset(array=w1215, index=1 ("索引"), length=27 ("长度")) -> (w1214:string[])
                        n699 = Build Array(w1214, w1216) -> (w1235:string[][])
                        n700 = Transpose 2D Array(2D array=w1235) -> (transposed array=w1221:string[][])
                        n701 = local write "保险位置"(bool[][] [[FALSE, FALSE, FALSE, FALSE, FALSE, FALSE, FALSE, FALSE, FALSE, FALSE, FALSE, FALSE], [FALSE, FALSE, FALSE, FALSE, FALSE, FALSE, FALSE, FALSE, FALSE, FALSE, FALSE, FALSE], [FALSE, FALSE, FALSE, FALSE, FALSE, FALSE, FALSE, FALSE, FALSE, FALSE, FALSE, FALSE], [FALSE, FALSE, FALSE, FALSE, FALSE, FALSE, FALSE, FALSE, FALSE, FALSE, FALSE, FALSE], [FALSE, FALSE, FALSE, FALSE, FALSE, FALSE, FALSE, FALSE, FALSE, FALSE, FALSE, FALSE], [FALSE, FALSE, FALSE, FALSE, FALSE, FALSE, FALSE, FALSE, FALSE, FALSE, FALSE, FALSE], [FALSE, FALSE, FALSE, FALSE, FALSE, FALSE, FALSE, FALSE, FALSE, FALSE, FALSE, FALSE], [FALSE, FALSE, FALSE, FALSE, FALSE, FALSE, FALSE, FALSE, FALSE, FALSE, FALSE, FALSE], [FALSE, FALSE, FALSE, FALSE, FALSE, FALSE, FALSE, FALSE, FALSE, FALSE, FALSE, FALSE], [FALSE, FALSE, FALSE, FALSE, FALSE, FALSE, FALSE, FALSE, FALSE, FALSE, FALSE, FALSE]]) -> ()
                        n702 = local write "从板信息电压温度通道配置"(w1221) -> ()
                      }
                      frame #3 {
                        n703 = Index Array(array=w1249, index (col)=1 ("禁用的索引 (列)")) -> (element=w1241:string[])  [unwired: 1 in]
                        n704 = Array Subset(array=w1241, index=4 ("索引"), length=20 ("长度")) -> (w1252:string[])
                        n705 = Array Subset(array=w1241, index=24 ("索引"), length=20 ("长度")) -> (w1242:string[])
                        n706 = for {
                          tunnel: w1252 -> [w1276] mode=indexing
                          shift-right: [w1273] -> w1245
                          shift-left: i32[] [] -> [w1272]
                          n707 = Fract/Exp String To Number(string=w1276, default (0 dbl)=u8 0) -> (number=w1271:u8)  [unwired: 2 in, 1 out]
                          n708 = Equal To 0?(x=w1271) -> (x = 0?=w1274:bool)
                          n709 = Insert Into Array(array=w1272, new element=w1271) -> (w1270:i32[])  [unwired: 1 in]
                          n710 = Select(t=w1272, s=w1274, f=w1270) -> (s? t:f=w1273:i32[])
                        }
                        n711 = for {
                          tunnel: w1242 -> [w1257] mode=indexing
                          tunnel: [w1256] -> w1240 mode=indexing
                          n712 = Fract/Exp String To Number(string=w1257, default (0 dbl)=u8 0) -> (number=w1256:u8)  [unwired: 2 in, 1 out]
                        }
                        n713 = local write "5个通道电压个数(最小5个)"(w1240) -> ()
                        n714 = Array Size(array=w1245) -> (size(s)=w1248:i32)
                        n715 = Quotient & Remainder(x=w1248, y=2) -> (floor(x/y)=w1246:i32)  [unwired: 1 out]
                        n716 = for {
                          N: w1246 -> [_]
                          tunnel: w1245 -> [w1261]
                          i -> [w1260]
                          n717 = Multiply(x=w1260, y=2) -> (x*y=w1268:i32)
                          n718 = Increment(x=w1268) -> (x+1=w1267:i32)
                          n719 = Index Array(array=w1261, index #1=w1268, index #2=w1267) -> (element #1=w1266:i32, element #2=w1265:i32)
                          n720 = local read "保险位置"() -> (w1258:T6)
                          n721 = Decrement(x=w1266) -> (x-1=w1263:i32)
                          n722 = Decrement(x=w1265) -> (x-1=w1262:i32)
                          n723 = Replace Array Subset(array=w1258, new element=TRUE, index (row)=w1263, index (col)=w1262) -> (w1259:T6)
                          n724 = local write "保险位置"(w1259) -> ()
                        }
                      }
                      frame #4 {
                        n725 = Transpose 2D Array(2D array=w1282) -> (transposed array=w1291:dbl[][])
                        n726 = Array Subset(array=w1285, index (row)=0 ("索引"), index (col)=0 ("索引"), length (col)=2 ("索引")) -> (w1302:string[][])  [unwired: 1 in]
                        n727 = for {
                          tunnel: w1291 -> [w1320] mode=indexing
                          shift-right: [w1319] -> w1299
                          shift-left: string[] [] -> [w1317]
                          n728 = for {
                            N: 7 -> [_]
                            tunnel: w1320 -> [w1323] mode=indexing
                            tunnel: [w1321] -> w1318 mode=indexing
                            n729 = Format Into String(format string="%#f" ("格式字符串"), w1323) -> (resulting string=w1321:string)  [unwired: 2 in, 1 out]
                          }
                          n730 = Insert Into Array(array=w1317, new element=w1318) -> (w1319:string[])  [unwired: 1 in]
                        }
                        n731 = Cluster To Array(cluster=w1283) -> (array=w1304:dbl[])
                        n732 = Index Array(array=w1302, index (col) #1=0 ("禁用的索引 (列)"), index (col) #2=1 ("索引 (列)")) -> (element #1=w1290:string[], element #2=w1292:string[])  [unwired: 2 in]
                        n733 = for {
                          tunnel: w1304 -> [w1326] mode=indexing
                          tunnel: [w1324] -> w1300 mode=indexing
                          n734 = Format Into String(format string="%#f" ("格式字符串"), w1326) -> (resulting string=w1324:string)  [unwired: 2 in, 1 out]
                        }
                        n735 = Insert Into Array(array=w1290, index=0 ("索引"), new element="从板板号" ("新元素/子数组")) -> (w1287:string[])
                        n736 = Number To Decimal String(number=w1284) -> (decimal integer string=w1294:string)  [unwired: 1 in]
                        n737 = Insert Into Array(array=w1287, new element=string[] ["从板板号", "电压个数", "电压起始值", "温度个数", "温度起始值", "第一个保险通道", "第一个保险位置", "第二个保险通道", "第二个保险位置", "第三个保险通道", "第三个保险位置", "第四个保险通道", "第四个保险位置", "第五个保险通道", "第五个保险位置", "第六个保险通道", "第六个保险位置", "第七个保险通道", "第七个保险位置", "第八个保险通道", "第八个保险位置", "第九个保险通道", "第九个保险位置", "第十个保险通道", "第十个保险位置", "第1通道电压个数", "第2通道电压个数", "第3通道电压个数", "第4通道电压个数", "第5通道电压个数", "第6通道电压个数", "第7通道电压个数", "第8通道电压个数", "第9通道电压个数", "第10通道电压个数", "第11通道电压个数", "第12通道电压个数", "第13通道电压个数", "第14通道电压个数", "第15通道电压个数", "第16通道电压个数", "第17通道电压个数", "第18通道电压个数", "第19通道电压个数", "第20通道电压个数", "风机开启温度", "风机关闭温度", "加热开启温度", "加热关闭温度", "风机开启温差", "风机关闭温差", "加热关闭温差", "电压过高一级", "电压过低一级", "温度过高一级", "温度过低一级", "电压不均衡一级", "温度不均衡一级", "SOC过低一级", "电压过高二级", "电压过低二级", "温度过高二级", "温度过低二级", "电压不均衡二级", "温度不均衡二级", "SOC过低二级", "电压过高三级", "电压过低三级", "温度过高三级", "温度过低三级", "电压不均衡三级", "温度不均衡三级", "SOC过低三级", "均衡计算-电压高阀值1级", "均衡计算-电压高阀值2级", "均衡计算-电压低阀值1级", "均衡计算-电压低阀值2级", "均衡计算-最低电压阀值", "均衡停止-最低电压阀值", "均衡计算-电压极差阀值", "充电结束电压(90%)", "充电结束电压(91%)", "充电结束电压(92%)", "充电结束电压(93%)", "充电结束电压(94%)", "充电结束电压(95%)", "充电结束电压(96%)", "充电结束电压(97%)", "充电结束电压(98%)", "充电结束电压(99%)", "充电结束电压(100%)"] ("从板表头")) -> (w1281:string[])  [unwired: 1 in]
                        n738 = local read "输出数组"() -> (w1280:string[][])
                        n739 = Insert Into Array(array=w1292, new element #1=w1300, new element #2=w1299, new element #3=w1277) -> (w1298:string[])  [unwired: 1 in]
                        n740 = Decrement(x=w1284) -> (x-1=w1279:i32)
                        n741 = local write "从板表头"(w1281) -> ()
                        n742 = Insert Into Array(array=w1298, index=0 ("索引"), new element=w1294) -> (w1296:string[])
                        n743 = Replace Array Subset(array=w1280, new element=w1296, index (col)=w1279) -> (w1295:string[][])  [unwired: 1 in]
                        n744 = stacked-sequence {
                          tunnel: w1295 -> [w1308]
                          tunnel: w1294 -> [w1313]
                          frame #0 {
                            n745 = control-ref of="结果"() -> (w1315:refnum<vi>)
                            n746 = Concatenate Strings("从板", w1313, "记录完成") -> (w1311:string)
                            n747 = local write "输出数组"(w1308) -> ()
                            n748 = Build Array(w1311) -> (w1309:string[])
                            n749 = call "表格编辑.vi"("新元素/子数组"=w1309, "活动单元格:单元格背景色"=u32 6618880, "MCListbox引用句柄"=w1315) -> ()  [unwired: 9 in]
                          }
                        }
                        n750 = property on="查看" class="Bool (严格)"("Visible"=TRUE ("可见")) -> ()  [unwired: 2 in, 2 out]
                      }
                    }
                  }
                  frame True {
                    n751 = One Button Dialog(message="选择文件类型错误" ("消息"), button name ("OK")="确定" ("按钮名称（“确定”）")) -> ()  [unwired: 1 out]
                  }
                }
              }
              frame True {
              }
            }
          }
        }
      }
      event "从板信息电压温度通道配置": Value Change {
        w1329 = bool[][] [[FALSE, FALSE, FALSE, FALSE, FALSE, FALSE, FALSE, FALSE, FALSE, FALSE, FALSE, FALSE], [FALSE, FALSE, FALSE, FALSE, FALSE, FALSE, FALSE, FALSE, FALSE, FALSE, FALSE, FALSE], [FALSE, FALSE, FALSE, FALSE, FALSE, FALSE, FALSE, FALSE, FALSE, FALSE, FALSE, FALSE], [FALSE, FALSE, FALSE, FALSE, FALSE, FALSE, FALSE, FALSE, FALSE, FALSE, FALSE, FALSE], [FALSE, FALSE, FALSE, FALSE, FALSE, FALSE, FALSE, FALSE, FALSE, FALSE, FALSE, FALSE], [FALSE, FALSE, FALSE, FALSE, FALSE, FALSE, FALSE, FALSE, FALSE, FALSE, FALSE, FALSE], [FALSE, FALSE, FALSE, FALSE, FALSE, FALSE, FALSE, FALSE, FALSE, FALSE, FALSE, FALSE], [FALSE, FALSE, FALSE, FALSE, FALSE, FALSE, FALSE, FALSE, FALSE, FALSE, FALSE, FALSE], [FALSE, FALSE, FALSE, FALSE, FALSE, FALSE, FALSE, FALSE, FALSE, FALSE, FALSE, FALSE], [FALSE, FALSE, FALSE, FALSE, FALSE, FALSE, FALSE, FALSE, FALSE, FALSE, FALSE, FALSE]]
        n752 = event-data() -> ("NewVal"=w1330:string[][])  [unwired: 1 in, 5 out]
        n753 = Index Array(array=w1330, index (col)=1 ("禁用的索引 (列)")) -> (element=w1332:string[])  [unwired: 1 in]
        n754 = Array Subset(array=w1332, index=4 ("索引"), length=20 ("长度")) -> (w1342:string[])
        n755 = Array Subset(array=w1332, index=24 ("索引"), length=20 ("长度")) -> (w1333:string[])
        n756 = for {
          tunnel: w1342 -> [w1366] mode=indexing
          shift-right: [w1363] -> w1336
          shift-left: i32[] [] -> [w1362]
          n757 = Fract/Exp String To Number(string=w1366, default (0 dbl)=u8 0) -> (number=w1361:u8)  [unwired: 2 in, 1 out]
          n758 = Equal To 0?(x=w1361) -> (x = 0?=w1364:bool)
          n759 = Insert Into Array(array=w1362, new element=w1361) -> (w1360:i32[])  [unwired: 1 in]
          n760 = Select(t=w1362, s=w1364, f=w1360) -> (s? t:f=w1363:i32[])
        }
        n761 = for {
          tunnel: w1333 -> [w1347] mode=indexing
          tunnel: [w1346] -> w1331 mode=indexing
          n762 = Fract/Exp String To Number(string=w1347, default (0 dbl)=u8 0) -> (number=w1346:u8)  [unwired: 2 in, 1 out]
        }
        n763 = local write "5个通道电压个数(最小5个)"(w1331) -> ()
        n764 = Array Size(array=w1336) -> (size(s)=w1339:i32)
        n765 = Quotient & Remainder(x=w1339, y=2) -> (floor(x/y)=w1337:i32)  [unwired: 1 out]
        n766 = for {
          N: w1337 -> [_]
          tunnel: w1336 -> [w1351]
          tunnel: w1329 -> [_]
          i -> [w1350]
          n767 = Multiply(x=w1350, y=2) -> (x*y=w1358:i32)
          n768 = Increment(x=w1358) -> (x+1=w1357:i32)
          n769 = Index Array(array=w1351, index #1=w1358, index #2=w1357) -> (element #1=w1356:i32, element #2=w1355:i32)
          n770 = local read "保险位置"() -> (w1348:T6)
          n771 = Decrement(x=w1356) -> (x-1=w1353:i32)
          n772 = Decrement(x=w1355) -> (x-1=w1352:i32)
          n773 = Replace Array Subset(array=w1348, new element=TRUE, index (row)=w1353, index (col)=w1352) -> (w1349:T6)
          n774 = local write "保险位置"(w1349) -> ()
        }
        n775 = local write "保险位置"(w1329) -> ()
      }
      event "从板板号": Value Change {
        n776 = event-data() -> ("NewVal"=w1369:dbl)  [unwired: 1 in, 5 out]
        n777 = Decrement(x=w1369) -> (x-1=w1373:dbl)
        n778 = local read "输出数组"() -> (w1374:string[][])
        n779 = Index Array(array=w1374, index (col)=w1373) -> (element=w1372:string[])  [unwired: 1 in]
        n780 = Index Array(array=w1372, index=0 ("索引")) -> (element=w1368:string)
        n781 = Decimal String To Number(string=w1368) -> (number=w1367:i32)  [unwired: 2 in, 1 out]
        n782 = Equal?(x=w1367, y=w1369) -> (x = y?=w1370:bool)
        n783 = case shown="真" w1370 {
          tunnel: w1372 -> [_ w1375]
          frame False {
          }
          frame True {
            n784 = stacked-sequence {
              seq-local: [_ w1383 _] -> [_ _ w1421]
              tunnel: w1375 -> [_ w1385 _]
              frame #0 {
                n785 = local write "从板信息电压温度通道配置"(string[][] [] ("key names")) -> ()
                n786 = local write "一级故障 2"(dbl[][] [[0.0, 0.0, 0.0, 0.0, 0.0, 0.0, 0.0, 0.0, 0.0, 0.0, 0.0, 0.0, 0.0, 0.0, 0.0, 0.0, 0.0]] ("一级故障 2")) -> ()
                n787 = local write "加热控制参数 2"(T9 {"风机开启温度"=0.0, "风机关闭温度"=0.0, "加热开启温度"=0.0, "加热关闭温度"=0.0, "风机开启温差"=0.0, "风机关闭温差"=0.0, "加热关闭温差"=0.0} ("加热控制参数 2")) -> ()
              }
              frame #1 {
                n788 = local read "从板表头"() -> (w1384:string[])
                n789 = Search 1D Array(1D array=w1384, element="风机开启温度" ("元素")) -> (index of element=w1404:i32)  [unwired: 1 in]
                n790 = Search 1D Array(1D array=w1384, element="电压过高一级" ("元素"), start index (0)=w1404) -> (index of element=w1402:i32)
                n791 = Decrement(x=w1404) -> (x-1=w1406:i32)
                n792 = Array Subset(array=string[] ["从板板号", "电压个数", "温度个数", "第一个保险通道", "第一个保险位置", "第二个保险通道", "第二个保险位置", "第三个保险通道", "第三个保险位置", "第四个保险通道", "第四个保险位置", "第五个保险通道", "第五个保险位置", "第六个保险通道", "第六个保险位置", "第七个保险通道", "第七个保险位置", "第八个保险通道", "第八个保险位置", "第九个保险通道", "第九个保险位置", "第十个保险通道", "第十个保险位置", "第1通道电压个数", "第2通道电压个数", "第3通道电压个数", "第4通道电压个数", "第5通道电压个数", "第6通道电压个数", "第7通道电压个数", "第8通道电压个数", "第9通道电压个数", "第10通道电压个数", "第11通道电压个数", "第12通道电压个数", "第13通道电压个数", "第14通道电压个数", "第15通道电压个数", "第16通道电压个数", "第17通道电压个数", "第18通道电压个数", "第19通道电压个数", "第20通道电压个数", "风机开启温度", "风机关闭温度", "加热开启温度", "加热关闭温度", "风机开启温差", "风机关闭温差", "加热关闭温差", "电压过高一级", "电压过低一级", "温度过高一级", "温度过低一级", "电压不均衡一级", "温度不均衡一级", "SOC过低一级", "电压过高二级", "电压过低二级", "温度过高二级", "温度过低二级", "电压不均衡二级", "温度不均衡二级", "SOC过低二级", "电压过高三级", "电压过低三级", "温度过高三级", "温度过低三级", "电压不均衡三级", "温度不均衡三级", "SOC过低三级", "均衡计算-电压高阀值1级", "均衡计算-电压高阀值2级", "均衡计算-电压低阀值1级", "均衡计算-电压低阀值2级", "均衡计算-最低电压阀值", "均衡停止-最低电压阀值", "均衡计算-电压极差阀值", "充电结束电压(90%)", "充电结束电压(91%)", "充电结束电压(92%)", "充电结束电压(93%)", "充电结束电压(94%)", "充电结束电压(95%)", "充电结束电压(96%)", "充电结束电压(97%)", "充电结束电压(98%)", "充电结束电压(99%)", "充电结束电压(100%)"] ("从板表头"), index=1 ("长度"), length=27 ("长度")) -> (w1379:string[])
                n793 = Array Subset(array=w1385, index=1 ("索引"), length=w1406) -> (w1408:string[])
                n794 = Array Subset(array=w1385, index=w1402, length=21 ("长度")) -> (w1387:string[])
                n795 = Array Subset(array=w1385, index=w1404, length=7 ("长度")) -> (w1400:string[])
                n796 = for {
                  tunnel: w1387 -> [w1412] mode=indexing
                  tunnel: [w1411] -> w1386 mode=indexing
                  n797 = Fract/Exp String To Number(string=w1412) -> (number=w1411:dbl)  [unwired: 3 in, 1 out]
                }
                n798 = for {
                  tunnel: w1400 -> [w1414] mode=indexing
                  tunnel: [w1413] -> w1399 mode=indexing
                  n799 = Fract/Exp String To Number(string=w1414) -> (number=w1413:dbl)  [unwired: 3 in, 1 out]
                }
                n800 = Build Array(w1379, w1408) -> (w1407:string[][])
                n801 = Delete From Array(array=w1386, length=7 ("长度"), index=0 ("索引")) -> (deleted portion=w1395:dbl[], array with subset deleted=w1394:dbl[])
                n802 = Transpose 2D Array(2D array=w1407) -> (transposed array=w1383:string[][])
                n803 = Array To Cluster(array=w1399) -> (cluster=w1398:T10)
                n804 = Delete From Array(array=w1394, length=7 ("长度"), index=0 ("索引")) -> (deleted portion=w1391:dbl[], array with subset deleted=w1390:dbl[])
                n805 = local write "从板信息电压温度通道配置"(w1383) -> ()
                n806 = local write "加热控制参数 2"(w1398) -> ()
                n807 = Build Array(w1395, w1391, w1390) -> (w1389:dbl[][])
                n808 = Transpose 2D Array(2D array=w1389) -> (transposed array=w1388:dbl[][])
                n809 = local write "一级故障 2"(w1388) -> ()
              }
              frame #2 {
                w1426 = bool[][] [[FALSE, FALSE, FALSE, FALSE, FALSE, FALSE, FALSE, FALSE, FALSE, FALSE, FALSE, FALSE], [FALSE, FALSE, FALSE, FALSE, FALSE, FALSE, FALSE, FALSE, FALSE, FALSE, FALSE, FALSE], [FALSE, FALSE, FALSE, FALSE, FALSE, FALSE, FALSE, FALSE, FALSE, FALSE, FALSE, FALSE], [FALSE, FALSE, FALSE, FALSE, FALSE, FALSE, FALSE, FALSE, FALSE, FALSE, FALSE, FALSE], [FALSE, FALSE, FALSE, FALSE, FALSE, FALSE, FALSE, FALSE, FALSE, FALSE, FALSE, FALSE], [FALSE, FALSE, FALSE, FALSE, FALSE, FALSE, FALSE, FALSE, FALSE, FALSE, FALSE, FALSE], [FALSE, FALSE, FALSE, FALSE, FALSE, FALSE, FALSE, FALSE, FALSE, FALSE, FALSE, FALSE], [FALSE, FALSE, FALSE, FALSE, FALSE, FALSE, FALSE, FALSE, FALSE, FALSE, FALSE, FALSE], [FALSE, FALSE, FALSE, FALSE, FALSE, FALSE, FALSE, FALSE, FALSE, FALSE, FALSE, FALSE], [FALSE, FALSE, FALSE, FALSE, FALSE, FALSE, FALSE, FALSE, FALSE, FALSE, FALSE, FALSE]]
                n810 = Index Array(array=w1421, index (col)=1 ("禁用的索引 (列)")) -> (element=w1420:string[])  [unwired: 1 in]
                n811 = Array Subset(array=w1420, index=4 ("索引"), length=20 ("长度")) -> (w1433:string[])
                n812 = Array Subset(array=w1420, index=22 ("索引"), length=5 ("长度")) -> (w1423:string[])
                n813 = Index Array(array=w1420, index #1=0 ("索引")) -> (element #1=w1418:string, element #2=w1417:string)  [unwired: 1 in]
                n814 = for {
                  tunnel: w1423 -> [w1438] mode=indexing
                  tunnel: [w1437] -> w1422 mode=indexing
                  n815 = Fract/Exp String To Number(string=w1438, default (0 dbl)=u8 0) -> (number=w1437:u8)  [unwired: 2 in, 1 out]
                }
                n816 = for {
                  tunnel: w1433 -> [w1457] mode=indexing
                  shift-right: [w1454] -> w1427
                  shift-left: i32[] [] -> [w1453]
                  n817 = Fract/Exp String To Number(string=w1457, default (0 dbl)=u8 0) -> (number=w1452:u8)  [unwired: 2 in, 1 out]
                  n818 = Equal To 0?(x=w1452) -> (x = 0?=w1455:bool)
                  n819 = Insert Into Array(array=w1453, new element=w1452) -> (w1451:i32[])  [unwired: 1 in]
                  n820 = Select(t=w1453, s=w1455, f=w1451) -> (s? t:f=w1454:i32[])
                }
                n821 = Fract/Exp String To Number(string=w1417) -> (number=w1415:dbl)  [unwired: 3 in, 1 out]
                n822 = Fract/Exp String To Number(string=w1418) -> (number=w1416:dbl)  [unwired: 3 in, 1 out]
                n823 = local write "温度个数"(w1415) -> ()
                n824 = local write "电压个数"(w1416) -> ()
                n825 = local write "5个通道电压个数(最小5个)"(w1422) -> ()
                n826 = Array Size(array=w1427) -> (size(s)=w1430:i32)
                n827 = Quotient & Remainder(x=w1430, y=2) -> (floor(x/y)=w1428:i32)  [unwired: 1 out]
                n828 = for {
                  N: w1428 -> [_]
                  tunnel: w1427 -> [w1442]
                  tunnel: w1426 -> [_]
                  i -> [w1441]
                  n829 = Multiply(x=w1441, y=2) -> (x*y=w1449:i32)
                  n830 = Increment(x=w1449) -> (x+1=w1448:i32)
                  n831 = Index Array(array=w1442, index #1=w1449, index #2=w1448) -> (element #1=w1447:i32, element #2=w1446:i32)
                  n832 = local read "保险位置"() -> (w1439:T6)
                  n833 = Decrement(x=w1447) -> (x-1=w1444:i32)
                  n834 = Decrement(x=w1446) -> (x-1=w1443:i32)
                  n835 = Replace Array Subset(array=w1439, new element=TRUE, index (row)=w1444, index (col)=w1443) -> (w1440:T6)
                  n836 = local write "保险位置"(w1440) -> ()
                }
                n837 = local write "保险位置"(w1426) -> ()
              }
            }
          }
        }
      }
      event "查看": Value Change {
        n838 = event-data() -> ("NewVal"=w1458:bool)  [unwired: 1 in, 5 out]
        n839 = case shown="假" w1458 {
          frame False {
            n840 = call "选择从板号"() -> ("从板号"=w1459:dbl, "确定"=w1460:bool)  [unwired: 17 in, 1 out]
            n841 = case shown="真" w1460 {
              tunnel: w1459 -> [_ w1461]
              frame False {
              }
              frame True {
                n842 = local read "从板表头"() -> (w1462:string[])
                n843 = stacked-sequence {
                  tunnel: w1461 -> [_ w1474 w1506]
                  tunnel: w1462 -> [_ w1472 _]
                  frame #0 {
                    n844 = local write "从板信息电压温度通道配置"(string[][] [] ("key names")) -> ()
                    n845 = local write "一级故障 2"(dbl[][] [[0.0, 0.0, 0.0, 0.0, 0.0, 0.0, 0.0, 0.0, 0.0, 0.0, 0.0, 0.0, 0.0, 0.0, 0.0, 0.0, 0.0]] ("一级故障 2")) -> ()
                    n846 = local write "加热控制参数 2"(T9 {"风机开启温度"=0.0, "风机关闭温度"=0.0, "加热开启温度"=0.0, "加热关闭温度"=0.0, "风机开启温差"=0.0, "风机关闭温差"=0.0, "加热关闭温差"=0.0} ("加热控制参数 2")) -> ()
                  }
                  frame #1 {
                    n847 = local read "输出数组"() -> (w1473:string[][])
                    n848 = Decrement(x=w1474) -> (x-1=w1470:dbl)
                    n849 = Index Array(array=w1473, index (col)=w1470) -> (element=w1492:string[])  [unwired: 1 in]
                    n850 = Search 1D Array(1D array=w1472, element="风机开启温度" ("元素")) -> (index of element=w1494:i32)  [unwired: 1 in]
                    n851 = Search 1D Array(1D array=w1472, element="电压过高一级" ("元素"), start index (0)=w1494) -> (index of element=w1491:i32)
                    n852 = Decrement(x=w1494) -> (x-1=w1496:i32)
                    n853 = Array Subset(array=w1492, index=1 ("索引"), length=w1496) -> (w1498:string[])
                    n854 = Array Subset(array=w1492, index=w1491, length=21 ("长度")) -> (w1476:string[])
                    n855 = Array Subset(array=w1492, index=w1494, length=7 ("长度")) -> (w1489:string[])
                    n856 = Array Subset(array=string[] ["从板板号", "电压个数", "电压起始值", "温度个数", "温度起始值", "第一个保险通道", "第一个保险位置", "第二个保险通道", "第二个保险位置", "第三个保险通道", "第三个保险位置", "第四个保险通道", "第四个保险位置", "第五个保险通道", "第五个保险位置", "第六个保险通道", "第六个保险位置", "第七个保险通道", "第七个保险位置", "第八个保险通道", "第八个保险位置", "第九个保险通道", "第九个保险位置", "第十个保险通道", "第十个保险位置", "第1通道电压个数", "第2通道电压个数", "第3通道电压个数", "第4通道电压个数", "第5通道电压个数", "第6通道电压个数", "第7通道电压个数", "第8通道电压个数", "第9通道电压个数", "第10通道电压个数", "第11通道电压个数", "第12通道电压个数", "第13通道电压个数", "第14通道电压个数", "第15通道电压个数", "第16通道电压个数", "第17通道电压个数", "第18通道电压个数", "第19通道电压个数", "第20通道电压个数", "风机开启温度", "风机关闭温度", "加热开启温度", "加热关闭温度", "风机开启温差", "风机关闭温差", "加热关闭温差", "电压过高一级", "电压过低一级", "温度过高一级", "温度过低一级", "电压不均衡一级", "温度不均衡一级", "SOC过低一级", "电压过高二级", "电压过低二级", "温度过高二级", "温度过低二级", "电压不均衡二级", "温度不均衡二级", "SOC过低二级", "电压过高三级", "电压过低三级", "温度过高三级", "温度过低三级", "电压不均衡三级", "温度不均衡三级", "SOC过低三级", "均衡计算-电压高阀值1级", "均衡计算-电压高阀值2级", "均衡计算-电压低阀值1级", "均衡计算-电压低阀值2级", "均衡计算-最低电压阀值", "均衡停止-最低电压阀值", "均衡计算-电压极差阀值", "充电结束电压(90%)", "充电结束电压(91%)", "充电结束电压(92%)", "充电结束电压(93%)", "充电结束电压(94%)", "充电结束电压(95%)", "充电结束电压(96%)", "充电结束电压(97%)", "充电结束电压(98%)", "充电结束电压(99%)", "充电结束电压(100%)"] ("从板表头"), index=1 ("长度"), length=44 ("长度")) -> (w1466:string[])
                    n857 = for {
                      tunnel: w1476 -> [w1502] mode=indexing
                      tunnel: [w1501] -> w1475 mode=indexing
                      n858 = Fract/Exp String To Number(string=w1502) -> (number=w1501:dbl)  [unwired: 3 in, 1 out]
                    }
                    n859 = for {
                      tunnel: w1489 -> [w1504] mode=indexing
                      tunnel: [w1503] -> w1488 mode=indexing
                      n860 = Fract/Exp String To Number(string=w1504) -> (number=w1503:dbl)  [unwired: 3 in, 1 out]
                    }
                    n861 = Build Array(w1466, w1498) -> (w1497:string[][])
                    n862 = Delete From Array(array=w1475, length=7 ("长度"), index=0 ("索引")) -> (deleted portion=w1484:dbl[], array with subset deleted=w1483:dbl[])
                    n863 = Array To Cluster(array=w1488) -> (cluster=w1487:T10)
                    n864 = Transpose 2D Array(2D array=w1497) -> (transposed array=w1471:string[][])
                    n865 = local write "从板信息电压温度通道配置"(w1471) -> ()
                    n866 = Delete From Array(array=w1483, length=7 ("长度"), index=0 ("索引")) -> (deleted portion=w1480:dbl[], array with subset deleted=w1479:dbl[])
                    n867 = local write "加热控制参数 2"(w1487) -> ()
                    n868 = Build Array(w1484, w1480, w1479) -> (w1478:dbl[][])
                    n869 = Transpose 2D Array(2D array=w1478) -> (transposed array=w1477:dbl[][])
                    n870 = local write "一级故障 2"(w1477) -> ()
                  }
                  frame #2 {
                    n871 = Number To Decimal String(number=w1506) -> (decimal integer string=w1505:string)  [unwired: 1 in]
                    n872 = control-ref of="结果"() -> (w1512:refnum<vi>)
                    n873 = Concatenate Strings("从板", w1505, "导出完成") -> (w1509:string)
                    n874 = Build Array(w1509) -> (w1507:string[])
                    n875 = call "表格编辑.vi"("新元素/子数组"=w1507, "活动单元格:单元格背景色"=u32 6618880, "MCListbox引用句柄"=w1512) -> ()  [unwired: 9 in]
                  }
                }
              }
            }
          }
          frame True {
          }
        }
      }
      event "退出": Value Change {
        n876 = event-data() -> ()  [unwired: 1 in, 6 out]
        n877 = global read "配置文件全局.vi" "参数生成器读取地址"() -> (w1517:path)
        n878 = call <vilib>:"Application Directory.vi"() -> ("Application Directory"=w1523:path)
        n879 = Build Path(base path=w1523, name or relative path="config.ini" ("名称或相对路径")) -> (appended path=w1521:path)
        n880 = call <vilib>:"Open Config Data.vi"("configuration file path"=w1521) -> ("error out"=w1516:errorcluster, "refnum"=w1520:T11)  [unwired: 8 in, 1 out]
        n881 = call-poly <vilib>:"Write Key.vi"("section"="总信息", "error in (no error)"=w1516, "value"=w1517, "key"="参数生成器读取地址" ("section"), "refnum"=w1520) -> ("error out"=w1515:errorcluster, "refnum out"=w1514:T11)  [unwired: 4 in, 1 out]
        n882 = call <vilib>:"Close Config Data.vi"("error in (no error)"=w1515, "refnum"=w1514) -> ("error out"=w1513:errorcluster)  [unwired: 8 in, 1 out]
        n883 = call <vilib>:"Clear Errors.vi"("error in (no error)"=w1513) -> ()  [unwired: 6 in, 1 out]
      }
      event Panel Close? {
        n884 = event-data() -> ()  [unwired: 1 in, 4 out]
        n885 = global read "配置文件全局.vi" "参数生成器读取地址"() -> (w1529:path)
        n886 = call <vilib>:"Application Directory.vi"() -> ("Application Directory"=w1535:path)
        n887 = Build Path(base path=w1535, name or relative path="config.ini" ("名称或相对路径")) -> (appended path=w1533:path)
        n888 = call <vilib>:"Open Config Data.vi"("configuration file path"=w1533) -> ("error out"=w1528:errorcluster, "refnum"=w1532:T11)  [unwired: 8 in, 1 out]
        n889 = call-poly <vilib>:"Write Key.vi"("section"="总信息", "error in (no error)"=w1528, "value"=w1529, "key"="参数生成器读取地址" ("section"), "refnum"=w1532) -> ("error out"=w1527:errorcluster, "refnum out"=w1526:T11)  [unwired: 4 in, 1 out]
        n890 = call <vilib>:"Close Config Data.vi"("error in (no error)"=w1527, "refnum"=w1526) -> ("error out"=w1525:errorcluster)  [unwired: 8 in, 1 out]
        n891 = call <vilib>:"Clear Errors.vi"("error in (no error)"=w1525) -> ()  [unwired: 6 in, 1 out]
        n892 = event-data("Discard?"=FALSE ("放弃？")) -> ()  [unwired: 1 in, 1 out]
      }
      event Timeout {
        n893 = event-data() -> ()  [unwired: 1 in, 3 out]
        n894 = local read "从板个数"() -> (w1540:dbl)
        n895 = control-ref of="从板板号"() -> (w1541:refnum<vi>)
        n896 = property class="DigNum (严格)"(reference=w1541, "Maximum"=w1540, "Minimum"=1.0 ("数据输入界限:最小值")) -> ()  [unwired: 1 in, 2 out]
        n897 = case shown="假" FALSE {
          frame False {
          }
          frame True {
            n898 = local read "从板信息电压温度通道配置"() -> (w1565:string[][])
            n899 = local read "加热控制参数 2"() -> (w1564:T3)
            n900 = local read "一级故障 2"() -> (w1562:dbl[][])
            n901 = Transpose 2D Array(2D array=w1562) -> (transposed array=w1551:dbl[][])
            n902 = Cluster To Array(cluster=w1564) -> (array=w1563:dbl[])
            n903 = local read "均衡参数"() -> (w1545:T1)
            n904 = Array Subset(array=w1565, index (row)=0 ("索引"), index (col)=0 ("索引"), length (col)=2 ("索引")) -> (w1560:string[][])  [unwired: 1 in]
            n905 = for {
              tunnel: w1551 -> [w1577] mode=indexing
              shift-right: [w1576] -> w1558
              shift-left: string[] [] -> [w1574]
              n906 = for {
                N: 7 -> [_]
                tunnel: w1577 -> [w1580] mode=indexing
                tunnel: [w1578] -> w1575 mode=indexing
                n907 = Format Into String(format string="%#f" ("格式字符串"), w1580) -> (resulting string=w1578:string)  [unwired: 2 in, 1 out]
              }
              n908 = Insert Into Array(array=w1574, new element=w1575) -> (w1576:string[])  [unwired: 1 in]
            }
            n909 = Index Array(array=w1560, index (col) #2=1 ("索引 (列)")) -> (element #2=w1548:string[])  [unwired: 3 in, 1 out]
            n910 = for {
              tunnel: w1563 -> [w1583] mode=indexing
              tunnel: [w1581] -> w1559 mode=indexing
              n911 = Format Into String(format string="%#f" ("格式字符串"), w1583) -> (resulting string=w1581:string)  [unwired: 2 in, 1 out]
            }
            n912 = Cluster To Array(cluster=w1545) -> (array=w1544:sgl[])
            n913 = for {
              tunnel: w1544 -> [w1572] mode=indexing
              tunnel: [w1570] -> w1543 mode=indexing
              n914 = Format Into String(format string="%#f" ("格式字符串"), w1572) -> (resulting string=w1570:string)  [unwired: 2 in, 1 out]
            }
            n915 = local read "从板板号"() -> (w1554:dbl)
            n916 = Array Subset(array=w1548, length=28 ("长度")) -> (w1549:string[])  [unwired: 1 in]
            n917 = Number To Decimal String(number=w1554) -> (decimal integer string=w1553:string)  [unwired: 1 in]
            n918 = Insert Into Array(array=w1549, new element #1=w1559, new element #2=w1558, new element #3=w1543) -> (w1557:string[])  [unwired: 1 in]
            n919 = Decrement(x=w1554) -> (x-1=w1550:dbl)
            n920 = local read "输出数组"() -> (w1569:string[][])
            n921 = Insert Into Array(array=w1557, index=0 ("索引"), new element=w1553) -> (w1555:string[])
            n922 = Replace Array Subset(array=w1569, new element=w1555, index (col)=w1550) -> (w1542:string[][])  [unwired: 1 in]
            n923 = local write "从板表头"(string[] ["从板板号", "电压个数", "温度个数", "第一个保险通道", "第一个保险位置", "第二个保险通道", "第二个保险位置", "第三个保险通道", "第三个保险位置", "第四个保险通道", "第四个保险位置", "第五个保险通道", "第五个保险位置", "第六个保险通道", "第六个保险位置", "第七个保险通道", "第七个保险位置", "第八个保险通道", "第八个保险位置", "第九个保险通道", "第九个保险位置", "第十个保险通道", "第十个保险位置", "第1通道电压个数", "第2通道电压个数", "第3通道电压个数", "第4通道电压个数", "第5通道电压个数", "风机开启温度", "风机关闭温度", "加热开启温度", "加热关闭温度", "风机开启温差", "风机关闭温差", "加热关闭温差", "电压过高一级", "电压过低一级", "温度过高一级", "温度过低一级", "电压不均衡一级", "温度不均衡一级", "SOC过低一级", "电压过高二级", "电压过低二级", "温度过高二级", "温度过低二级", "电压不均衡二级", "温度不均衡二级", "SOC过低二级", "电压过高三级", "电压过低三级", "温度过高三级", "温度过低三级", "电压不均衡三级", "温度不均衡三级", "SOC过低三级", "均衡计算-电压高阀值1级", "均衡计算-电压高阀值2级", "均衡计算-电压低阀值1级", "均衡计算-电压低阀值2级", "均衡计算-最低电压阀值", "均衡停止-最低电压阀值", "均衡计算-电压极差阀值", "充电结束电压(90%)", "充电结束电压(91%)", "充电结束电压(92%)", "充电结束电压(93%)", "充电结束电压(94%)", "充电结束电压(95%)", "充电结束电压(96%)", "充电结束电压(97%)", "充电结束电压(98%)", "充电结束电压(99%)", "充电结束电压(100%)"] ("从板表头")) -> ()
            n924 = local write "输出数组"(w1542) -> ()
          }
        }
      }
      event Value Change {
        n925 = event-data() -> ("NewVal"=w1584:T5)  [unwired: 1 in, 5 out]
        n926 = case shown="真" w1584 {
          frame False {
          }
          frame True {
            n927 = local read "从板板号"() -> (w1587:dbl)
            n928 = local read "输出数组"() -> (w1588:string[][])
            n929 = Decrement(x=w1587) -> (x-1=w1586:dbl)
            n930 = Index Array(array=w1588, index (col)=w1586) -> (element=w1585:string[])  [unwired: 1 in]
            n931 = local write "临时从板数据"(w1585) -> ()
          }
        }
      }
      event "粘贴": Value Change {
        n932 = event-data() -> ("NewVal"=w1589:bool)  [unwired: 1 in, 5 out]
        n933 = case shown="真" w1589 {
          frame False {
          }
          frame True {
            n934 = local read "临时从板数据"() -> (w1593:string[])
            n935 = local read "从板板号"() -> (w1594:dbl)
            n936 = local read "输出数组"() -> (w1597:string[][])
            n937 = Decrement(x=w1594) -> (x-1=w1595:dbl)
            n938 = Number To Decimal String(number=w1594) -> (decimal integer string=w1591:string)  [unwired: 1 in]
            n939 = Replace Array Subset(array=w1593, new element=w1591, index=0 ("索引")) -> (w1590:string[])
            n940 = Replace Array Subset(array=w1597, new element=w1590, index (col)=w1595) -> (w1596:string[][])  [unwired: 1 in]
            n941 = local write "输出数组"(w1596) -> ()
            n942 = stacked-sequence {
              tunnel: w1591 -> [w1602]
              frame #0 {
                n943 = control-ref of="结果"() -> (w1604:refnum<vi>)
                n944 = Concatenate Strings("从板", w1602, "粘贴并保存成功") -> (w1600:string)
                n945 = Build Array(w1600) -> (w1598:string[])
                n946 = call "表格编辑.vi"("新元素/子数组"=w1598, "活动单元格:单元格背景色"=u32 6618880, "MCListbox引用句柄"=w1604) -> ()  [unwired: 9 in]
              }
            }
          }
        }
      }
    }
  }
  n947 = stacked-sequence {
    frame #0 {
      w1606 = FALSE ("主页按钮")
      n948 = global read "功能码全局.vi" "主板监控2"() -> (w1608:bool[])
      n949 = control-ref of="单选选项2"() -> (w1615:refnum<vi>)
      n950 = control-ref of="单选选项1"() -> (w1614:refnum<vi>)
      n951 = Build Array(w1614, w1615) -> (w1616:refnum<vi>[])
      n952 = Index Array(array=w1608, index #1=6 ("索引"), index #2=7 ("索引")) -> (element #1=w1610:bool, element #2=w1612:bool)
      n953 = Delete From Array(array=w1616, index=1 ("索引")) -> (deleted portion=w1618:refnum<vi>, array with subset deleted=w1617:refnum<vi>[])  [unwired: 1 in]
      n954 = property on="写配置文件" class="Bool (严格)"("Visible"=w1610) -> ()  [unwired: 2 in, 2 out]
      n955 = property on="读取(ini)" class="Bool (严格)"("Visible"=w1612) -> ()  [unwired: 2 in, 2 out]
      n956 = property on="预览" class="Bool (严格)"("Visible"=w1612) -> ()  [unwired: 2 in, 2 out]
      n957 = property class="Bool (严格)"(reference=w1618, "BoolText.TextColor"=u32 16448250) -> ()  [unwired: 1 in, 2 out]
      n958 = for {
        tunnel: u32 8977151 -> [w1629]
        tunnel: w1617 -> [w1628] mode=indexing
        n959 = property class="Bool (严格)"(reference=w1628, "BoolText.TextColor"=w1629) -> ()  [unwired: 1 in, 2 out]
      }
      n960 = local write "选项卡控件"(enum32{"主板", "从板", "预览"}."主板" ("选项卡控件")) -> ()
      n961 = local write "主从板"(enum32{"单选选项2", "单选选项1"}."单选选项1" ("主从板")) -> ()
      n962 = local write "均衡参数"(T1 {"充电结束电压(90%)"=3.0, "充电结束电压(91%)"=3.0, "充电结束电压(92%)"=3.0, "充电结束电压(93%)"=3.0, "充电结束电压(94%)"=3.0, "均衡计算-电压高阀值1级"=3.0, "均衡计算-电压高阀值2级"=3.0, "均衡计算-电压低阀值1级"=3.0, "均衡计算-电压低阀值2级"=3.0, "均衡计算-最低电压阀值"=3.0, "均衡停止-最低电压阀值"=3.0, "均衡计算-电压极差阀值"=3.0, "充电结束电压(95%)"=3.0, "充电结束电压(96%)"=3.0, "充电结束电压(97%)"=3.0, "充电结束电压(98%)"=3.0, "充电结束电压(99%)"=3.0, "充电结束电压(100%)"=3.0} ("均衡参数")) -> ()
      n963 = local write "从板表头"(string[] [] ("key names")) -> ()
      n964 = control-ref of="结果"() -> (w1626:refnum<vi>)
      n965 = for {
        N: 40 -> [_]
        tunnel: w1626 -> [w1637]
        i -> [w1635]
        n966 = Bundle(w1635, 0) -> (w1633:cluster{i32, i32})  [unwired: 1 out]
        n967 = property class="MCListbox (严格)"(reference=w1637, "ActiveCell"=w1633, "CellBG"=u32 16448250) -> ()  [unwired: 1 in, 2 out]
      }
      n968 = property class="MCListbox (严格)"(reference=w1626, "ItemNames"=string[][] [] ("项名")) -> ()  [unwired: 1 in, 2 out]
      n969 = for {
        N: 100 -> [_]
        tunnel: [w1631] -> w1623 mode=indexing
        n970 = for {
          N: 30 -> [_]
          tunnel: [" "] -> w1631 mode=indexing
        }
      }
      n971 = local write "读主板参数"(w1606) -> ()
      n972 = local write "写配置文件"(w1606) -> ()
      n973 = local write "读从板参数"(w1606) -> ()
      n974 = local write "读取(ini)"(w1606) -> ()
      n975 = local write "预览"(w1606) -> ()
      n976 = local write "退出"(w1606) -> ()
      n977 = local write "输出数组"(w1623) -> ()
      n978 = local write "自动记录"(w1606) -> ()
      n979 = local write "布尔"(w1606) -> ()
      n980 = property on="查看" class="Bool (严格)"("Visible"=w1606) -> ()  [unwired: 2 in, 2 out]
      n981 = call "自适应屏幕分辨率.vi"() -> ()  [unwired: 16 in]
    }
  }
